vi "Main.vi"() -> ()   [LabVIEW 2013]
doc: "Use this template to build a producer/consumer design pattern with events to produce queue items. Use this design pattern instead of the User Interface Event Handler pattern for user interfaces when you want to execute code asynchronously in response to an event without slowing the user interface responsiveness."
uses:
  ControlLib.llb/state_cntrl.ctl
  ControlLib.llb/main_clstr.ctl
  ControlLib.llb/main_cons_loop_clstr.ctl
  ControlLib.llb/res_range_type_cntrl.ctl
panel:
  out "array":dbl[][](array[numeric])
  out "state_ind":T1=enum."idle" caption="State Status"
  in  "Tab Control":T2(tab)
  in  "initialize":bool caption="Clear All Flags"
  out "stat_oper_resp":string caption="Status Operation Cond Resp"
  in  "stat_oper_cond":bool caption="Check Status Oper Cond"
  in  "trig_dely_auto":bool=TRUE
  in  "trig_delay":dbl caption="Trigger Delay (s)"
  in  "smpl_cnt":u32=1 caption="Sample Count" min=1 max=500000 step=1
  in  "trig_timer_val":dbl caption="Trig Timer Value (s)" max=359999.0 format="%#_2e"
  in  "no_of_trig":u32=1 caption="No of Trigger" max=500000 step=1
  in  "max_trig_cnt":enum16{"Specify Count", "Infinity"}(ring) caption="Max Trig Cnt"
  in  "trig_src":T3(ring)=enum."Immediate" caption="Trigger Source"
  in  "conf_trig":bool caption="Config Trigger"
  out "Error Message":string
  in  "err_qry":bool caption="Error Query"
  in  "fetch_numbers":bool
  in  "byte_count":i32=1024
  out "scan_data":string[](array[string]) caption="Scan Data"
  in  "fetch":bool caption="Fetch Data"
  in  "init":bool caption="Initialize Trigger"
  in  "scan":bool caption="Start Scan"
  in  "range":T4(ring)=enum."Auto" caption="Range"
  in  "res":T5(ring)=enum."6 1/2" caption="Resolution"
  in  "off_comp":bool
  in  "conf_4_wire":bool caption="4 Wire Config"
  in  "open_ch":bool caption="Open Channel"
  in  "chk_ch_state":bool caption="Check channel state?"
  out "ch_state?":string caption="State of the channel"
  in  "VISA resource name":refnum<visa-resource-name>
  in  "close_ch":bool caption="Close Channel"
  in  "ch_string":string caption="Channel or ABUS"
  in  "res_path":path caption="Resistance Path"
  out "res_table":string[][](table) caption="Resistance Table"
  in  "start":bool
  out "text_file":string caption="Data File"
  out "ch_list_str":string caption="Channels Being Scan"
  in  "stop":bool
  # "JPL Automated Multiplexer Safe To Mate - June 2017"
  # "To measure the resistances:\n\n1.  Upload a channel list file.\n2.  Press START to scan.\n3.  The START button will depress\n      itself when the scanning is done."
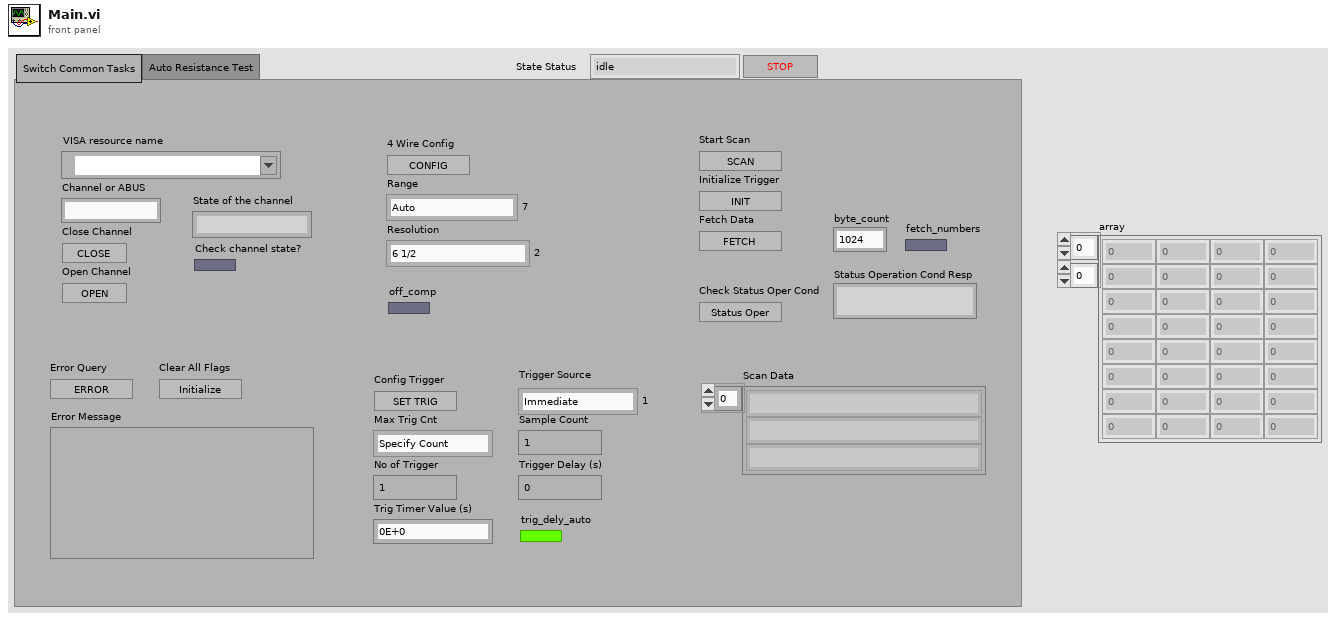
[diagram p1: front panel]
types:
  T1 = typedef "state_cntrl.ctl" = enum16{"initialize", "idle", "read_res_col", "res_val_qry", "plc_ch_in_100_list", "plc_ch_in_1K_list", "plc_ch_in_10K_list", "plc_ch_in_100K_list", "plc_ch_in_1M_list", "plc_ch_in_10M_list", "plc_ch_in_100M_list", "set_100_list_flg", "set_1K_list_flg", "set_10K_list_flg", "set_100K_list_flg", "set_1M_list_flg", "set_10M_list_flg", "set_100M_list_flg", "fin_arry_qry", "chk_100_list_flg", "chk_1K_list_flg", "chk_10K_list_flg", "chk_100K_list_flg", "chk_1M_list_flg", "chk_10M_list_flg", "chk_100M_list_flg", "set_100_ohm_chnl_list", "set_1K_ohm_chnl_list", "set_10K_ohm_chnl_list", "set_100K_ohm_chnl_list", "set_1M_ohm_chnl_list", "set_10M_ohm_chnl_list", "set_100M_ohm_chnl_list", "place_res_in_range", "eof", "det_rnge_to_meas", "set_ch_list", "conf_wire_mode", "conf_trig_type", "start_scan", "scan_cancel_qry", "init_meas", "done_meas_qry", "fetch_data", "fin_test_qry", "fill_data_table", "disp_results"}
  T2 = enum32{"Switch Common Tasks", "Auto Resistance Test"}
  T3 = enum16{"Bus", "Immediate", "External", "Alarm 1", "Alarm 2", "Alarm 3", "Alarm 4", "Timer"}
  T4 = enum16{"100 Ohm", "1 kOhm", "10 kOhm", "100 kOhm", "1 MOhm", "10 MOhm", "100 MOhm", "Auto", "Minimum", "Maximum", "Default"}
  T5 = enum16{"4 1/2", "5 1/2", "6 1/2", "Least", "Highest", "Default"}
  T6 = typedef "main_clstr.ctl" = cluster{"state":T1, "res_col_cnt":i32}
  T7 = typedef "main_cons_loop_clstr.ctl" = cluster{"state":T1, "res_row_cnt":i32, "res_col":dbl[], "res_range_type":T8, "chnl_col":dbl[], "range_setting":bool[], "first_time_set":bool[], "100_list_ch":dbl[], "100_list_row_cnt":i32, "1K_list_ch":dbl[], "1K_list_row_cnt":i32, "10K_list_ch":dbl[], "10K_list_row_cnt":i32, "100K_list_ch":dbl[], "100K_list_row_cnt":i32, "1M_list_ch":dbl[], "1M_list_row_cnt":i32, "10M_list_ch":dbl[], "10M_list_row_cnt":i32, "100M_list_ch":dbl[], "100M_list_row_cnt":i32, "list_flag":bool[], "ch_list_set_cnt":i32, "res_tot_cnt":i32, "slot_col":dbl[], "ch_list_indx_100":i32[], "ch_list_indx_1K":i32[], "ch_list_indx_10K":i32[], "ch_list_indx_100K":i32[], "ch_list_indx_1M":i32[], "ch_list_indx_10M":i32[], "ch_list_indx_100M":i32[], "res_table":dbl[][], "100_ch_list_str":string, "1K_ch_list_str":string, "10K_ch_list_str":string, "100K_ch_list_str":string, "1M_ch_list_str":string, "10M_ch_list_str":string, "100M_ch_list_str":string, "range":enum16{"100 Ohm", "1 kOhm", "10 kOhm", "100 kOhm", "1 MOhm", "10 MOhm", "100 MOhm", "Auto", "Minimum", "Maximum", "Default"}, "resolution":enum16{"4 1/2", "5 1/2", "6 1/2", "Least", "Highest", "Default"}, "scan_data":string[], "res_table_text":string[][]}
  T8 = typedef "res_range_type_cntrl.ctl" = enum16{"100", "1K", "10K", "100K", "1M", "10M", "100M"}
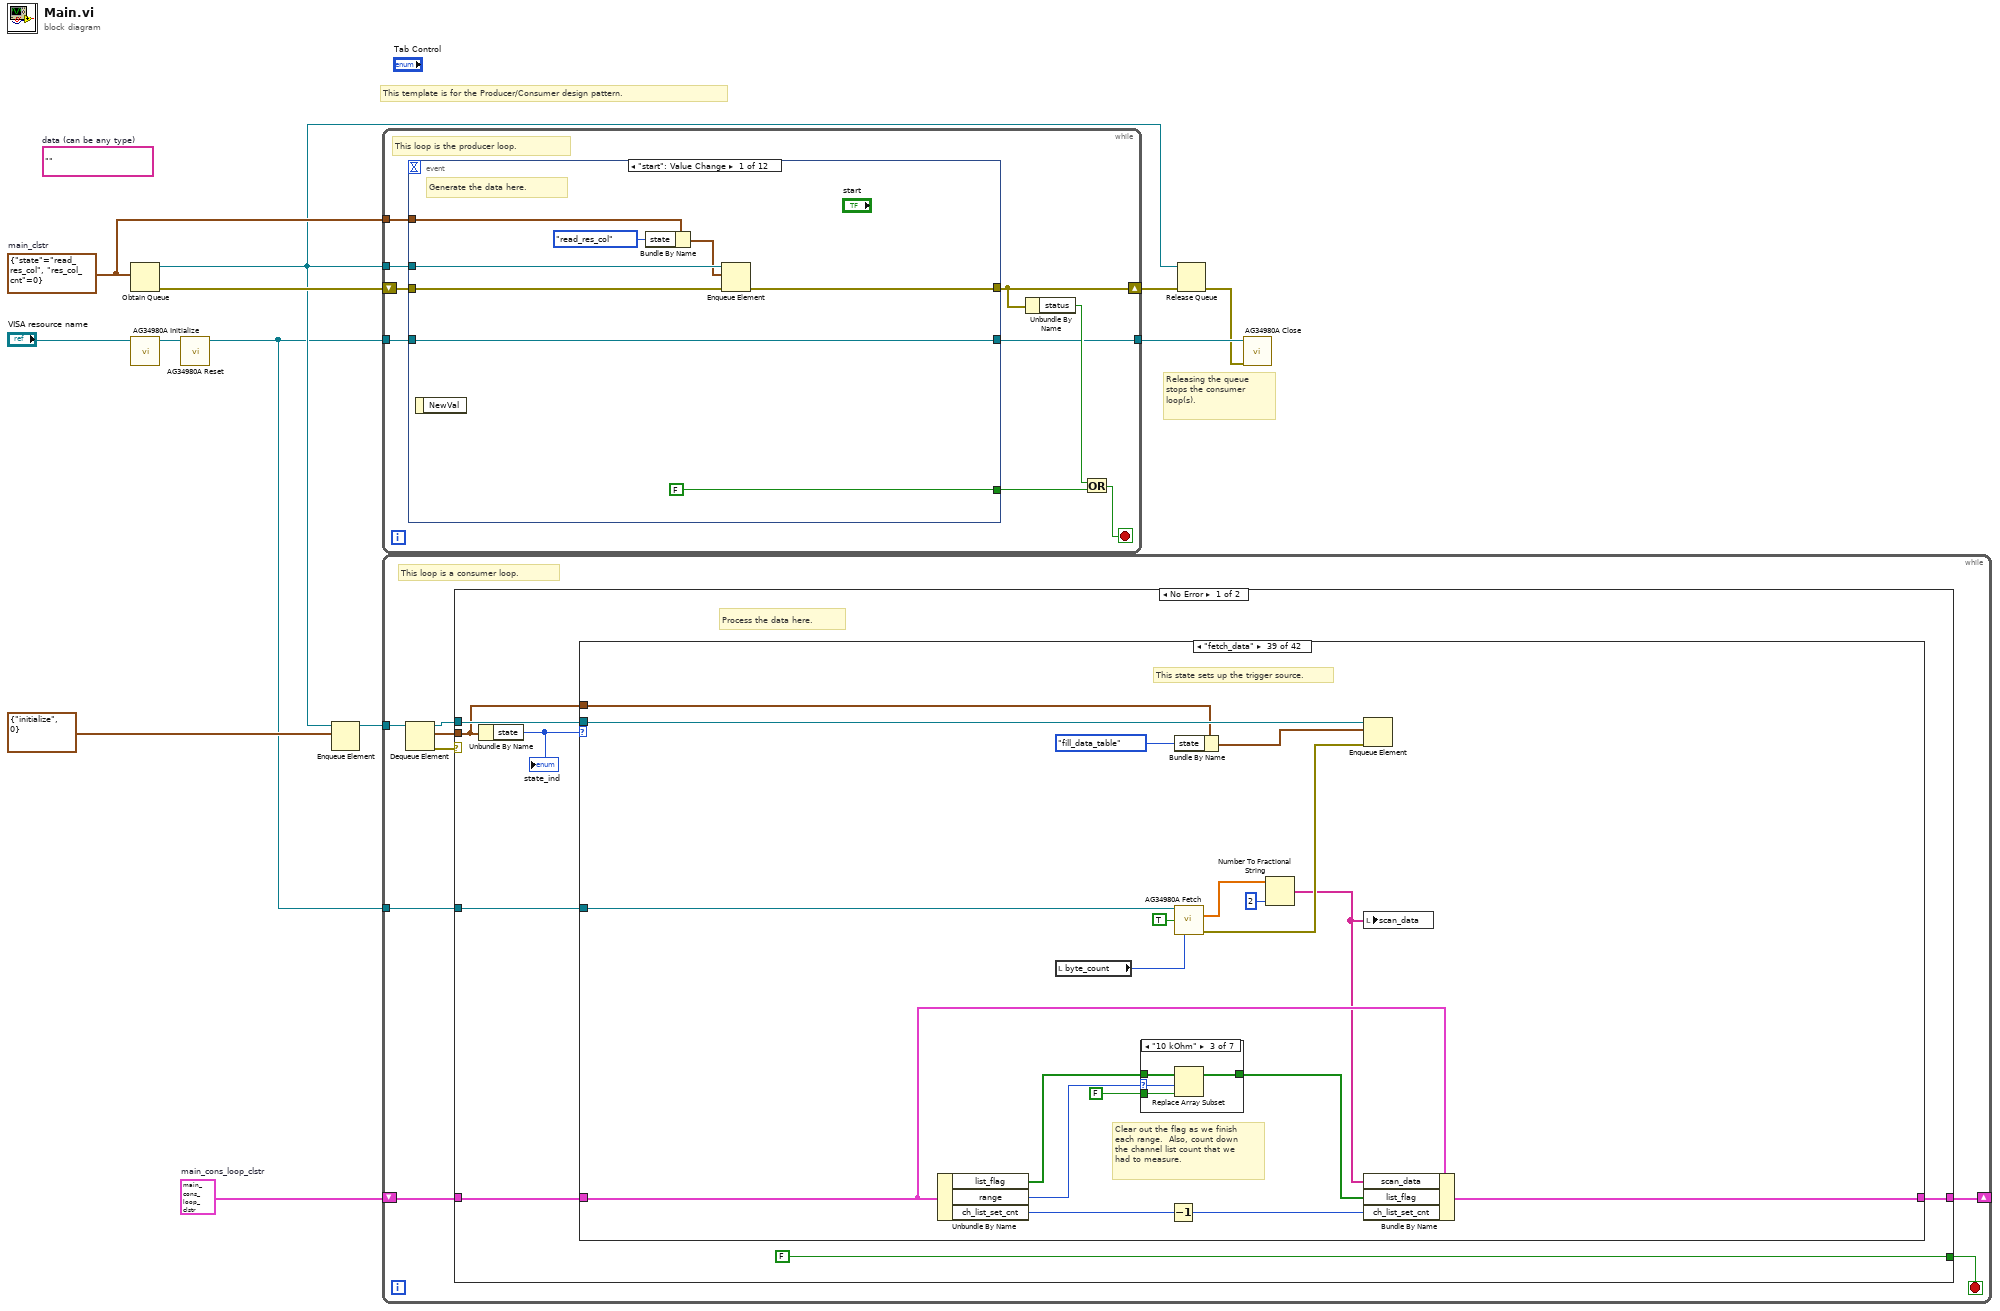
[diagram p0: block diagram]
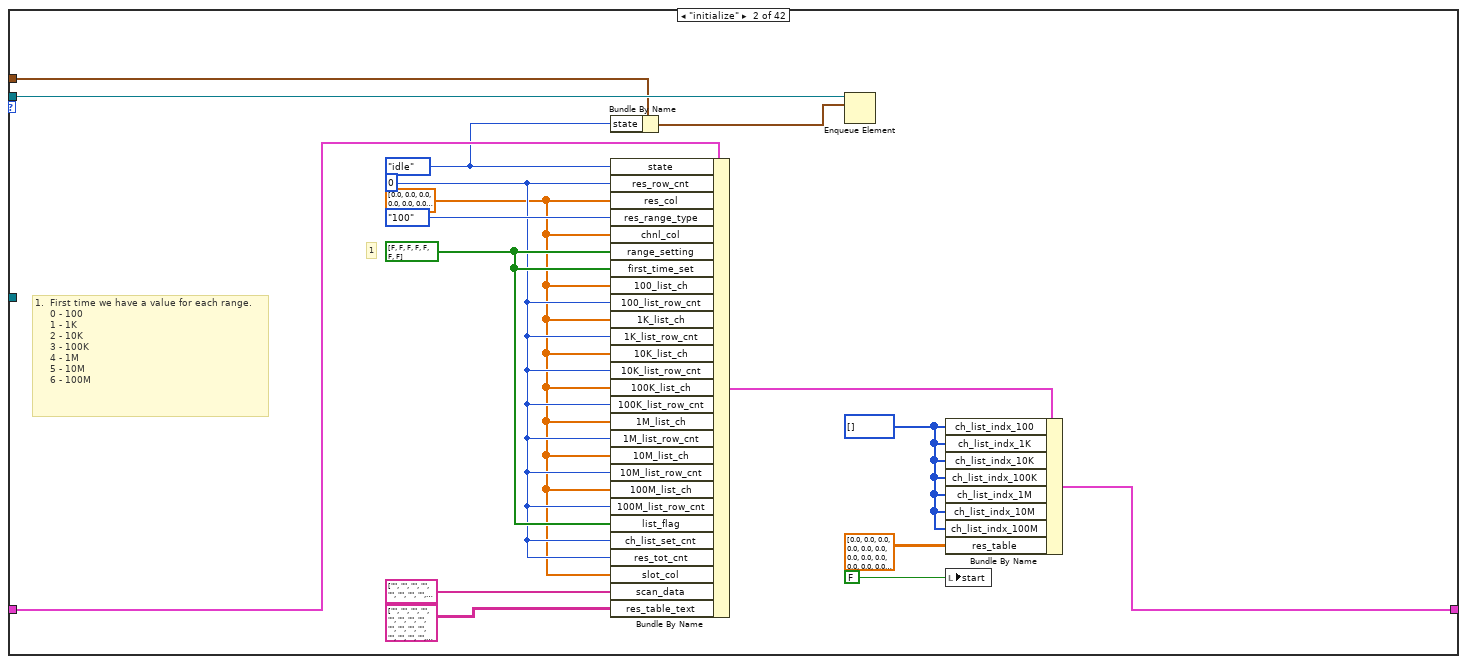
[diagram p3: hidden frame]
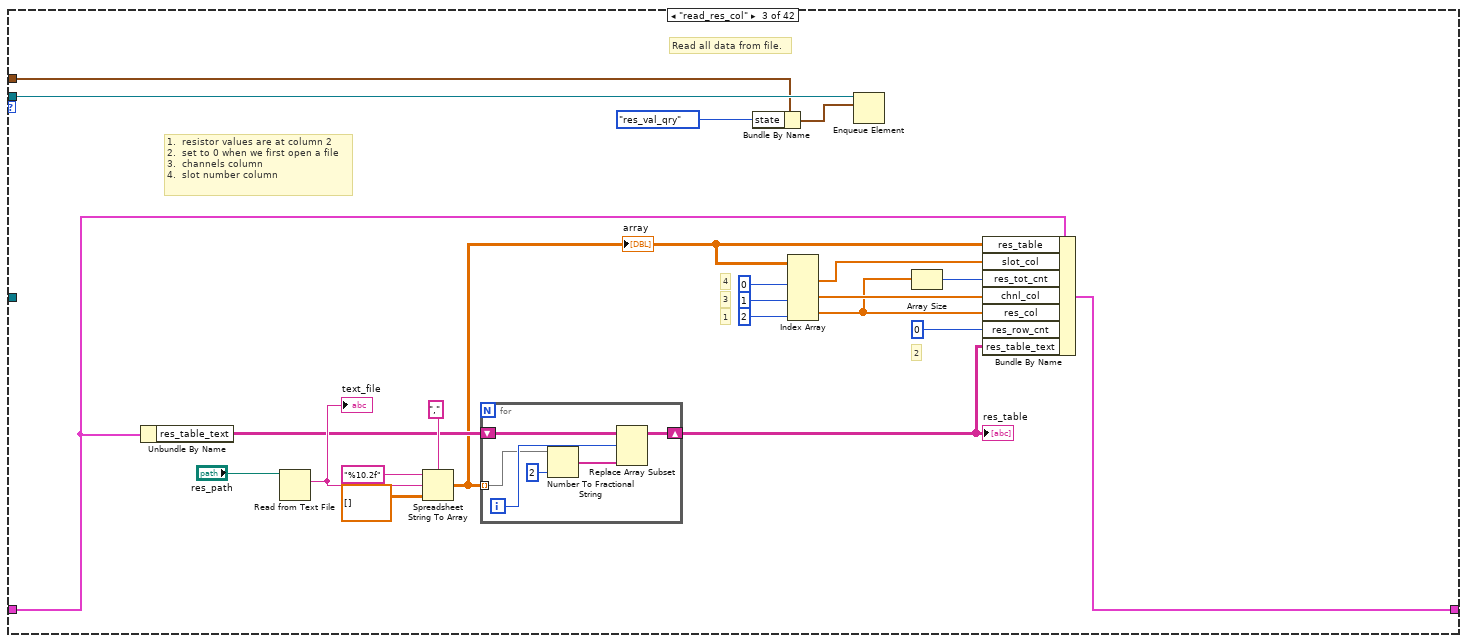
[diagram p4: hidden frame]
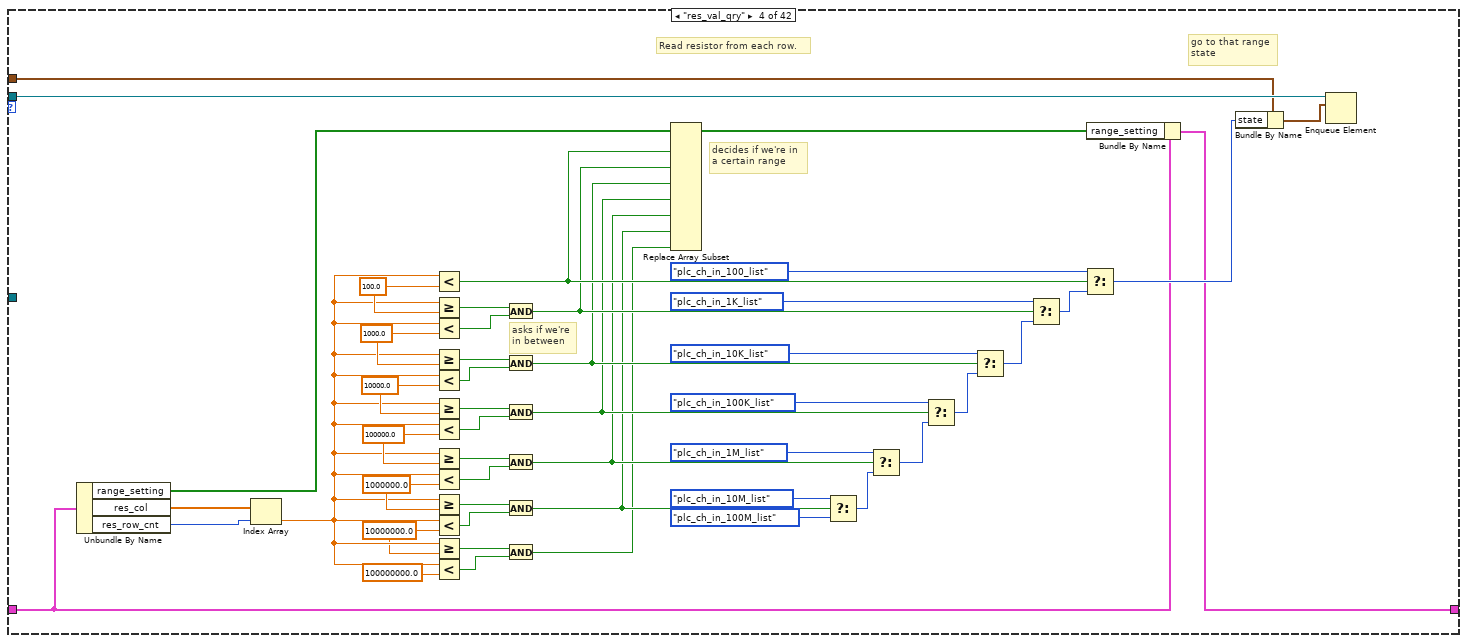
[diagram p5: hidden frame]
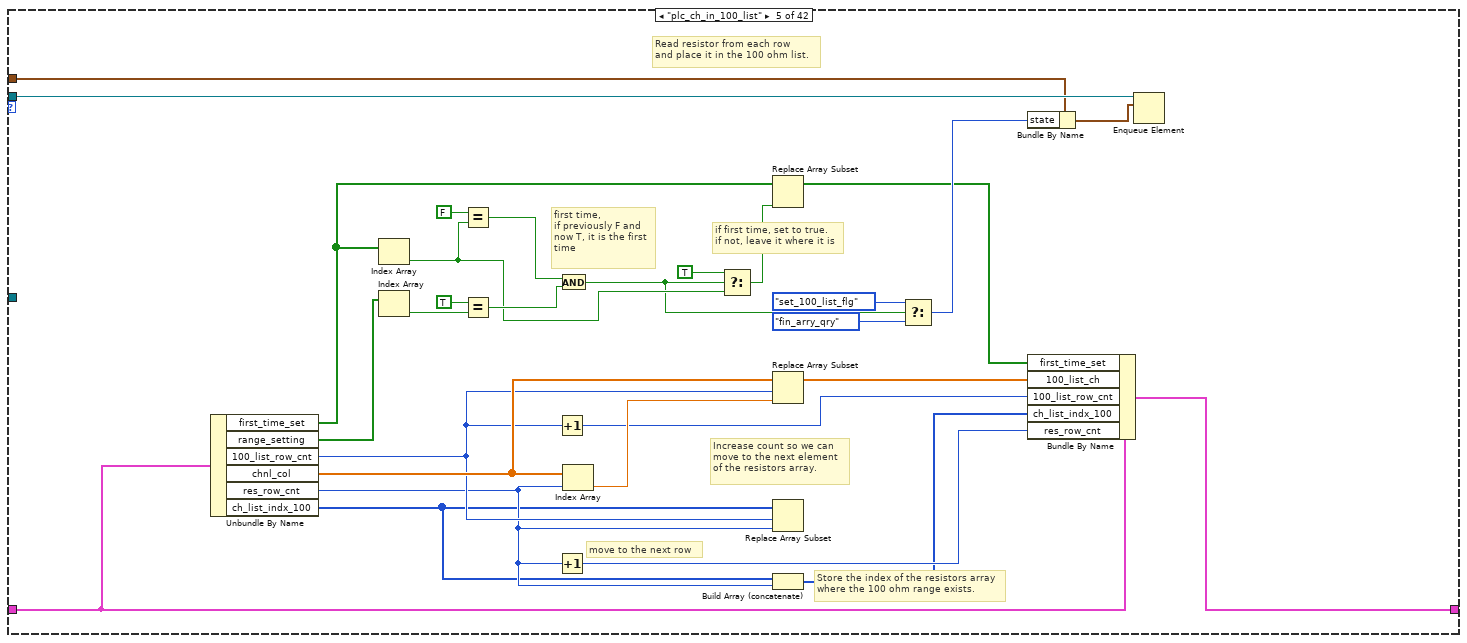
[diagram p6: hidden frame]
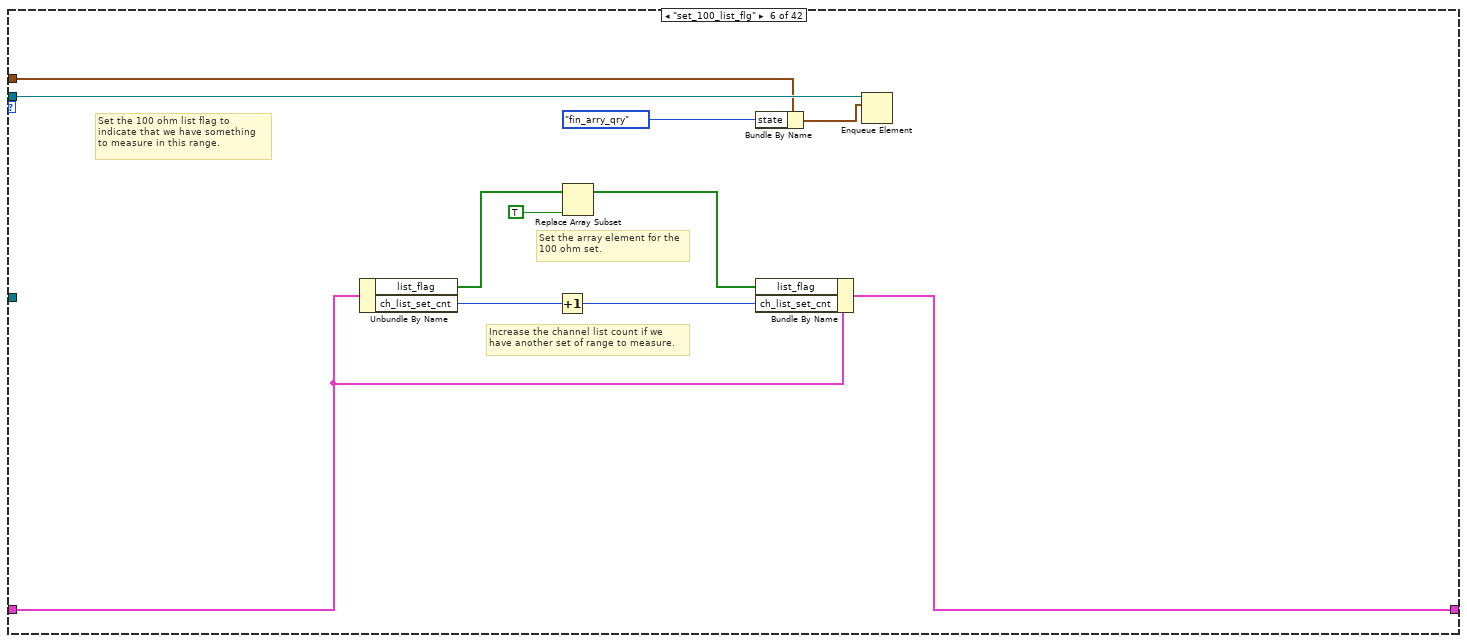
[diagram p7: hidden frame]
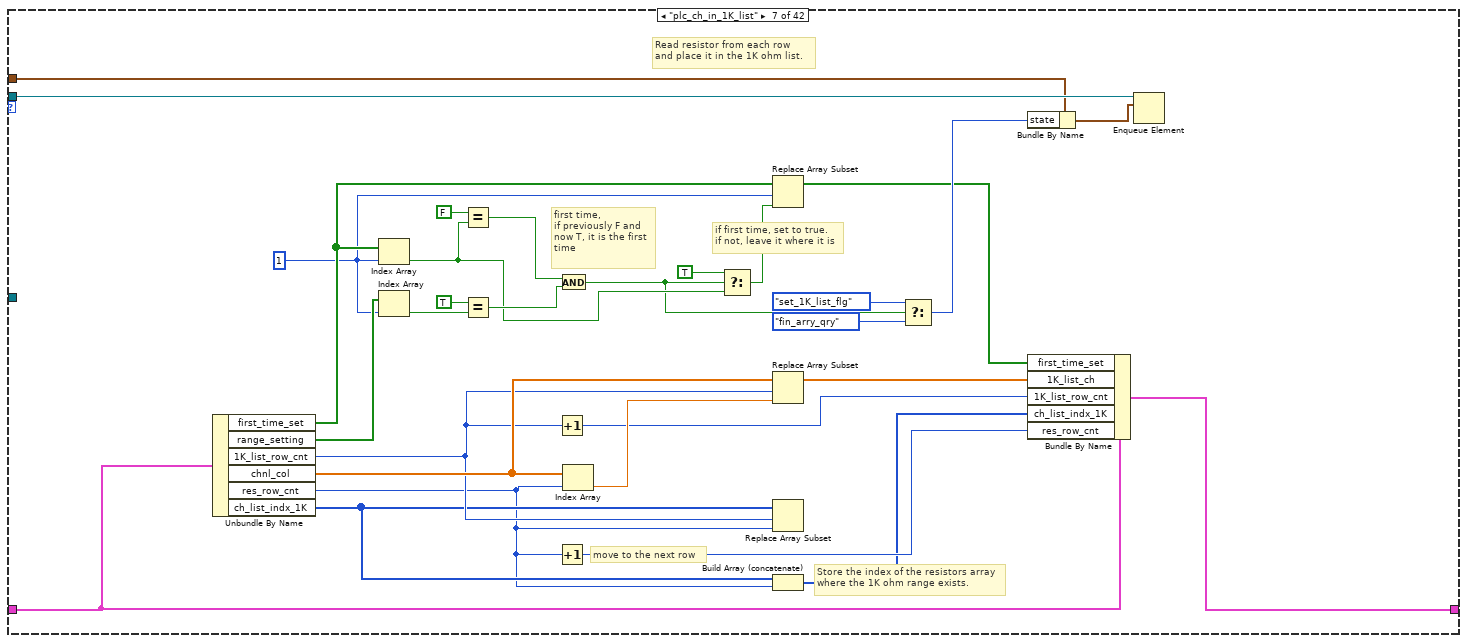
[diagram p8: hidden frame]
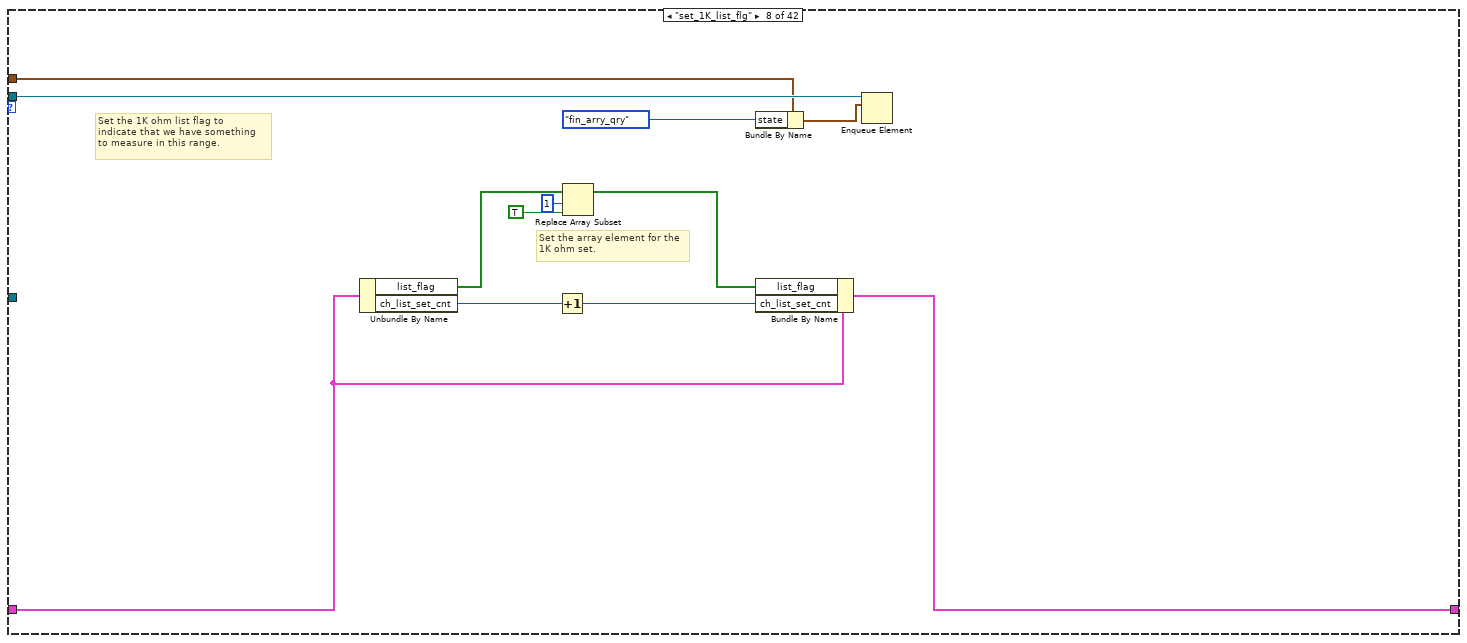
[diagram p9: hidden frame]
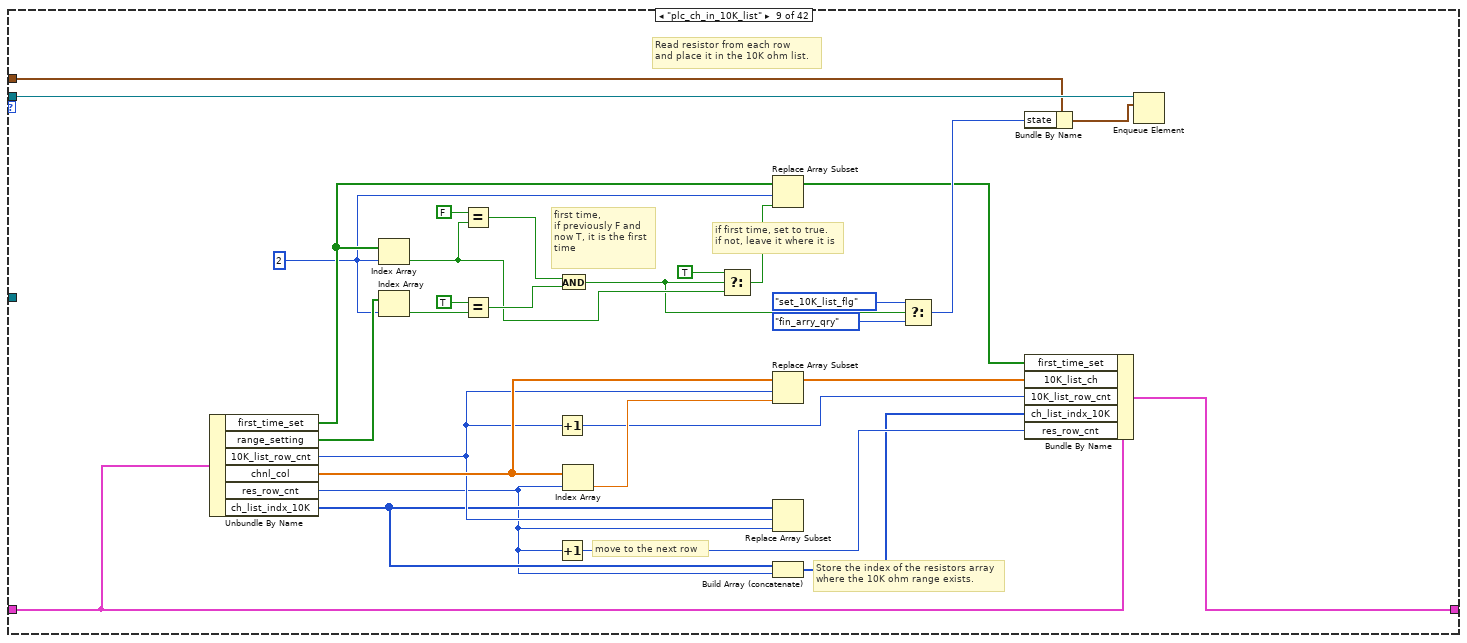
[diagram p10: hidden frame]
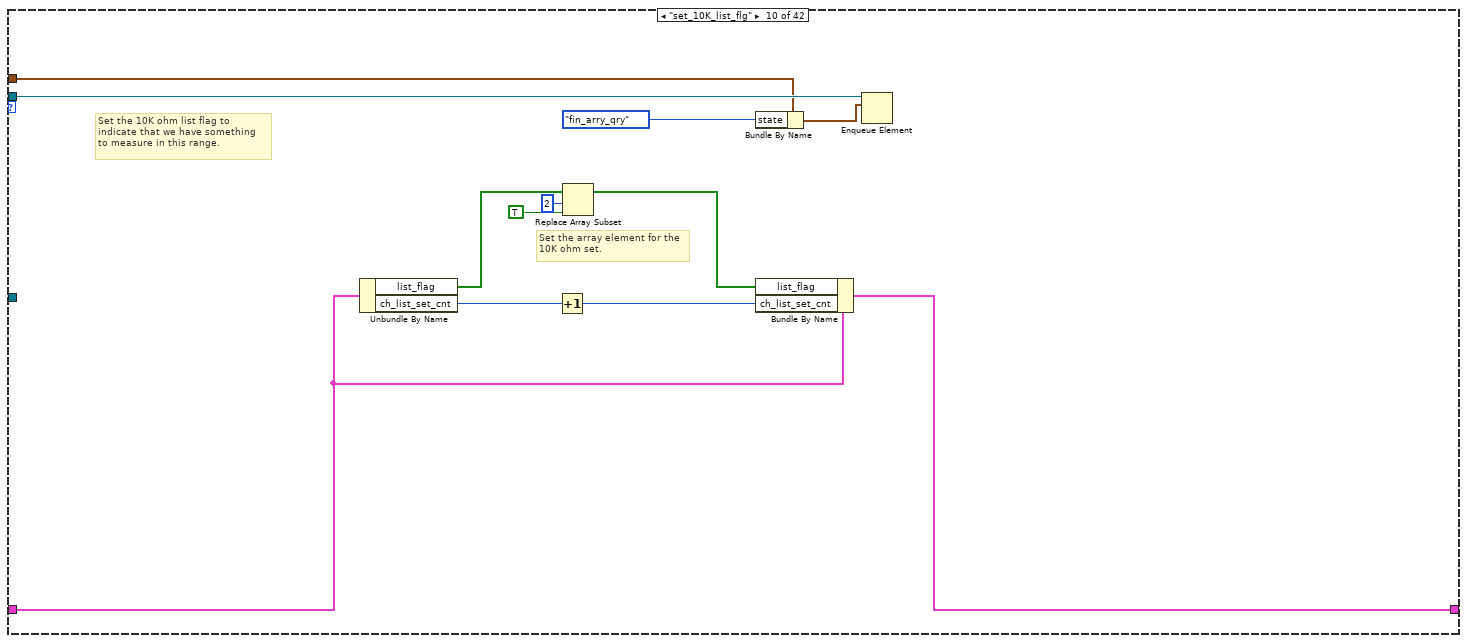
[diagram p11: hidden frame]
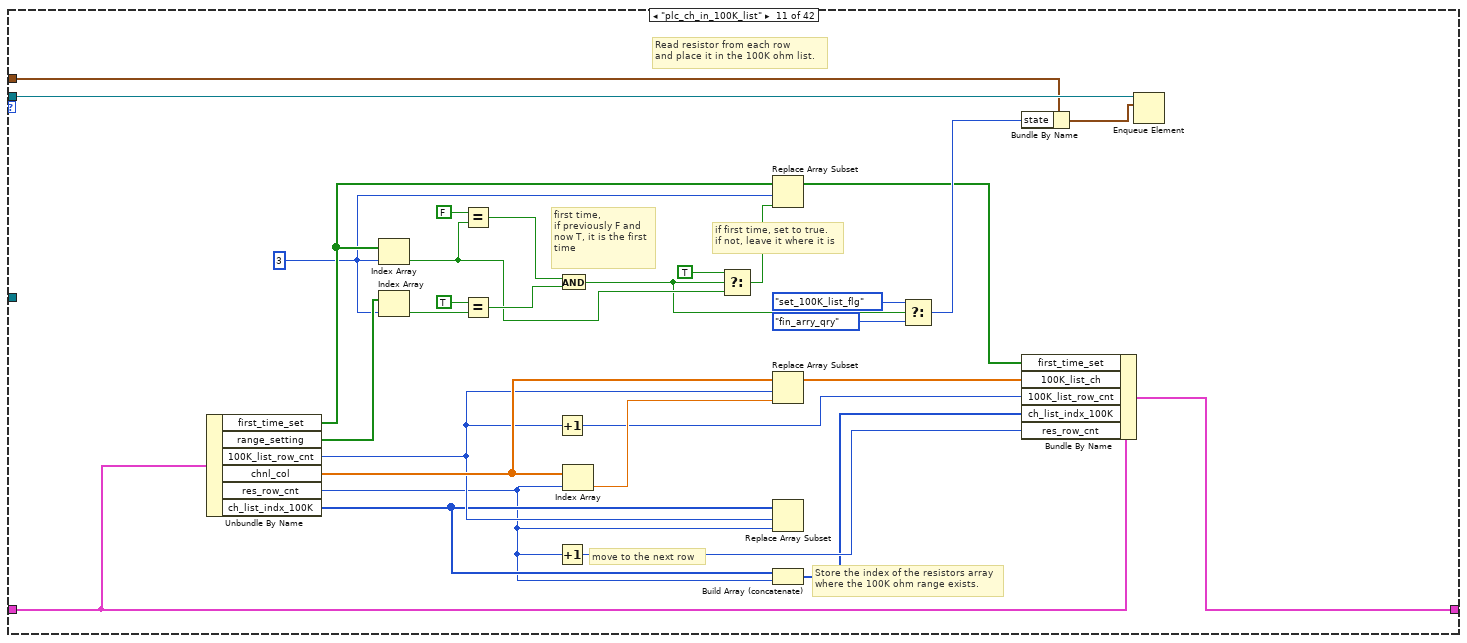
[diagram p12: hidden frame]
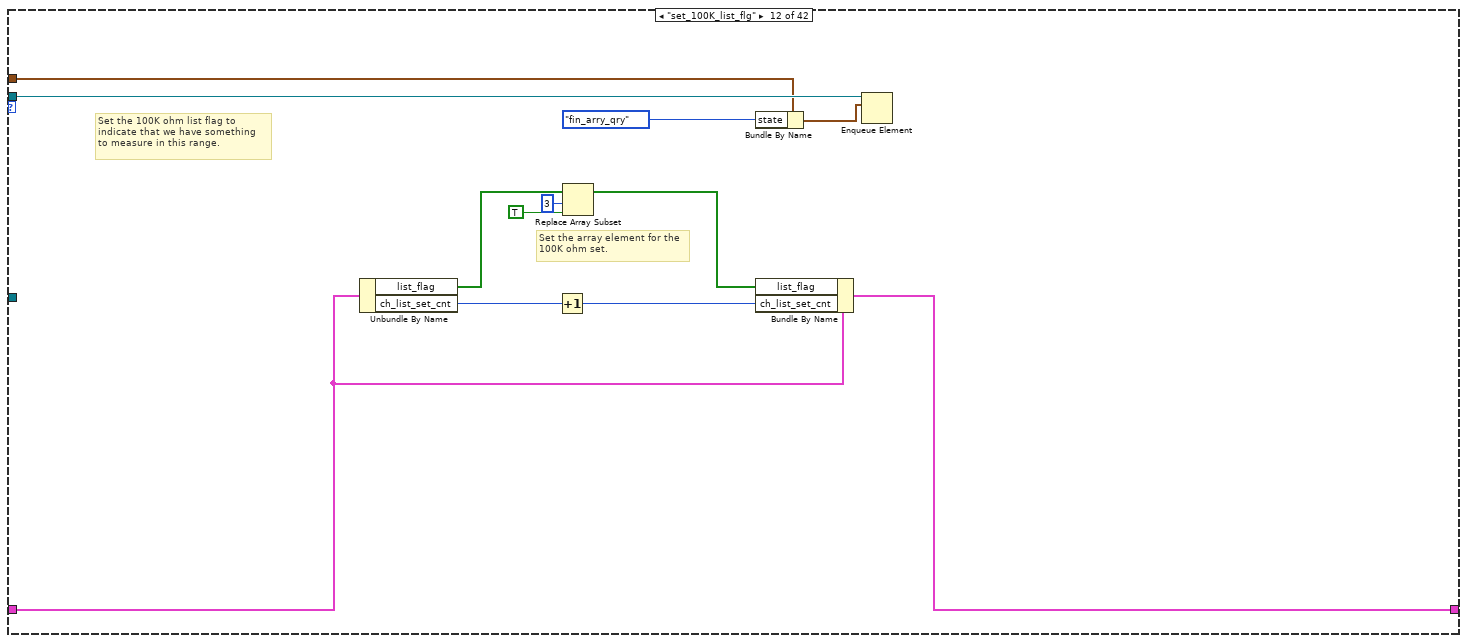
[diagram p13: hidden frame]
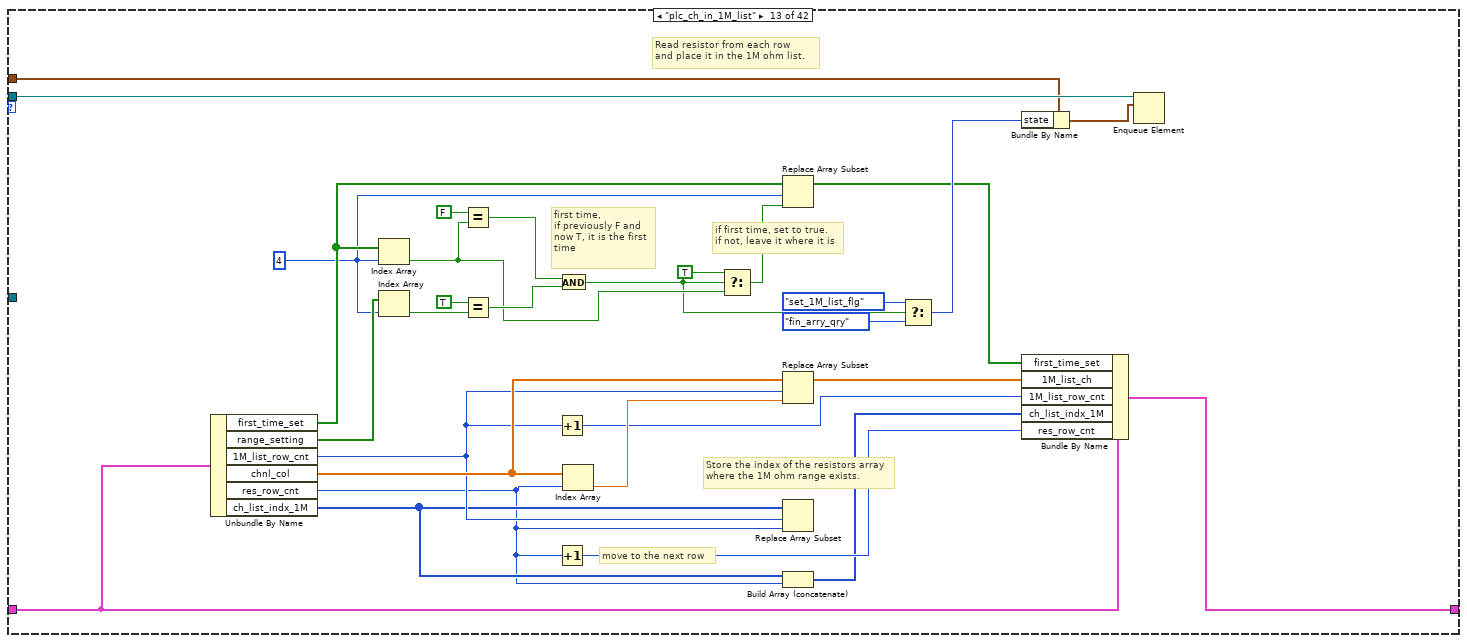
[diagram p14: hidden frame]
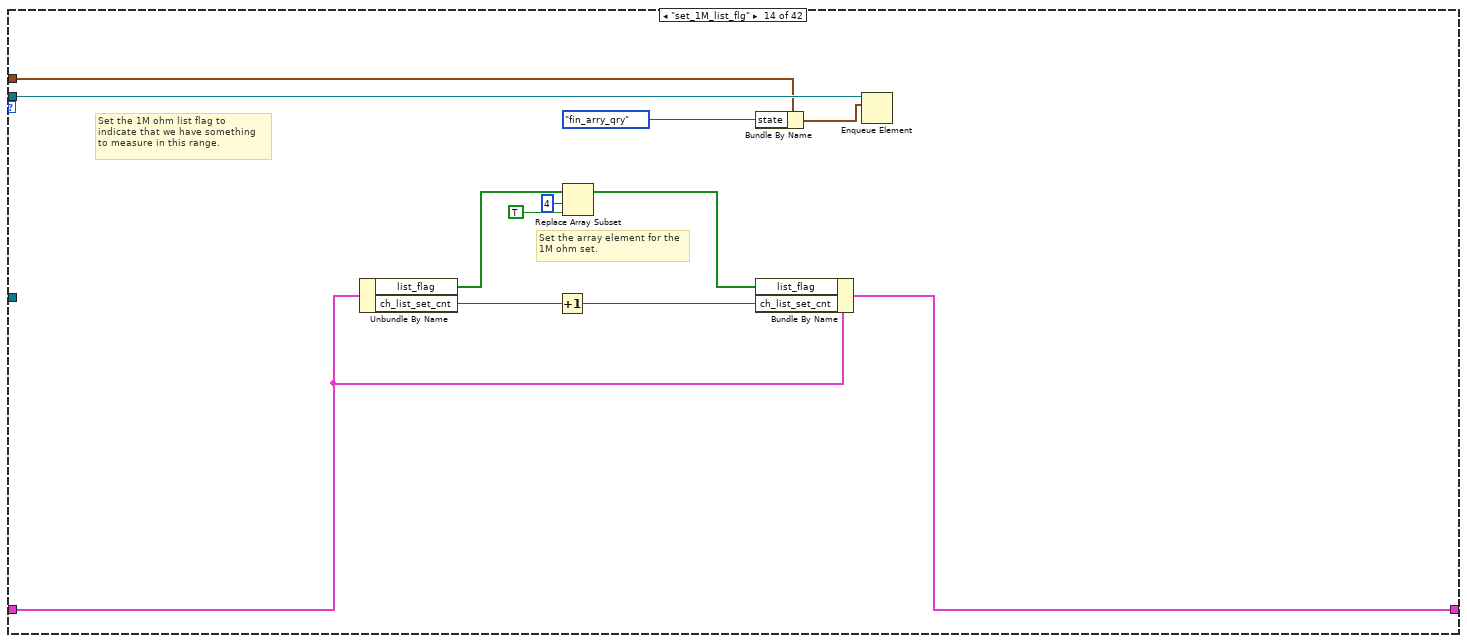
[diagram p15: hidden frame]
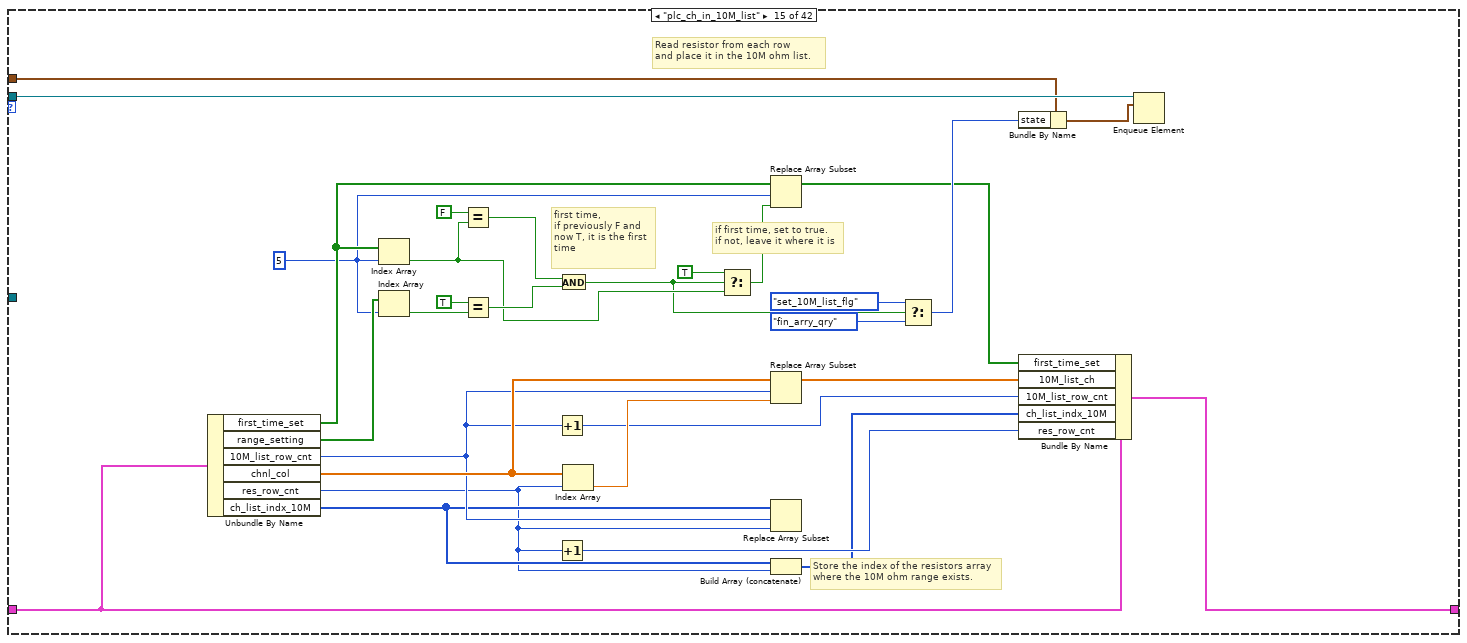
[diagram p16: hidden frame]
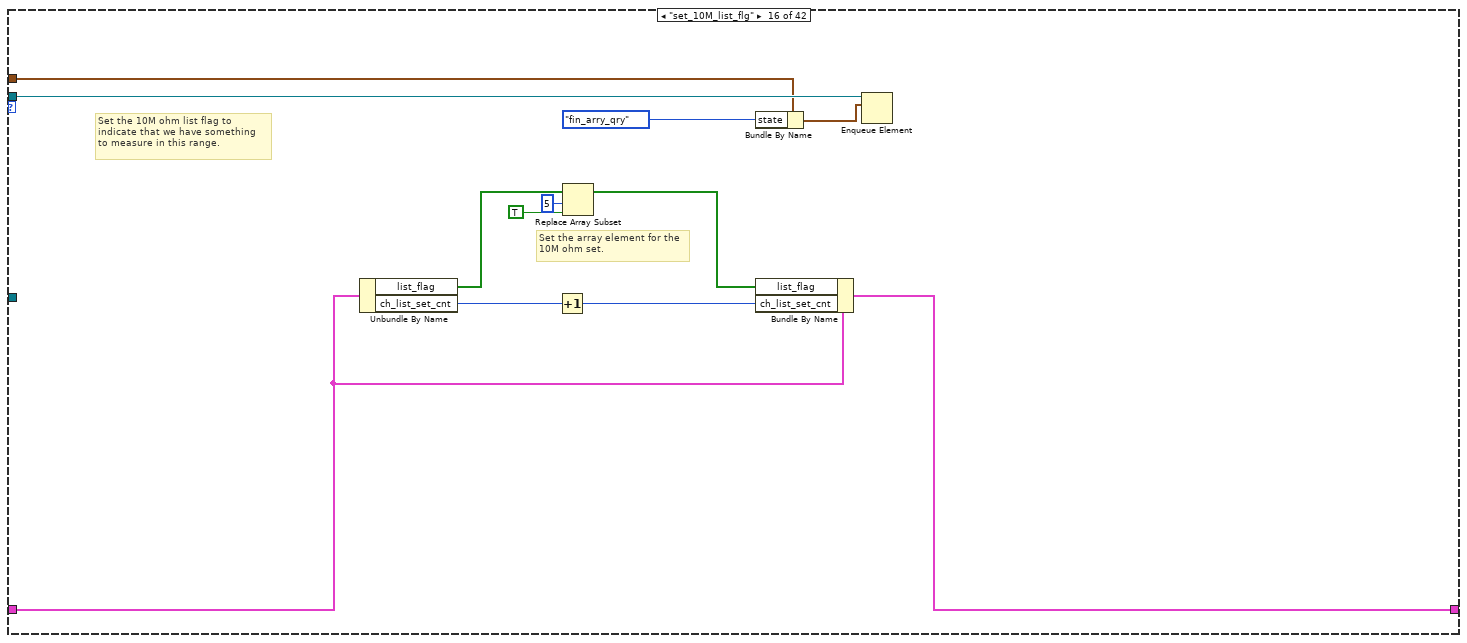
[diagram p17: hidden frame]
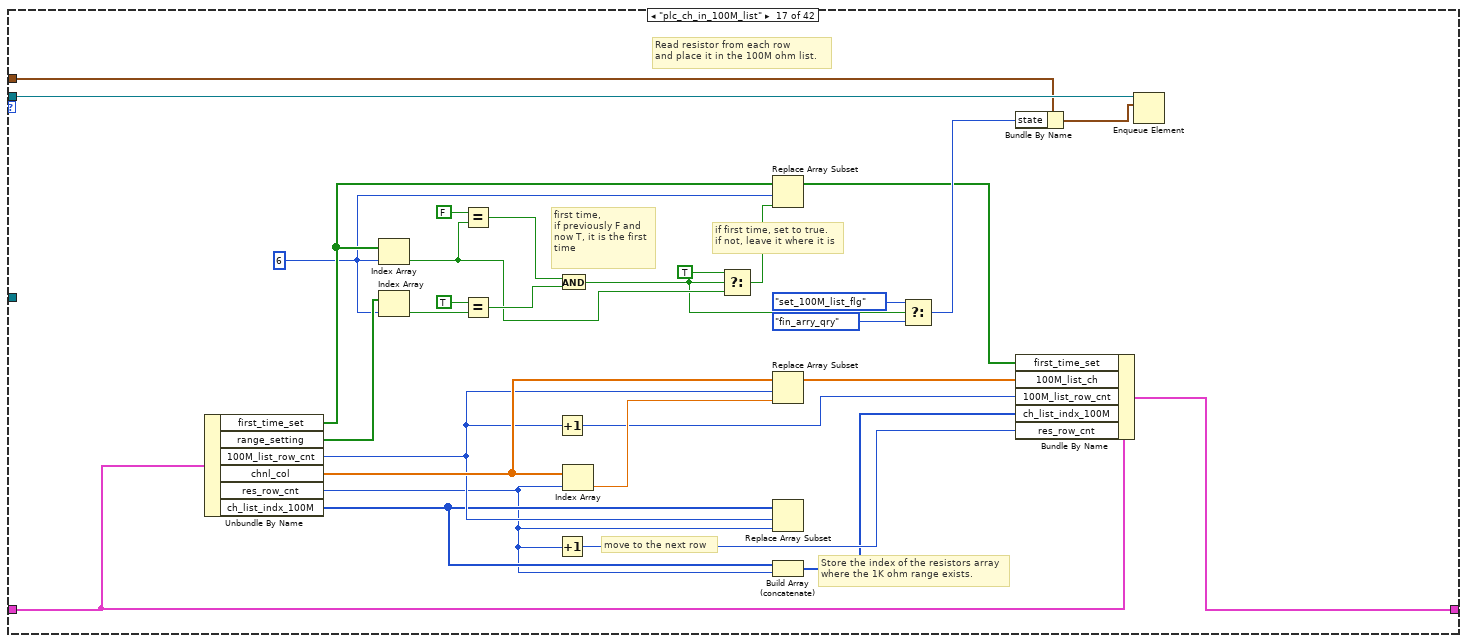
[diagram p18: hidden frame]
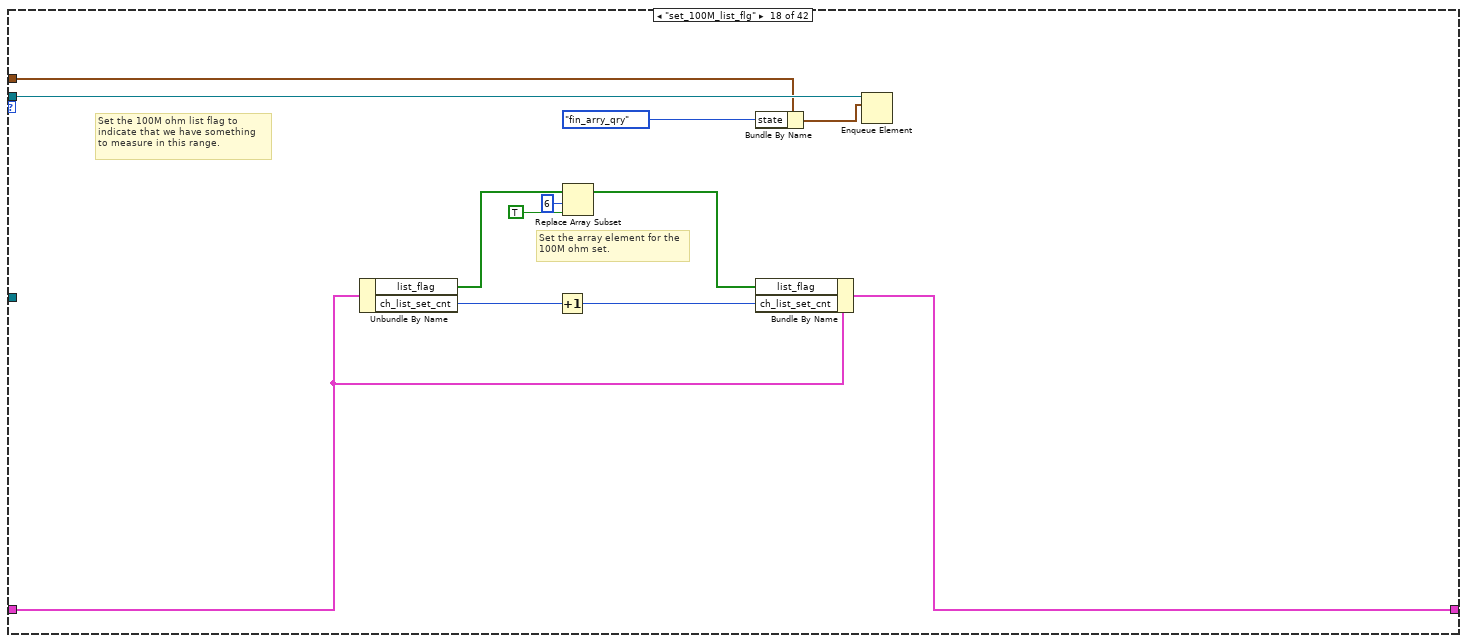
[diagram p19: hidden frame]
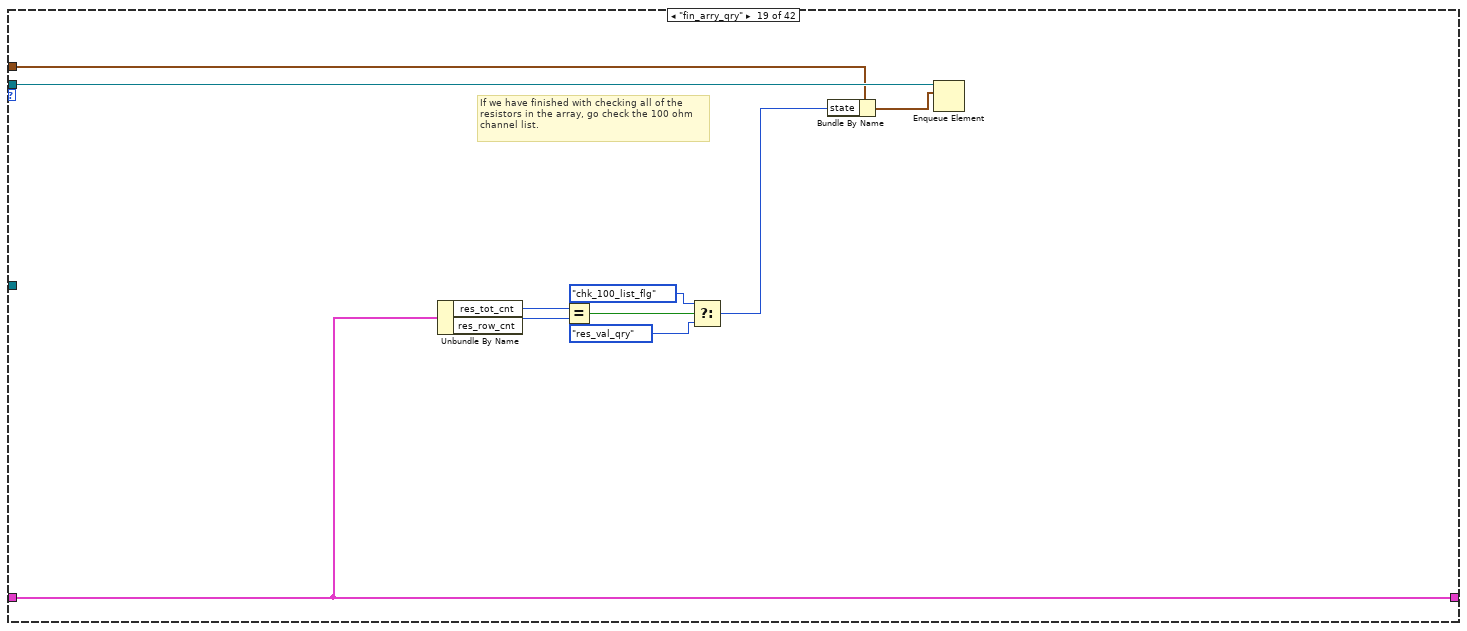
[diagram p20: hidden frame]
diagram:
  w5 = T7 {"state"=enum."read_res_col", "res_row_cnt"=0, "res_col"=[], "res_range_type"=enum."100", "chnl_col"=[], "range_setting"=[], "first_time_set"=[], "100_list_ch"=[], "100_list_row_cnt"=0, "1K_list_ch"=[], "1K_list_row_cnt"=0, "10K_list_ch"=[], "10K_list_row_cnt"=0, "100K_list_ch"=[], "100K_list_row_cnt"=0, "1M_list_ch"=[], "1M_list_row_cnt"=0, "10M_list_ch"=[], "10M_list_row_cnt"=0, "100M_list_ch"=[], "100M_list_row_cnt"=0, "list_flag"=[], "ch_list_set_cnt"=0, "res_tot_cnt"=0, "slot_col"=[], "ch_list_indx_100"=[], "ch_list_indx_1K"=[], "ch_list_indx_10K"=[], "ch_list_indx_100K"=[], "ch_list_indx_1M"=[], "ch_list_indx_10M"=[], "ch_list_indx_100M"=[], "res_table"=[], "100_ch_list_str"="", "1K_ch_list_str"="", "10K_ch_list_str"="", "100K_ch_list_str"="", "1M_ch_list_str"="", "10M_ch_list_str"="", "100M_ch_list_str"="", "range"=enum."100 Ohm", "resolution"=enum."4 1/2", "scan_data"=[], "res_table_text"=[]}  # main_cons_loop_clstr
  w6 = T6 {"state"=enum."read_res_col", "res_col_cnt"=0}  # main_clstr
  (unwired) ""  # data (can be any type)
  # "Releasing the queue stops the consumer loop(s)."
  # "This template is for the Producer/Consumer design pattern."
  n1 = Obtain Queue(element data type=w6) -> (queue out=w4:refnum<queue>, error out=w12:errorcluster)  [unwired: 4 in, 1 out]
  n2 = call <instrlib>:"AG34980A Initialize.vi"("VISA resource name"="VISA resource name") -> ("VISA session"=w9:refnum<visa-resource-name>)  [unwired: 13 in, 1 out]
  n3 = call <instrlib>:"AG34980A Reset.vi"("VISA resource name"=w9) -> ("VISA resource name out"=w1:refnum<visa-resource-name>)  [unwired: 13 in, 1 out]
  n4 = Enqueue Element(queue=w4, element=T6 {"state"=enum."initialize", "res_col_cnt"=0}) -> (queue out=w3:refnum<queue>)  [unwired: 2 in, 2 out]
  n5 = while {
    shift-right: [w18] -> w11
    shift-left: w12 -> [w20]
    tunnel: w4 -> [w21]
    tunnel: w1 -> [w16]
    tunnel: [w15] -> w8
    tunnel: w6 -> [w13]
    stop <- w14 stop-if-true
    # "This loop is the producer loop."
    n6 = event shown="[0] \"start\": Value Change" {
      selector: _ -> [_ _ _ _ _ _ _ _ _ _ _ _]
      dyn-events: _ -> [_ _ _ _ _ _ _ _ _ _ _ _]
      timeout: _ -> [_ _ _ _ _ _ _ _ _ _ _ _]
      tunnel: w21 -> [w29 w37 _ _ _ _ _ _ _ _ _ _]
      tunnel: w20 -> [w28 w36 w38 w46 w52 w57 w77 w88 w93 w97 w105 w110]
      tunnel: [w27 w35 w38 w46 w52 w57 w77 w88 w93 w97 w105 w110] -> w18
      tunnel: [FALSE ("stop") FALSE ("stop") FALSE ("stop") FALSE ("stop") FALSE ("stop") FALSE ("stop") FALSE ("stop") FALSE ("stop") FALSE ("stop") FALSE ("stop") FALSE ("stop") "stop"] -> w19
      tunnel: w16 -> [w25 w33 w44 w50 w55 w63 w86 w91 w95 w102 w107 w109]
      tunnel: [w25 w33 w39 w47 w54 w61 w85 w89 w94 w101 w106 w109] -> w15
      tunnel: w13 -> [w24 w32 _ _ _ _ _ _ _ _ _ _]
      event "start": Value Change {
        # "Generate the data here."
        n7 = event-data() -> ()  [unwired: 1 in, 1 out]
        n8 = Bundle By Name(cluster=w24, "state"=state_cntrl."read_res_col") -> (w22:T6)
        n9 = Enqueue Element(queue=w29, element=w22, error in (no error)=w28) -> (error out=w27:errorcluster)  [unwired: 1 in, 2 out]
      }
      event "initialize": Value Change {
        # "Generate the data here."
        n10 = event-data() -> ()  [unwired: 1 in, 1 out]
        n11 = Bundle By Name(cluster=w32, "state"=state_cntrl."initialize") -> (w30:T6)
        n12 = Enqueue Element(queue=w37, element=w30, error in (no error)=w36) -> (error out=w35:errorcluster)  [unwired: 1 in, 2 out]
      }
      event "close_ch": Value Change {
        n13 = event-data() -> ()  [unwired: 1 in, 1 out]
        n14 = call <instrlib>:"AG34980A Switch.vi"("VISA resource name"=w44, "Channel List"="ch_string", "Open/Close (0:Close)"=enum16{"Close", "Open"}."Close", "Set/Check (F:Set)"="chk_ch_state") -> ("VISA resource name out"=w39:refnum<visa-resource-name>, "Channel State?"=→"ch_state?":string)  [unwired: 9 in, 1 out]
      }
      event "open_ch": Value Change {
        n15 = event-data() -> ()  [unwired: 1 in, 1 out]
        n16 = local read "ch_string"() -> (w48:string)
        n17 = call <instrlib>:"AG34980A Switch.vi"("VISA resource name"=w50, "Channel List"=w48, "Open/Close (0:Close)"=enum16{"Close", "Open"}."Open") -> ("VISA resource name out"=w47:refnum<visa-resource-name>)  [unwired: 10 in, 2 out]
      }
      event "err_qry": Value Change {
        n18 = event-data() -> ()  [unwired: 1 in, 1 out]
        n19 = call <instrlib>:"AG34980A Error Query.vi"("VISA resource name"=w55) -> ("VISA resource name out"=w54:refnum<visa-resource-name>, "Error Message"=→"Error Message":string)  [unwired: 11 in, 2 out]
      }
      event "conf_4_wire": Value Change {
        n20 = event-data() -> ()  [unwired: 1 in, 1 out]
        n21 = local read "ch_string"() -> (w62:string)
        n22 = disable-structure shown="Enabled" {
          disable-tunnel: w63 -> [w70 w75]
          disable-tunnel: w62 -> [w69 w74]
          disable-tunnel: [w68 w76] -> w61
          disable-tunnel: "range" -> [w67 w73]
          disable-tunnel: "res" -> [w66 w72]
          disable-tunnel: "off_comp" -> [w65 w71]
          frame Enabled {
            n23 = call <instrlib>:"AG34980A Configure 4-Wire Resistance.vi"("VISA resource name"=w70, "Channel List(empty)"=w69, "Range (7:Auto)"=w67, "Resolution (5:Default)"=w66, "Offset Compensation (F:Off)"=w65) -> ("VISA resource name out"=w68:refnum<visa-resource-name>)  [unwired: 9 in, 1 out]
          }
          frame Disabled {
            n24 = call "AG34980A_Configure_4_Wire_Resistance.vi"("VISA resource name"=w75, "Channel List(empty)"=w74, "Range (7:Auto)"=w73, "Resolution (5:Default)"=w72, "Offset Compensation (F:Off)"=w71) -> ("VISA resource name out"=w76:refnum<visa-resource-name>)  [unwired: 9 in, 1 out]
          }
        }
      }
      event "conf_trig": Value Change {
        n25 = event-data() -> ()  [unwired: 1 in, 1 out]
        n26 = call <instrlib>:"AG34980A Configure Trigger.vi"("VISA resource name"=w86, "Trigger Timer Value (0 sec)"="trig_timer_val", "Sample Count (1)"="smpl_cnt", "Trigger Source (1:Immediate)"="trig_src", "Max Trigger Count (0:Specify Count)"="max_trig_cnt", "# Triggers (1)"="no_of_trig", "Trigger Delay (0 sec)"="trig_delay", "Trigger Delay Auto? (T:On)"="trig_dely_auto") -> ("VISA resource name out"=w85:refnum<visa-resource-name>)  [unwired: 6 in, 1 out]
      }
      event "scan": Value Change {
        n27 = event-data() -> ()  [unwired: 1 in, 1 out]
        n28 = local read "ch_string"() -> (w90:string)
        n29 = call <instrlib>:"AG34980A Configure Scan.vi"("VISA resource name"=w91, "Scan List(empty)"=w90) -> ("VISA resource name out"=w89:refnum<visa-resource-name>)  [unwired: 12 in, 1 out]
      }
      event "init": Value Change {
        n30 = event-data() -> ()  [unwired: 1 in, 1 out]
        n31 = call <instrlib>:"AG34980A Initiate.vi"("VISA resource name"=w95) -> ("VISA resource name out"=w94:refnum<visa-resource-name>)  [unwired: 13 in, 1 out]
      }
      event "fetch": Value Change {
        n32 = event-data() -> ()  [unwired: 1 in, 1 out]
        n33 = call <instrlib>:"AG34980A Fetch.vi"("VISA resource name"=w102, "Numbers Only (T:On)"="fetch_numbers", "Byte Count (1024 bytes)"="byte_count") -> ("VISA resource name out"=w101:refnum<visa-resource-name>, "Output Data"=→"scan_data":string[])  [unwired: 9 in, 2 out]
      }
      event "stat_oper_cond": Value Change {
        n34 = event-data() -> ()  [unwired: 1 in, 1 out]
        n35 = call "AG34980A_Status_Oper_Cond.vi"("VISA resource name"=w107) -> ("VISA resource name out"=w106:refnum<visa-resource-name>, "resp"=→"stat_oper_resp":string)  [unwired: 12 in, 1 out]
      }
      event "stop": Value Change {
        n36 = event-data() -> ()  [unwired: 1 in, 1 out]
      }
    }
    n37 = Unbundle By Name(w18) -> ("status"=w17:bool)
    n38 = Or(x=w17, y=w19) -> (x .or. y?=w14:bool)
  }
  n39 = while {
    tunnel: w3 -> [w119]
    shift-right: [w114] -> _
    shift-left: w5 -> [w115]
    tunnel: w1 -> [w112]
    stop <- w113 stop-if-true
    # "This loop is a consumer loop."
    n40 = Dequeue Element(queue=w119) -> (queue out=w116:refnum<queue>, element=w117:T6, error out=w118:errorcluster)  [unwired: 2 in, 1 out]
    n41 = case shown="No Error" w118 {
      tunnel: w117 -> [w123 _]
      tunnel: [FALSE TRUE] -> w113
      tunnel: w116 -> [w124 _]
      tunnel: w115 -> [w122 w3308]
      tunnel: [w121 w3308] -> w114
      tunnel: w112 -> [w120 _]
      frame No Error {
        # "Process the data here."
        n42 = Unbundle By Name(w123) -> ("state"=w125:T1)
        "state_ind" <- w125
        n43 = case shown="\"fetch_data\"" w125 {
          tunnel: w124 -> [_ w134 w161 w220 w249 w260 w290 w302 w332 w344 w374 w386 w416 w428 w458 w470 w500 w512 w522 w531 w541 w551 w561 w571 w581 w592 w624 w656 w688 w720 w752 w784 w823 w831 w848 w856 w863 w870 w902 w947 w3296 w3307]
          tunnel: w123 -> [_ w132 w160 w218 w247 w258 w288 w300 w330 w342 w372 w384 w414 w426 w456 w468 w498 w510 w520 w529 w539 w549 w559 w569 w579 w590 w622 w654 w686 w718 w750 w782 w821 w829 w846 w854 w861 w868 w900 w945 w3294 w3303]
          tunnel: w122 -> [w127 w143 w147 w172 w246 w257 w287 w299 w329 w341 w371 w383 w413 w425 w455 w467 w497 w509 w513 w525 w535 w545 w555 w565 w575 w585 w617 w649 w681 w713 w745 w777 w807 w826 w833 w853 w858 w865 w893 w933 w3292 w3299]
          tunnel: [w127 w137 w155 w201 w241 w254 w282 w296 w324 w338 w366 w380 w408 w422 w450 w464 w492 w506 w513 w525 w535 w545 w555 w565 w575 w583 w616 w648 w680 w712 w744 w776 w807 w826 w833 w853 w858 w865 w892 w932 w3292 w3297] -> w121
          tunnel: w120 -> [_ _ _ _ _ _ _ _ _ _ _ _ _ _ _ _ _ _ _ _ _ _ _ _ _ _ _ _ _ _ _ _ w819 w827 w844 _ w859 w866 w898 _ _ _]
          frame "idle", Default {
          }
          frame "initialize" {
            w135 = i32[] [] ("ch_list_indx_100")
            w133 = state_cntrl."idle" ("state")
            w140 = 0 ("100_list_row_cnt")
            w139 = dbl[] [0.0, 0.0, 0.0, 0.0, 0.0, 0.0, 0.0, 0.0, 0.0, 0.0, 0.0, 0.0, 0.0, 0.0, 0.0, 0.0, 0.0, 0.0, 0.0, 0.0, 0.0, 0.0, 0.0, 0.0, 0.0, 0.0, 0.0, 0.0, 0.0, 0.0, 0.0, 0.0, 0.0, 0.0, 0.0, 0.0, 0.0, 0.0, 0.0, 0.0, 0.0, 0.0, 0.0, 0.0, 0.0, 0.0, 0.0, 0.0, 0.0, 0.0, 0.0, 0.0, 0.0, 0.0, 0.0, 0.0, 0.0, 0.0, 0.0, 0.0, 0.0, 0.0, 0.0, 0.0, 0.0, 0.0, 0.0, 0.0, 0.0] ("100_list_ch")
            w141 = bool[] [FALSE, FALSE, FALSE, FALSE, FALSE, FALSE, FALSE] ("first_time_val")
            # "1.  First time we have a value for each range.\n     0 - 100\n     1 - 1K\n     2 - 10K\n     3 - 100K\n     4 - 1M\n     5 - 10M\n     6 - 100M"
            # "1"
            n44 = Bundle By Name(cluster=w132, "state"=w133) -> (w131:T6)
            n45 = Bundle By Name(cluster=w143, "state"=w133, "res_row_cnt"=w140, "res_col"=w139, "res_range_type"=res_range_type_cntrl."100", "chnl_col"=w139, "range_setting"=w141, "first_time_set"=w141, "100_list_ch"=w139, "100_list_row_cnt"=w140, "1K_list_ch"=w139, "1K_list_row_cnt"=w140, "10K_list_ch"=w139, "10K_list_row_cnt"=w140, "100K_list_ch"=w139, "100K_list_row_cnt"=w140, "1M_list_ch"=w139, "1M_list_row_cnt"=w140, "10M_list_ch"=w139, "10M_list_row_cnt"=w140, "100M_list_ch"=w139, "100M_list_row_cnt"=w140, "list_flag"=w141, "ch_list_set_cnt"=w140, "res_tot_cnt"=w140, "slot_col"=w139, "scan_data"=string[] ["", "", "", "", "", "", "", "", "", "", "", "", "", "", "", "", "", "", "", "", "", "", "", "", "", "", "", "", "", "", "", "", "", "", "", "", "", "", "", " "], "res_table_text"=string[][] [["", "", "", "", "", ""], ["", "", "", "", "", ""], ["", "", "", "", "", ""], ["", "", "", "", "", ""], ["", "", "", "", "", ""], ["", "", "", "", "", ""], ["", "", "", "", "", ""], ["", "", "", "", "", ""], ["", "", "", "", "", ""], ["", "", "", "", "", ""], ["", "", "", "", "", ""], ["", "", "", "", "", ""], ["", "", "", "", "", ""], ["", "", "", "", "", ""], ["", "", "", "", "", ""], ["", "", "", "", "", ""], ["", "", "", "", "", ""], ["", "", "", "", "", ""], ["", "", "", "", "", ""], ["", "", "", "", "", ""], ["", "", "", "", "", ""], ["", "", "", "", "", ""], ["", "", "", "", "", ""], ["", "", "", "", "", ""], ["", "", "", "", "", ""], ["", "", "", "", "", ""], ["", "", "", "", "", ""], ["", "", "", "", "", ""], ["", "", "", "", "", ""], ["", "", "", "", "", ""], ["", "", "", "", "", ""], ["", "", "", "", "", ""], ["", "", "", "", "", ""], ["", "", "", "", "", ""], ["", "", "", "", "", ""], ["", "", "", "", "", ""], ["", "", "", "", "", ""], ["", "", "", "", "", ""], ["", "", "", "", "", ""], ["", "", "", "", "", ""], ["", "", "", "", "", ""], ["", "", "", "", "", ""], ["", "", "", "", "", ""], ["", "", "", "", "", ""], ["", "", "", "", "", ""], ["", "", "", "", "", ""], ["", "", "", "", "", ""], ["", "", "", "", "", ""], ["", "", "", "", "", ""], ["", "", "", "", "", ""], ["", "", "", "", "", ""], ["", "", "", "", "", ""], ["", "", "", "", "", ""], ["", "", "", "", "", ""], ["", "", "", "", "", ""], ["", "", "", "", "", ""], ["", "", "", "", "", ""], ["", "", "", "", "", ""], ["", "", "", "", "", ""], ["", "", "", "", "", ""], ["", "", "", "", "", ""], ["", "", "", "", "", ""], ["", "", "", "", "", ""], ["", "", "", "", "", ""], ["", "", "", "", "", ""], ["", "", "", "", "", ""], ["", "", "", "", "", ""], ["", "", "", "", "", ""], ["", "", "", "", "", " "]]) -> (w138:T7)
            n46 = Enqueue Element(queue=w134, element=w131) -> ()  [unwired: 2 in, 3 out]
            n47 = Bundle By Name(cluster=w138, "ch_list_indx_100"=w135, "ch_list_indx_1K"=w135, "ch_list_indx_10K"=w135, "ch_list_indx_100K"=w135, "ch_list_indx_1M"=w135, "ch_list_indx_10M"=w135, "ch_list_indx_100M"=w135, "res_table"=dbl[][] [[0.0, 0.0, 0.0, 0.0], [0.0, 0.0, 0.0, 0.0], [0.0, 0.0, 0.0, 0.0], [0.0, 0.0, 0.0, 0.0], [0.0, 0.0, 0.0, 0.0], [0.0, 0.0, 0.0, 0.0], [0.0, 0.0, 0.0, 0.0], [0.0, 0.0, 0.0, 0.0], [0.0, 0.0, 0.0, 0.0], [0.0, 0.0, 0.0, 0.0], [0.0, 0.0, 0.0, 0.0], [0.0, 0.0, 0.0, 0.0], [0.0, 0.0, 0.0, 0.0], [0.0, 0.0, 0.0, 0.0], [0.0, 0.0, 0.0, 0.0], [0.0, 0.0, 0.0, 0.0], [0.0, 0.0, 0.0, 0.0], [0.0, 0.0, 0.0, 0.0], [0.0, 0.0, 0.0, 0.0], [0.0, 0.0, 0.0, 0.0], [0.0, 0.0, 0.0, 0.0], [0.0, 0.0, 0.0, 0.0], [0.0, 0.0, 0.0, 0.0], [0.0, 0.0, 0.0, 0.0], [0.0, 0.0, 0.0, 0.0], [0.0, 0.0, 0.0, 0.0], [0.0, 0.0, 0.0, 0.0], [0.0, 0.0, 0.0, 0.0], [0.0, 0.0, 0.0, 0.0], [0.0, 0.0, 0.0, 0.0], [0.0, 0.0, 0.0, 0.0], [0.0, 0.0, 0.0, 0.0], [0.0, 0.0, 0.0, 0.0], [0.0, 0.0, 0.0, 0.0], [0.0, 0.0, 0.0, 0.0], [0.0, 0.0, 0.0, 0.0], [0.0, 0.0, 0.0, 0.0], [0.0, 0.0, 0.0, 0.0], [0.0, 0.0, 0.0, 0.0], [0.0, 0.0, 0.0, 0.0], [0.0, 0.0, 0.0, 0.0], [0.0, 0.0, 0.0, 0.0], [0.0, 0.0, 0.0, 0.0], [0.0, 0.0, 0.0, 0.0], [0.0, 0.0, 0.0, 0.0], [0.0, 0.0, 0.0, 0.0], [0.0, 0.0, 0.0, 0.0], [0.0, 0.0, 0.0, 0.0], [0.0, 0.0, 0.0, 0.0], [0.0, 0.0, 0.0, 0.0], [0.0, 0.0, 0.0, 0.0], [0.0, 0.0, 0.0, 0.0], [0.0, 0.0, 0.0, 0.0], [0.0, 0.0, 0.0, 0.0], [0.0, 0.0, 0.0, 0.0], [0.0, 0.0, 0.0, 0.0], [0.0, 0.0, 0.0, 0.0], [0.0, 0.0, 0.0, 0.0], [0.0, 0.0, 0.0, 0.0], [0.0, 0.0, 0.0, 0.0], [0.0, 0.0, 0.0, 0.0], [0.0, 0.0, 0.0, 0.0], [0.0, 0.0, 0.0, 0.0], [0.0, 0.0, 0.0, 0.0], [0.0, 0.0, 0.0, 0.0], [0.0, 0.0, 0.0, 0.0], [0.0, 0.0, 0.0, 0.0], [0.0, 0.0, 0.0, 0.0], [0.0, 0.0, 0.0, 0.0]]) -> (w137:T7)
            n48 = local write "start"(FALSE ("start")) -> ()
          }
          frame "read_res_col" {
            # "4"
            # "3"
            # "Read all data from file."
            # "2"
            # "1"
            # "1.  resistor values are at column 2\n2.  set to 0 when we first open a file\n3.  channels column\n4.  slot number column"
            n49 = Unbundle By Name(w147) -> ("res_table_text"=w146:string[][])
            n50 = Read from Text File(file (use dialog)="res_path") -> (text=w164:string)  [unwired: 3 in, 3 out]
            "text_file" <- w164
            n51 = Spreadsheet String To Array(delimiter (Tab)=",", format string="%10.2f", spreadsheet string=w164, array type (2D Dbl)=dbl[][] []) -> (array=w145:dbl[][])
            "array" <- w145
            n52 = for {
              shift-right: [w170] -> w144
              shift-left: w146 -> [w171]
              tunnel: w145 -> [w168] mode=indexing
              i -> [w169]
              n53 = Number To Fractional String(number=w168, precision (6)=i16 2) -> (F-format string=w167:string[])  [unwired: 2 in]
              n54 = Replace Array Subset(array=w171, new element=w167, index (row)=w169) -> (w170:string[][])  [unwired: 1 in]
            }
            "res_table" <- w144
            n55 = Bundle By Name(cluster=w160, "state"=state_cntrl."res_val_qry") -> (w159:T6)
            n56 = Index Array(array=w145, index (col) #1=0 ("disabled index (col)"), index (col) #2=1 ("disabled index (col)"), index (col) #3=2 ("disabled index (col)")) -> (element #1=w149:dbl[], element #2=w153:dbl[], element #3=w152:dbl[])  [unwired: 3 in]
            n57 = Enqueue Element(queue=w161, element=w159) -> ()  [unwired: 2 in, 3 out]
            n58 = Array Size(array=w152) -> (size(s)=w151:i32)
            n59 = Bundle By Name(cluster=w147, "res_table"=w145, "slot_col"=w149, "res_tot_cnt"=w151, "chnl_col"=w153, "res_col"=w152, "res_row_cnt"=0 ("res_col_cnt"), "res_table_text"=w144) -> (w155:T7)
          }
          frame "res_val_qry" {
            w176 = 10000000.0 ("y")
            w181 = 1000000.0 ("y")
            w185 = 100000.0 ("y")
            w189 = 10000.0 ("y")
            w193 = 1000.0 ("y")
            w197 = 100.0 ("y")
            # "asks if we're\nin between"
            # "go to that range\nstate"
            # "decides if we're in\na certain range"
            # "Read resistor from each row."
            n60 = Unbundle By Name(w172) -> ("range_setting"=w200:bool[], "res_col"=w217:dbl[], "res_row_cnt"=w216:i32)
            n61 = Index Array(array=w217, index=w216) -> (element=w177:dbl)
            n62 = Less?(x=w177, y=w197) -> (x < y?=w199:bool)
            n63 = Greater Or Equal?(x=w177, y=w197) -> (x >= y?=w196:bool)
            n64 = Less?(x=w177, y=w193) -> (x < y?=w195:bool)
            n65 = Greater Or Equal?(x=w177, y=w193) -> (x >= y?=w192:bool)
            n66 = Less?(x=w177, y=w189) -> (x < y?=w191:bool)
            n67 = Greater Or Equal?(x=w177, y=w189) -> (x >= y?=w188:bool)
            n68 = Less?(x=w177, y=w185) -> (x < y?=w187:bool)
            n69 = Greater Or Equal?(x=w177, y=w185) -> (x >= y?=w184:bool)
            n70 = Less?(x=w177, y=w181) -> (x < y?=w183:bool)
            n71 = Greater Or Equal?(x=w177, y=w181) -> (x >= y?=w180:bool)
            n72 = Less?(x=w177, y=w176) -> (x < y?=w179:bool)
            n73 = Greater Or Equal?(x=w177, y=w176) -> (x >= y?=w175:bool)
            n74 = Less?(x=w177, y=100000000.0) -> (x < y?=w174:bool)
            n75 = And(x=w196, y=w195) -> (x .and. y?=w194:bool)
            n76 = And(x=w192, y=w191) -> (x .and. y?=w190:bool)
            n77 = And(x=w188, y=w187) -> (x .and. y?=w186:bool)
            n78 = And(x=w184, y=w183) -> (x .and. y?=w182:bool)
            n79 = And(x=w180, y=w179) -> (x .and. y?=w178:bool)
            n80 = And(x=w175, y=w174) -> (x .and. y?=w173:bool)
            n81 = Replace Array Subset(array=w200, new element #1=w199, new element #2=w194, new element #3=w190, new element #4=w186, new element #5=w182, new element #6=w178, new element #7=w173) -> (w202:bool[])  [unwired: 7 in]
            n82 = Select(t=state_cntrl."plc_ch_in_10M_list" ("state"), s=w178, f=state_cntrl."plc_ch_in_100M_list" ("state")) -> (s? t:f=w211:T1)
            n83 = Select(t=state_cntrl."plc_ch_in_1M_list" ("state"), s=w182, f=w211) -> (s? t:f=w212:T1)
            n84 = Select(t=state_cntrl."plc_ch_in_100K_list" ("state"), s=w186, f=w212) -> (s? t:f=w213:T1)
            n85 = Select(t=state_cntrl."plc_ch_in_10K_list" ("state"), s=w190, f=w213) -> (s? t:f=w214:T1)
            n86 = Select(t=state_cntrl."plc_ch_in_1K_list" ("state"), s=w194, f=w214) -> (s? t:f=w215:T1)
            n87 = Select(t=state_cntrl."plc_ch_in_100_list" ("state"), s=w199, f=w215) -> (s? t:f=w209:T1)
            n88 = Bundle By Name(cluster=w172, "range_setting"=w202) -> (w201:T7)
            n89 = Bundle By Name(cluster=w218, "state"=w209) -> (w219:T6)
            n90 = Enqueue Element(queue=w220, element=w219) -> ()  [unwired: 2 in, 3 out]
          }
          frame "plc_ch_in_100_list" {
            # "move to the next row"
            # "Store the index of the resistors array\nwhere the 100 ohm range exists."
            # "Increase count so we can\nmove to the next element\nof the resistors array."
            # "if first time, set to true.\nif not, leave it where it is"
            # "first time,\nif previously F and\nnow T, it is the first\ntime"
            # "Read resistor from each row\nand place it in the 100 ohm list."
            n91 = Unbundle By Name(w246) -> ("first_time_set"=w234:bool[], "range_setting"=w240:bool[], "100_list_row_cnt"=w225:i32, "chnl_col"=w245:dbl[], "res_row_cnt"=w223:i32, "ch_list_indx_100"=w222:i32[])
            n92 = Index Array(array=w234) -> (element=w232:bool)  [unwired: 1 in]
            n93 = Index Array(array=w240) -> (element=w239:bool)  [unwired: 1 in]
            n94 = Equal?(x=FALSE, y=w232) -> (x = y?=w236:bool)
            n95 = Equal?(x=TRUE, y=w239) -> (x = y?=w235:bool)
            n96 = Increment(x=w225) -> (x+1=w242:i32)
            n97 = Increment(x=w223) -> (x+1=w224:i32)
            n98 = And(x=w236, y=w235) -> (x .and. y?=w230:bool)
            n99 = Index Array(array=w245, index=w223) -> (element=w244:dbl)
            n100 = Select(t=TRUE ("x"), s=w230, f=w232) -> (s? t:f=w231:bool)
            n101 = Replace Array Subset(array=w234, new element=w231) -> (w226:bool[])  [unwired: 1 in]
            n102 = Replace Array Subset(array=w245, new element=w244, index=w225) -> (w243:dbl[])
            n103 = Replace Array Subset(array=w222, new element=w223, index=w225) -> ()  [unwired: 1 out]
            n104 = Build Array (concatenate)(w222, w223) -> (w221:i32[])
            n105 = Select(t=state_cntrl."set_100_list_flg" ("state"), s=w230, f=state_cntrl."fin_arry_qry") -> (s? t:f=w228:T1)
            n106 = Bundle By Name(cluster=w247, "state"=w228) -> (w248:T6)
            n107 = Bundle By Name(cluster=w246, "first_time_set"=w226, "100_list_ch"=w243, "100_list_row_cnt"=w242, "ch_list_indx_100"=w221, "res_row_cnt"=w224) -> (w241:T7)
            n108 = Enqueue Element(queue=w249, element=w248) -> ()  [unwired: 2 in, 3 out]
          }
          frame "set_100_list_flg" {
            # "Increase the channel list count if we\nhave another set of range to measure."
            # "Set the array element for the\n100 ohm set."
            # "Set the 100 ohm list flag to\nindicate that we have something\nto measure in this range."
            n109 = Unbundle By Name(w257) -> ("list_flag"=w253:bool[], "ch_list_set_cnt"=w256:i32)
            n110 = Increment(x=w256) -> (x+1=w255:i32)
            n111 = Replace Array Subset(array=w253, new element=TRUE ("new element/subarray")) -> (w252:bool[])  [unwired: 1 in]
            n112 = Bundle By Name(cluster=w258, "state"=state_cntrl."fin_arry_qry" ("f")) -> (w259:T6)
            n113 = Bundle By Name(cluster=w257, "list_flag"=w252, "ch_list_set_cnt"=w255) -> (w254:T7)
            n114 = Enqueue Element(queue=w260, element=w259) -> ()  [unwired: 2 in, 3 out]
          }
          frame "plc_ch_in_1K_list" {
            w266 = 1 ("index")
            # "move to the next row"
            # "Store the index of the resistors array\nwhere the 1K ohm range exists."
            # "Read resistor from each row\nand place it in the 1K ohm list."
            # "if first time, set to true.\nif not, leave it where it is"
            # "first time,\nif previously F and\nnow T, it is the first\ntime"
            n115 = Unbundle By Name(w287) -> ("first_time_set"=w275:bool[], "range_setting"=w281:bool[], "1K_list_row_cnt"=w265:i32, "chnl_col"=w286:dbl[], "res_row_cnt"=w262:i32, "ch_list_indx_1K"=w263:i32[])
            n116 = Index Array(array=w275, index=w266) -> (element=w273:bool)
            n117 = Index Array(array=w281, index=w266) -> (element=w280:bool)
            n118 = Equal?(x=FALSE, y=w273) -> (x = y?=w277:bool)
            n119 = Equal?(x=TRUE, y=w280) -> (x = y?=w276:bool)
            n120 = Increment(x=w265) -> (x+1=w283:i32)
            n121 = Increment(x=w262) -> (x+1=w264:i32)
            n122 = And(x=w277, y=w276) -> (x .and. y?=w271:bool)
            n123 = Index Array(array=w286, index=w262) -> (element=w285:dbl)
            n124 = Select(t=TRUE ("x"), s=w271, f=w273) -> (s? t:f=w272:bool)
            n125 = Replace Array Subset(array=w275, new element=w272, index=w266) -> (w267:bool[])
            n126 = Replace Array Subset(array=w286, new element=w285, index=w265) -> (w284:dbl[])
            n127 = Replace Array Subset(array=w263, new element=w262, index=w265) -> ()  [unwired: 1 out]
            n128 = Build Array (concatenate)(w263, w262) -> (w261:i32[])
            n129 = Select(t=state_cntrl."set_1K_list_flg" ("state"), s=w271, f=state_cntrl."fin_arry_qry") -> (s? t:f=w269:T1)
            n130 = Bundle By Name(cluster=w288, "state"=w269) -> (w289:T6)
            n131 = Bundle By Name(cluster=w287, "first_time_set"=w267, "1K_list_ch"=w284, "1K_list_row_cnt"=w283, "ch_list_indx_1K"=w261, "res_row_cnt"=w264) -> (w282:T7)
            n132 = Enqueue Element(queue=w290, element=w289) -> ()  [unwired: 2 in, 3 out]
          }
          frame "set_1K_list_flg" {
            # "Set the array element for the\n1K ohm set."
            # "Set the 1K ohm list flag to\nindicate that we have something\nto measure in this range."
            n133 = Unbundle By Name(w299) -> ("list_flag"=w295:bool[], "ch_list_set_cnt"=w298:i32)
            n134 = Increment(x=w298) -> (x+1=w297:i32)
            n135 = Replace Array Subset(array=w295, new element=TRUE ("new element/subarray"), index=1) -> (w294:bool[])
            n136 = Bundle By Name(cluster=w300, "state"=state_cntrl."fin_arry_qry" ("f")) -> (w301:T6)
            n137 = Bundle By Name(cluster=w299, "list_flag"=w294, "ch_list_set_cnt"=w297) -> (w296:T7)
            n138 = Enqueue Element(queue=w302, element=w301) -> ()  [unwired: 2 in, 3 out]
          }
          frame "plc_ch_in_10K_list" {
            w308 = 2 ("index")
            # "move to the next row"
            # "Store the index of the resistors array\nwhere the 10K ohm range exists."
            # "Read resistor from each row\nand place it in the 10K ohm list."
            # "if first time, set to true.\nif not, leave it where it is"
            # "first time,\nif previously F and\nnow T, it is the first\ntime"
            n139 = Unbundle By Name(w329) -> ("first_time_set"=w317:bool[], "range_setting"=w323:bool[], "10K_list_row_cnt"=w307:i32, "chnl_col"=w328:dbl[], "res_row_cnt"=w304:i32, "ch_list_indx_10K"=w305:i32[])
            n140 = Index Array(array=w317, index=w308) -> (element=w315:bool)
            n141 = Index Array(array=w323, index=w308) -> (element=w322:bool)
            n142 = Equal?(x=FALSE, y=w315) -> (x = y?=w319:bool)
            n143 = Equal?(x=TRUE, y=w322) -> (x = y?=w318:bool)
            n144 = Increment(x=w307) -> (x+1=w325:i32)
            n145 = Increment(x=w304) -> (x+1=w306:i32)
            n146 = And(x=w319, y=w318) -> (x .and. y?=w313:bool)
            n147 = Index Array(array=w328, index=w304) -> (element=w327:dbl)
            n148 = Select(t=TRUE ("x"), s=w313, f=w315) -> (s? t:f=w314:bool)
            n149 = Replace Array Subset(array=w317, new element=w314, index=w308) -> (w309:bool[])
            n150 = Replace Array Subset(array=w328, new element=w327, index=w307) -> (w326:dbl[])
            n151 = Replace Array Subset(array=w305, new element=w304, index=w307) -> ()  [unwired: 1 out]
            n152 = Build Array (concatenate)(w305, w304) -> (w303:i32[])
            n153 = Select(t=state_cntrl."set_10K_list_flg" ("state"), s=w313, f=state_cntrl."fin_arry_qry") -> (s? t:f=w311:T1)
            n154 = Bundle By Name(cluster=w330, "state"=w311) -> (w331:T6)
            n155 = Bundle By Name(cluster=w329, "first_time_set"=w309, "10K_list_ch"=w326, "10K_list_row_cnt"=w325, "ch_list_indx_10K"=w303, "res_row_cnt"=w306) -> (w324:T7)
            n156 = Enqueue Element(queue=w332, element=w331) -> ()  [unwired: 2 in, 3 out]
          }
          frame "set_10K_list_flg" {
            # "Set the array element for the\n10K ohm set."
            # "Set the 10K ohm list flag to\nindicate that we have something\nto measure in this range."
            n157 = Unbundle By Name(w341) -> ("list_flag"=w337:bool[], "ch_list_set_cnt"=w340:i32)
            n158 = Increment(x=w340) -> (x+1=w339:i32)
            n159 = Replace Array Subset(array=w337, new element=TRUE ("new element/subarray"), index=2) -> (w336:bool[])
            n160 = Bundle By Name(cluster=w342, "state"=state_cntrl."fin_arry_qry" ("f")) -> (w343:T6)
            n161 = Bundle By Name(cluster=w341, "list_flag"=w336, "ch_list_set_cnt"=w339) -> (w338:T7)
            n162 = Enqueue Element(queue=w344, element=w343) -> ()  [unwired: 2 in, 3 out]
          }
          frame "plc_ch_in_100K_list" {
            w350 = 3 ("index")
            # "move to the next row"
            # "Store the index of the resistors array\nwhere the 100K ohm range exists."
            # "Read resistor from each row\nand place it in the 100K ohm list."
            # "if first time, set to true.\nif not, leave it where it is"
            # "first time,\nif previously F and\nnow T, it is the first\ntime"
            n163 = Unbundle By Name(w371) -> ("first_time_set"=w359:bool[], "range_setting"=w365:bool[], "100K_list_row_cnt"=w349:i32, "chnl_col"=w370:dbl[], "res_row_cnt"=w346:i32, "ch_list_indx_100K"=w347:i32[])
            n164 = Index Array(array=w359, index=w350) -> (element=w357:bool)
            n165 = Index Array(array=w365, index=w350) -> (element=w364:bool)
            n166 = Equal?(x=FALSE, y=w357) -> (x = y?=w361:bool)
            n167 = Equal?(x=TRUE, y=w364) -> (x = y?=w360:bool)
            n168 = Increment(x=w349) -> (x+1=w367:i32)
            n169 = Increment(x=w346) -> (x+1=w348:i32)
            n170 = And(x=w361, y=w360) -> (x .and. y?=w355:bool)
            n171 = Index Array(array=w370, index=w346) -> (element=w369:dbl)
            n172 = Select(t=TRUE ("x"), s=w355, f=w357) -> (s? t:f=w356:bool)
            n173 = Replace Array Subset(array=w359, new element=w356, index=w350) -> (w351:bool[])
            n174 = Replace Array Subset(array=w370, new element=w369, index=w349) -> (w368:dbl[])
            n175 = Replace Array Subset(array=w347, new element=w346, index=w349) -> ()  [unwired: 1 out]
            n176 = Build Array (concatenate)(w347, w346) -> (w345:i32[])
            n177 = Select(t=state_cntrl."set_100K_list_flg" ("state"), s=w355, f=state_cntrl."fin_arry_qry") -> (s? t:f=w353:T1)
            n178 = Bundle By Name(cluster=w372, "state"=w353) -> (w373:T6)
            n179 = Bundle By Name(cluster=w371, "first_time_set"=w351, "100K_list_ch"=w368, "100K_list_row_cnt"=w367, "ch_list_indx_100K"=w345, "res_row_cnt"=w348) -> (w366:T7)
            n180 = Enqueue Element(queue=w374, element=w373) -> ()  [unwired: 2 in, 3 out]
          }
          frame "set_100K_list_flg" {
            # "Set the array element for the\n100K ohm set."
            # "Set the 100K ohm list flag to\nindicate that we have something\nto measure in this range."
            n181 = Unbundle By Name(w383) -> ("list_flag"=w379:bool[], "ch_list_set_cnt"=w382:i32)
            n182 = Increment(x=w382) -> (x+1=w381:i32)
            n183 = Replace Array Subset(array=w379, new element=TRUE ("new element/subarray"), index=3) -> (w378:bool[])
            n184 = Bundle By Name(cluster=w384, "state"=state_cntrl."fin_arry_qry" ("f")) -> (w385:T6)
            n185 = Bundle By Name(cluster=w383, "list_flag"=w378, "ch_list_set_cnt"=w381) -> (w380:T7)
            n186 = Enqueue Element(queue=w386, element=w385) -> ()  [unwired: 2 in, 3 out]
          }
          frame "plc_ch_in_1M_list" {
            w392 = 4 ("index")
            # "move to the next row"
            # "Store the index of the resistors array\nwhere the 1M ohm range exists."
            # "Read resistor from each row\nand place it in the 1M ohm list."
            # "if first time, set to true.\nif not, leave it where it is"
            # "first time,\nif previously F and\nnow T, it is the first\ntime"
            n187 = Unbundle By Name(w413) -> ("first_time_set"=w401:bool[], "range_setting"=w407:bool[], "1M_list_row_cnt"=w391:i32, "chnl_col"=w412:dbl[], "res_row_cnt"=w388:i32, "ch_list_indx_1M"=w389:i32[])
            n188 = Index Array(array=w401, index=w392) -> (element=w399:bool)
            n189 = Index Array(array=w407, index=w392) -> (element=w406:bool)
            n190 = Equal?(x=FALSE, y=w399) -> (x = y?=w403:bool)
            n191 = Equal?(x=TRUE, y=w406) -> (x = y?=w402:bool)
            n192 = Increment(x=w391) -> (x+1=w409:i32)
            n193 = Increment(x=w388) -> (x+1=w390:i32)
            n194 = And(x=w403, y=w402) -> (x .and. y?=w397:bool)
            n195 = Index Array(array=w412, index=w388) -> (element=w411:dbl)
            n196 = Select(t=TRUE ("x"), s=w397, f=w399) -> (s? t:f=w398:bool)
            n197 = Replace Array Subset(array=w401, new element=w398, index=w392) -> (w393:bool[])
            n198 = Replace Array Subset(array=w412, new element=w411, index=w391) -> (w410:dbl[])
            n199 = Replace Array Subset(array=w389, new element=w388, index=w391) -> ()  [unwired: 1 out]
            n200 = Build Array (concatenate)(w389, w388) -> (w387:i32[])
            n201 = Select(t=state_cntrl."set_1M_list_flg" ("state"), s=w397, f=state_cntrl."fin_arry_qry") -> (s? t:f=w395:T1)
            n202 = Bundle By Name(cluster=w414, "state"=w395) -> (w415:T6)
            n203 = Bundle By Name(cluster=w413, "first_time_set"=w393, "1M_list_ch"=w410, "1M_list_row_cnt"=w409, "ch_list_indx_1M"=w387, "res_row_cnt"=w390) -> (w408:T7)
            n204 = Enqueue Element(queue=w416, element=w415) -> ()  [unwired: 2 in, 3 out]
          }
          frame "set_1M_list_flg" {
            # "Set the array element for the\n1M ohm set."
            # "Set the 1M ohm list flag to\nindicate that we have something\nto measure in this range."
            n205 = Unbundle By Name(w425) -> ("list_flag"=w421:bool[], "ch_list_set_cnt"=w424:i32)
            n206 = Increment(x=w424) -> (x+1=w423:i32)
            n207 = Replace Array Subset(array=w421, new element=TRUE ("new element/subarray"), index=4) -> (w420:bool[])
            n208 = Bundle By Name(cluster=w426, "state"=state_cntrl."fin_arry_qry" ("f")) -> (w427:T6)
            n209 = Bundle By Name(cluster=w425, "list_flag"=w420, "ch_list_set_cnt"=w423) -> (w422:T7)
            n210 = Enqueue Element(queue=w428, element=w427) -> ()  [unwired: 2 in, 3 out]
          }
          frame "plc_ch_in_10M_list" {
            w434 = 5 ("index")
            # "Store the index of the resistors array\nwhere the 10M ohm range exists."
            # "Read resistor from each row\nand place it in the 10M ohm list."
            # "if first time, set to true.\nif not, leave it where it is"
            # "first time,\nif previously F and\nnow T, it is the first\ntime"
            n211 = Unbundle By Name(w455) -> ("first_time_set"=w443:bool[], "range_setting"=w449:bool[], "10M_list_row_cnt"=w433:i32, "chnl_col"=w454:dbl[], "res_row_cnt"=w430:i32, "ch_list_indx_10M"=w431:i32[])
            n212 = Index Array(array=w443, index=w434) -> (element=w441:bool)
            n213 = Index Array(array=w449, index=w434) -> (element=w448:bool)
            n214 = Equal?(x=FALSE, y=w441) -> (x = y?=w445:bool)
            n215 = Equal?(x=TRUE, y=w448) -> (x = y?=w444:bool)
            n216 = Increment(x=w433) -> (x+1=w451:i32)
            n217 = Increment(x=w430) -> (x+1=w432:i32)
            n218 = And(x=w445, y=w444) -> (x .and. y?=w439:bool)
            n219 = Index Array(array=w454, index=w430) -> (element=w453:dbl)
            n220 = Select(t=TRUE ("x"), s=w439, f=w441) -> (s? t:f=w440:bool)
            n221 = Replace Array Subset(array=w443, new element=w440, index=w434) -> (w435:bool[])
            n222 = Replace Array Subset(array=w454, new element=w453, index=w433) -> (w452:dbl[])
            n223 = Replace Array Subset(array=w431, new element=w430, index=w433) -> ()  [unwired: 1 out]
            n224 = Build Array (concatenate)(w431, w430) -> (w429:i32[])
            n225 = Select(t=state_cntrl."set_10M_list_flg" ("state"), s=w439, f=state_cntrl."fin_arry_qry") -> (s? t:f=w437:T1)
            n226 = Bundle By Name(cluster=w456, "state"=w437) -> (w457:T6)
            n227 = Bundle By Name(cluster=w455, "first_time_set"=w435, "10M_list_ch"=w452, "10M_list_row_cnt"=w451, "ch_list_indx_10M"=w429, "res_row_cnt"=w432) -> (w450:T7)
            n228 = Enqueue Element(queue=w458, element=w457) -> ()  [unwired: 2 in, 3 out]
          }
          frame "set_10M_list_flg" {
            # "Set the array element for the\n10M ohm set."
            # "Set the 10M ohm list flag to\nindicate that we have something\nto measure in this range."
            n229 = Unbundle By Name(w467) -> ("list_flag"=w463:bool[], "ch_list_set_cnt"=w466:i32)
            n230 = Increment(x=w466) -> (x+1=w465:i32)
            n231 = Replace Array Subset(array=w463, new element=TRUE ("new element/subarray"), index=5) -> (w462:bool[])
            n232 = Bundle By Name(cluster=w468, "state"=state_cntrl."fin_arry_qry" ("f")) -> (w469:T6)
            n233 = Bundle By Name(cluster=w467, "list_flag"=w462, "ch_list_set_cnt"=w465) -> (w464:T7)
            n234 = Enqueue Element(queue=w470, element=w469) -> ()  [unwired: 2 in, 3 out]
          }
          frame "plc_ch_in_100M_list" {
            w476 = 6 ("index")
            # "move to the next row"
            # "Store the index of the resistors array\nwhere the 1K ohm range exists."
            # "Read resistor from each row\nand place it in the 100M ohm list."
            # "if first time, set to true.\nif not, leave it where it is"
            # "first time,\nif previously F and\nnow T, it is the first\ntime"
            n235 = Unbundle By Name(w497) -> ("first_time_set"=w485:bool[], "range_setting"=w491:bool[], "100M_list_row_cnt"=w475:i32, "chnl_col"=w496:dbl[], "res_row_cnt"=w472:i32, "ch_list_indx_100M"=w473:i32[])
            n236 = Index Array(array=w485, index=w476) -> (element=w483:bool)
            n237 = Index Array(array=w491, index=w476) -> (element=w490:bool)
            n238 = Equal?(x=FALSE, y=w483) -> (x = y?=w487:bool)
            n239 = Equal?(x=TRUE, y=w490) -> (x = y?=w486:bool)
            n240 = Increment(x=w475) -> (x+1=w493:i32)
            n241 = Increment(x=w472) -> (x+1=w474:i32)
            n242 = And(x=w487, y=w486) -> (x .and. y?=w481:bool)
            n243 = Index Array(array=w496, index=w472) -> (element=w495:dbl)
            n244 = Select(t=TRUE ("x"), s=w481, f=w483) -> (s? t:f=w482:bool)
            n245 = Replace Array Subset(array=w485, new element=w482, index=w476) -> (w477:bool[])
            n246 = Replace Array Subset(array=w496, new element=w495, index=w475) -> (w494:dbl[])
            n247 = Replace Array Subset(array=w473, new element=w472, index=w475) -> ()  [unwired: 1 out]
            n248 = Build Array (concatenate)(w473, w472) -> (w471:i32[])
            n249 = Select(t=state_cntrl."set_100M_list_flg" ("state"), s=w481, f=state_cntrl."fin_arry_qry") -> (s? t:f=w479:T1)
            n250 = Bundle By Name(cluster=w498, "state"=w479) -> (w499:T6)
            n251 = Bundle By Name(cluster=w497, "first_time_set"=w477, "100M_list_ch"=w494, "100M_list_row_cnt"=w493, "ch_list_indx_100M"=w471, "res_row_cnt"=w474) -> (w492:T7)
            n252 = Enqueue Element(queue=w500, element=w499) -> ()  [unwired: 2 in, 3 out]
          }
          frame "set_100M_list_flg" {
            # "Set the array element for the\n100M ohm set."
            # "Set the 100M ohm list flag to\nindicate that we have something\nto measure in this range."
            n253 = Unbundle By Name(w509) -> ("list_flag"=w505:bool[], "ch_list_set_cnt"=w508:i32)
            n254 = Increment(x=w508) -> (x+1=w507:i32)
            n255 = Replace Array Subset(array=w505, new element=TRUE ("new element/subarray"), index=6) -> (w504:bool[])
            n256 = Bundle By Name(cluster=w510, "state"=state_cntrl."fin_arry_qry" ("f")) -> (w511:T6)
            n257 = Bundle By Name(cluster=w509, "list_flag"=w504, "ch_list_set_cnt"=w507) -> (w506:T7)
            n258 = Enqueue Element(queue=w512, element=w511) -> ()  [unwired: 2 in, 3 out]
          }
          frame "fin_arry_qry" {
            # "If we have finished with checking all of the\nresistors in the array, go check the 100 ohm\nchannel list."
            n259 = Unbundle By Name(w513) -> ("res_tot_cnt"=w519:i32, "res_row_cnt"=w518:i32)
            n260 = Equal?(x=w519, y=w518) -> (x = y?=w517:bool)
            n261 = Select(t=state_cntrl."chk_100_list_flg", s=w517, f=state_cntrl."res_val_qry") -> (s? t:f=w515:T1)
            n262 = Bundle By Name(cluster=w520, "state"=w515) -> (w521:T6)
            n263 = Enqueue Element(queue=w522, element=w521) -> ()  [unwired: 2 in, 3 out]
          }
          frame "chk_100_list_flg" {
            # "Check to see if there is any resistor to measure\nin the 100 ohm range list.  If not, check the\n1K ohm list."
            n264 = Unbundle By Name(w525) -> ("list_flag"=w524:bool[])
            n265 = Index Array(array=w524) -> (element=w523:bool)  [unwired: 1 in]
            n266 = Select(t=state_cntrl."set_100_ohm_chnl_list", s=w523, f=state_cntrl."chk_1K_list_flg") -> (s? t:f=w527:T1)
            n267 = Bundle By Name(cluster=w529, "state"=w527) -> (w530:T6)
            n268 = Enqueue Element(queue=w531, element=w530) -> ()  [unwired: 2 in, 3 out]
          }
          frame "chk_1K_list_flg" {
            # "Check to see if there is any resistor to measure\nin the 1K ohm range list.  If not, check the\n10K ohm list."
            n269 = Unbundle By Name(w535) -> ("list_flag"=w534:bool[])
            n270 = Index Array(array=w534, index=1) -> (element=w533:bool)
            n271 = Select(t=state_cntrl."set_1K_ohm_chnl_list", s=w533, f=state_cntrl."chk_10K_list_flg") -> (s? t:f=w537:T1)
            n272 = Bundle By Name(cluster=w539, "state"=w537) -> (w540:T6)
            n273 = Enqueue Element(queue=w541, element=w540) -> ()  [unwired: 2 in, 3 out]
          }
          frame "chk_10K_list_flg" {
            # "Check to see if there is any resistor to measure\nin the 10K ohm range list.  If not, check the\n100K ohm list."
            n274 = Unbundle By Name(w545) -> ("list_flag"=w544:bool[])
            n275 = Index Array(array=w544, index=2) -> (element=w543:bool)
            n276 = Select(t=state_cntrl."set_10K_ohm_chnl_list", s=w543, f=state_cntrl."chk_100K_list_flg") -> (s? t:f=w547:T1)
            n277 = Bundle By Name(cluster=w549, "state"=w547) -> (w550:T6)
            n278 = Enqueue Element(queue=w551, element=w550) -> ()  [unwired: 2 in, 3 out]
          }
          frame "chk_100K_list_flg" {
            # "Check to see if there is any resistor to measure\nin the 100K ohm range list.  If not, check the\n1M ohm list."
            n279 = Unbundle By Name(w555) -> ("list_flag"=w554:bool[])
            n280 = Index Array(array=w554, index=3) -> (element=w553:bool)
            n281 = Select(t=state_cntrl."set_100K_ohm_chnl_list", s=w553, f=state_cntrl."chk_1M_list_flg") -> (s? t:f=w557:T1)
            n282 = Bundle By Name(cluster=w559, "state"=w557) -> (w560:T6)
            n283 = Enqueue Element(queue=w561, element=w560) -> ()  [unwired: 2 in, 3 out]
          }
          frame "chk_1M_list_flg" {
            # "Check to see if there is any resistor to measure\nin the 1M ohm range list.  If not, check the\n10M ohm list."
            n284 = Unbundle By Name(w565) -> ("list_flag"=w564:bool[])
            n285 = Index Array(array=w564, index=4) -> (element=w563:bool)
            n286 = Select(t=state_cntrl."set_1M_ohm_chnl_list", s=w563, f=state_cntrl."chk_10M_list_flg") -> (s? t:f=w567:T1)
            n287 = Bundle By Name(cluster=w569, "state"=w567) -> (w570:T6)
            n288 = Enqueue Element(queue=w571, element=w570) -> ()  [unwired: 2 in, 3 out]
          }
          frame "chk_10M_list_flg" {
            # "Check to see if there is any resistor to measure\nin the 10M ohm range list.  If not, it must be\nfor the 100M ohm range."
            n289 = Unbundle By Name(w575) -> ("list_flag"=w574:bool[])
            n290 = Index Array(array=w574, index=5) -> (element=w573:bool)
            n291 = Select(t=state_cntrl."set_10M_ohm_chnl_list", s=w573, f=state_cntrl."set_100M_ohm_chnl_list") -> (s? t:f=w577:T1)
            n292 = Bundle By Name(cluster=w579, "state"=w577) -> (w580:T6)
            n293 = Enqueue Element(queue=w581, element=w580) -> ()  [unwired: 2 in, 3 out]
          }
          frame "set_100_ohm_chnl_list" {
            # "configure for 100 ohm range"
            # "array of 100 ohm range indexes"
            # "Go through the 100 ohm ch list index array\nand pull out the slot # and ch # to form the\nchannel list."
            n294 = Unbundle By Name(w585) -> ("ch_list_indx_100"=w589:i32[], "res_table"=w588:dbl[][])
            n295 = for {
              N -> [w602]
              tunnel: w589 -> [w612] mode=indexing
              tunnel: w588 -> [w613]
              shift-right: [w593] -> w584
              shift-left: "" -> [w595]
              i -> [w600]
              # "don't add a comma if\nwe're at the last channel"
              # "slot #\nch #"
              n296 = Decrement(x=w602) -> (x-1=w601:i32)
              n297 = Index Array(array=w613, index (row)=w612) -> (element=w611:dbl[])  [unwired: 1 in]
              n298 = Equal?(x=w601, y=w600) -> (x = y?=w599:bool)
              n299 = Index Array(array=w611) -> (element #1=w610:dbl, element #2=w609:dbl)  [unwired: 2 in]
              n300 = To Long Integer(number=w610) -> (32bit integer=w608:i32)
              n301 = To Long Integer(number=w609) -> (32bit integer=w604:i32)
              n302 = Number To Decimal String(number=w608, width (-)=i16 1) -> (decimal integer string=w606:string)
              n303 = Format Value(format string="%03d", value (0)=w604) -> (output string=w605:string)  [unwired: 1 in]
              n304 = Select(t="", s=w599, f="," ("string")) -> (s? t:f=w596:string)
              n305 = Concatenate Strings(w606, w605, w596) -> (w594:string)
              n306 = Concatenate Strings(w595, w594) -> (w593:string)
            }
            "ch_list_str" <- w584
            n307 = Bundle By Name(cluster=w585, "range"=T4."100 Ohm", "100_ch_list_str"=w584) -> (w583:T7)
            n308 = Bundle By Name(cluster=w590, "state"=state_cntrl."conf_wire_mode") -> (w591:T6)
            n309 = Enqueue Element(queue=w592, element=w591) -> ()  [unwired: 2 in, 3 out]
          }
          frame "set_1K_ohm_chnl_list" {
            # "configure for 1K ohm range"
            # "array of 1K ohm range indexes"
            # "Go through the 1K ohm ch list index array\nand pull out the slot # and ch # to form the\nchannel list."
            n310 = Unbundle By Name(w617) -> ("ch_list_indx_1K"=w621:i32[], "res_table"=w620:dbl[][])
            n311 = for {
              N -> [w634]
              tunnel: w621 -> [w644] mode=indexing
              tunnel: w620 -> [w645]
              shift-right: [w625] -> w614
              shift-left: "" -> [w627]
              i -> [w632]
              # "don't add a comma if\nwe're at the last channel"
              # "slot #\nch #"
              n312 = Decrement(x=w634) -> (x-1=w633:i32)
              n313 = Index Array(array=w645, index (row)=w644) -> (element=w643:dbl[])  [unwired: 1 in]
              n314 = Equal?(x=w633, y=w632) -> (x = y?=w631:bool)
              n315 = Index Array(array=w643) -> (element #1=w642:dbl, element #2=w641:dbl)  [unwired: 2 in]
              n316 = To Long Integer(number=w642) -> (32bit integer=w640:i32)
              n317 = To Long Integer(number=w641) -> (32bit integer=w636:i32)
              n318 = Number To Decimal String(number=w640, width (-)=i16 1) -> (decimal integer string=w638:string)
              n319 = Format Value(format string="%03d", value (0)=w636) -> (output string=w637:string)  [unwired: 1 in]
              n320 = Select(t="", s=w631, f="," ("string")) -> (s? t:f=w628:string)
              n321 = Concatenate Strings(w638, w637, w628) -> (w626:string)
              n322 = Concatenate Strings(w627, w626) -> (w625:string)
            }
            n323 = local write "ch_list_str"(w614) -> ()
            n324 = Bundle By Name(cluster=w617, "range"=T4."1 kOhm", "1K_ch_list_str"=w614) -> (w616:T7)
            n325 = Bundle By Name(cluster=w622, "state"=state_cntrl."conf_wire_mode") -> (w623:T6)
            n326 = Enqueue Element(queue=w624, element=w623) -> ()  [unwired: 2 in, 3 out]
          }
          frame "set_10K_ohm_chnl_list" {
            # "configure for 10K ohm range"
            # "array of 10K ohm range indexes"
            # "Go through the 10K ohm ch list index array\nand pull out the slot # and ch # to form the\nchannel list."
            n327 = Unbundle By Name(w649) -> ("ch_list_indx_10K"=w653:i32[], "res_table"=w652:dbl[][])
            n328 = for {
              N -> [w666]
              tunnel: w653 -> [w676] mode=indexing
              tunnel: w652 -> [w677]
              shift-right: [w657] -> w647
              shift-left: "" -> [w659]
              i -> [w664]
              # "don't add a comma if\nwe're at the last channel"
              # "slot #\nch #"
              n329 = Decrement(x=w666) -> (x-1=w665:i32)
              n330 = Index Array(array=w677, index (row)=w676) -> (element=w675:dbl[])  [unwired: 1 in]
              n331 = Equal?(x=w665, y=w664) -> (x = y?=w663:bool)
              n332 = Index Array(array=w675) -> (element #1=w674:dbl, element #2=w673:dbl)  [unwired: 2 in]
              n333 = To Long Integer(number=w674) -> (32bit integer=w672:i32)
              n334 = To Long Integer(number=w673) -> (32bit integer=w668:i32)
              n335 = Number To Decimal String(number=w672, width (-)=i16 1) -> (decimal integer string=w670:string)
              n336 = Format Value(format string="%03d", value (0)=w668) -> (output string=w669:string)  [unwired: 1 in]
              n337 = Select(t="", s=w663, f="," ("string")) -> (s? t:f=w660:string)
              n338 = Concatenate Strings(w670, w669, w660) -> (w658:string)
              n339 = Concatenate Strings(w659, w658) -> (w657:string)
            }
            n340 = local write "ch_list_str"(w647) -> ()
            n341 = Bundle By Name(cluster=w649, "range"=T4."10 kOhm", "10K_ch_list_str"=w647) -> (w648:T7)
            n342 = Bundle By Name(cluster=w654, "state"=state_cntrl."conf_wire_mode") -> (w655:T6)
            n343 = Enqueue Element(queue=w656, element=w655) -> ()  [unwired: 2 in, 3 out]
          }
          frame "set_100K_ohm_chnl_list" {
            # "configure for 100K ohm range"
            # "array of 100K ohm range indexes"
            # "Go through the 100K ohm ch list index array\nand pull out the slot # and ch # to form the\nchannel list."
            n344 = Unbundle By Name(w681) -> ("ch_list_indx_100K"=w685:i32[], "res_table"=w684:dbl[][])
            n345 = for {
              N -> [w698]
              tunnel: w685 -> [w708] mode=indexing
              tunnel: w684 -> [w709]
              shift-right: [w689] -> w678
              shift-left: "" -> [w691]
              i -> [w696]
              # "don't add a comma if\nwe're at the last channel"
              # "slot #\nch #"
              n346 = Decrement(x=w698) -> (x-1=w697:i32)
              n347 = Index Array(array=w709, index (row)=w708) -> (element=w707:dbl[])  [unwired: 1 in]
              n348 = Equal?(x=w697, y=w696) -> (x = y?=w695:bool)
              n349 = Index Array(array=w707) -> (element #1=w706:dbl, element #2=w705:dbl)  [unwired: 2 in]
              n350 = To Long Integer(number=w706) -> (32bit integer=w704:i32)
              n351 = To Long Integer(number=w705) -> (32bit integer=w700:i32)
              n352 = Number To Decimal String(number=w704, width (-)=i16 1) -> (decimal integer string=w702:string)
              n353 = Format Value(format string="%03d", value (0)=w700) -> (output string=w701:string)  [unwired: 1 in]
              n354 = Select(t="", s=w695, f="," ("string")) -> (s? t:f=w692:string)
              n355 = Concatenate Strings(w702, w701, w692) -> (w690:string)
              n356 = Concatenate Strings(w691, w690) -> (w689:string)
            }
            n357 = local write "ch_list_str"(w678) -> ()
            n358 = Bundle By Name(cluster=w681, "range"=T4."100 kOhm", "100K_ch_list_str"=w678) -> (w680:T7)
            n359 = Bundle By Name(cluster=w686, "state"=state_cntrl."conf_wire_mode") -> (w687:T6)
            n360 = Enqueue Element(queue=w688, element=w687) -> ()  [unwired: 2 in, 3 out]
          }
          frame "set_1M_ohm_chnl_list" {
            # "configure for 1M ohm range"
            # "array of 1M ohm range indexes"
            # "Go through the 1M ohm ch list index array\nand pull out the slot # and ch # to form the\nchannel list."
            n361 = Unbundle By Name(w713) -> ("ch_list_indx_1M"=w717:i32[], "res_table"=w716:dbl[][])
            n362 = for {
              N -> [w730]
              tunnel: w717 -> [w740] mode=indexing
              tunnel: w716 -> [w741]
              shift-right: [w721] -> w710
              shift-left: "" -> [w723]
              i -> [w728]
              # "don't add a comma if\nwe're at the last channel"
              # "slot #\nch #"
              n363 = Decrement(x=w730) -> (x-1=w729:i32)
              n364 = Index Array(array=w741, index (row)=w740) -> (element=w739:dbl[])  [unwired: 1 in]
              n365 = Equal?(x=w729, y=w728) -> (x = y?=w727:bool)
              n366 = Index Array(array=w739) -> (element #1=w738:dbl, element #2=w737:dbl)  [unwired: 2 in]
              n367 = To Long Integer(number=w738) -> (32bit integer=w736:i32)
              n368 = To Long Integer(number=w737) -> (32bit integer=w732:i32)
              n369 = Number To Decimal String(number=w736, width (-)=i16 1) -> (decimal integer string=w734:string)
              n370 = Format Value(format string="%03d", value (0)=w732) -> (output string=w733:string)  [unwired: 1 in]
              n371 = Select(t="", s=w727, f="," ("string")) -> (s? t:f=w724:string)
              n372 = Concatenate Strings(w734, w733, w724) -> (w722:string)
              n373 = Concatenate Strings(w723, w722) -> (w721:string)
            }
            n374 = local write "ch_list_str"(w710) -> ()
            n375 = Bundle By Name(cluster=w713, "range"=T4."1 MOhm", "1M_ch_list_str"=w710) -> (w712:T7)
            n376 = Bundle By Name(cluster=w718, "state"=state_cntrl."conf_wire_mode") -> (w719:T6)
            n377 = Enqueue Element(queue=w720, element=w719) -> ()  [unwired: 2 in, 3 out]
          }
          frame "set_10M_ohm_chnl_list" {
            # "configure for 10M ohm range"
            # "array of 10M ohm range indexes"
            # "Go through the 10M ohm ch list index array\nand pull out the slot # and ch # to form the\nchannel list."
            n378 = Unbundle By Name(w745) -> ("ch_list_indx_10M"=w749:i32[], "res_table"=w748:dbl[][])
            n379 = for {
              N -> [w762]
              tunnel: w749 -> [w772] mode=indexing
              tunnel: w748 -> [w773]
              shift-right: [w753] -> w742
              shift-left: "" -> [w755]
              i -> [w760]
              # "don't add a comma if\nwe're at the last channel"
              # "slot #\nch #"
              n380 = Decrement(x=w762) -> (x-1=w761:i32)
              n381 = Index Array(array=w773, index (row)=w772) -> (element=w771:dbl[])  [unwired: 1 in]
              n382 = Equal?(x=w761, y=w760) -> (x = y?=w759:bool)
              n383 = Index Array(array=w771) -> (element #1=w770:dbl, element #2=w769:dbl)  [unwired: 2 in]
              n384 = To Long Integer(number=w770) -> (32bit integer=w768:i32)
              n385 = To Long Integer(number=w769) -> (32bit integer=w764:i32)
              n386 = Number To Decimal String(number=w768, width (-)=i16 1) -> (decimal integer string=w766:string)
              n387 = Format Value(format string="%03d", value (0)=w764) -> (output string=w765:string)  [unwired: 1 in]
              n388 = Select(t="", s=w759, f="," ("string")) -> (s? t:f=w756:string)
              n389 = Concatenate Strings(w766, w765, w756) -> (w754:string)
              n390 = Concatenate Strings(w755, w754) -> (w753:string)
            }
            n391 = local write "ch_list_str"(w742) -> ()
            n392 = Bundle By Name(cluster=w745, "range"=T4."10 MOhm", "10M_ch_list_str"=w742) -> (w744:T7)
            n393 = Bundle By Name(cluster=w750, "state"=state_cntrl."conf_wire_mode") -> (w751:T6)
            n394 = Enqueue Element(queue=w752, element=w751) -> ()  [unwired: 2 in, 3 out]
          }
          frame "set_100M_ohm_chnl_list" {
            # "configure for 100M ohm range"
            # "array of 100M ohm range indexes"
            # "Go through the 100M ohm ch list index array\nand pull out the slot # and ch # to form the\nchannel list."
            n395 = Unbundle By Name(w777) -> ("ch_list_indx_100M"=w781:i32[], "res_table"=w780:dbl[][])
            n396 = for {
              N -> [w794]
              tunnel: w781 -> [w804] mode=indexing
              tunnel: w780 -> [w805]
              shift-right: [w785] -> w774
              shift-left: "" -> [w787]
              i -> [w792]
              # "don't add a comma if\nwe're at the last channel"
              # "slot #\nch #"
              n397 = Decrement(x=w794) -> (x-1=w793:i32)
              n398 = Index Array(array=w805, index (row)=w804) -> (element=w803:dbl[])  [unwired: 1 in]
              n399 = Equal?(x=w793, y=w792) -> (x = y?=w791:bool)
              n400 = Index Array(array=w803) -> (element #1=w802:dbl, element #2=w801:dbl)  [unwired: 2 in]
              n401 = To Long Integer(number=w802) -> (32bit integer=w800:i32)
              n402 = To Long Integer(number=w801) -> (32bit integer=w796:i32)
              n403 = Number To Decimal String(number=w800, width (-)=i16 1) -> (decimal integer string=w798:string)
              n404 = Format Value(format string="%03d", value (0)=w796) -> (output string=w797:string)  [unwired: 1 in]
              n405 = Select(t="", s=w791, f="," ("string")) -> (s? t:f=w788:string)
              n406 = Concatenate Strings(w798, w797, w788) -> (w786:string)
              n407 = Concatenate Strings(w787, w786) -> (w785:string)
            }
            n408 = local write "ch_list_str"(w774) -> ()
            n409 = Bundle By Name(cluster=w777, "range"=T4."100 MOhm", "100M_ch_list_str"=w774) -> (w776:T7)
            n410 = Bundle By Name(cluster=w782, "state"=state_cntrl."conf_wire_mode") -> (w783:T6)
            n411 = Enqueue Element(queue=w784, element=w783) -> ()  [unwired: 2 in, 3 out]
          }
          frame "conf_wire_mode" {
            # "This state configure the switch for a 4 wire\nresistance test."
            n412 = Unbundle By Name(w807) -> ("100_ch_list_str"=w817:string, "1K_ch_list_str"=w816:string, "10K_ch_list_str"=w815:string, "100K_ch_list_str"=w814:string, "1M_ch_list_str"=w813:string, "10M_ch_list_str"=w812:string, "100M_ch_list_str"=w811:string, "range"=w809:T4)
            n413 = local read "res"() -> (w818:T5)
            n414 = Build Array(w817, w816, w815, w814, w813, w812, w811) -> (w810:string[])
            n415 = Index Array(array=w810, index=w809) -> (element=w808:string)
            n416 = call <instrlib>:"AG34980A Configure 4-Wire Resistance.vi"("VISA resource name"=w819, "Channel List(empty)"=w808, "Resolution (5:Default)"=w818) -> ("error out"=w806:errorcluster)  [unwired: 11 in, 1 out]
            n417 = Bundle By Name(cluster=w821, "state"=state_cntrl."conf_trig_type") -> (w822:T6)
            n418 = Enqueue Element(queue=w823, element=w822, error in (no error)=w806) -> ()  [unwired: 1 in, 3 out]
          }
          frame "conf_trig_type" {
            # "This state sets up the trigger source."
            n419 = local read "trig_src"() -> (w824:T3)
            n420 = Bundle By Name(cluster=w829, "state"=state_cntrl."start_scan") -> (w830:T6)
            n421 = call <instrlib>:"AG34980A Configure Trigger.vi"("VISA resource name"=w827, "Trigger Source (1:Immediate)"=w824) -> ("error out"=w825:errorcluster)  [unwired: 12 in, 1 out]
            n422 = Enqueue Element(queue=w831, element=w830, error in (no error)=w825) -> ()  [unwired: 1 in, 3 out]
          }
          frame "start_scan" {
            # "This state sets the scan for the channels list."
            n423 = Unbundle By Name(w833) -> ("100_ch_list_str"=w843:string, "1K_ch_list_str"=w842:string, "10K_ch_list_str"=w841:string, "100K_ch_list_str"=w840:string, "1M_ch_list_str"=w839:string, "10M_ch_list_str"=w838:string, "100M_ch_list_str"=w837:string, "range"=w835:T4)
            n424 = Build Array(w843, w842, w841, w840, w839, w838, w837) -> (w836:string[])
            n425 = Index Array(array=w836, index=w835) -> (element=w834:string)
            n426 = call <instrlib>:"AG34980A Configure Scan.vi"("VISA resource name"=w844, "Scan List(empty)"=w834) -> ("error out"=w832:errorcluster)  [unwired: 12 in, 1 out]
            n427 = Bundle By Name(cluster=w846, "state"=state_cntrl."scan_cancel_qry") -> (w847:T6)
            n428 = Enqueue Element(queue=w848, element=w847, error in (no error)=w832) -> ()  [unwired: 1 in, 3 out]
          }
          frame "scan_cancel_qry" {
            # "If the start button is still pressed,\ncontinue with the measurement.\nElse, clear all flags and quit."
            # "This state check if we need to cancel the measurment."
            n429 = property on="start" class="Bool (strict)"() -> ("Value"=w849:bool)  [unwired: 2 in, 2 out]
            n430 = Select(t=state_cntrl."init_meas" ("state"), s=w849, f=state_cntrl."initialize") -> (s? t:f=w850:T1)
            n431 = Bundle By Name(cluster=w854, "state"=w850) -> (w855:T6)
            n432 = Enqueue Element(queue=w856, element=w855) -> ()  [unwired: 2 in, 3 out]
          }
          frame "init_meas" {
            # "Put the switch into the \"wait-for-trigger\" mode.\nOnce the trigger happens, the internal DMM will\ntake the measurement.  We are using the\nimmediate trigger, so the measurment should\nhappens right away."
            n433 = call <instrlib>:"AG34980A Initiate.vi"("VISA resource name"=w859) -> ("error out"=w857:errorcluster)  [unwired: 13 in, 1 out]
            n434 = Bundle By Name(cluster=w861, "state"=state_cntrl."done_meas_qry") -> (w862:T6)
            n435 = Enqueue Element(queue=w863, element=w862, error in (no error)=w857) -> ()  [unwired: 1 in, 3 out]
          }
          frame "done_meas_qry" {
            # "We will check if the switch has the\nmeasurments ready."
            n436 = while {
              tunnel: w866 -> [w883]
              tunnel: [w871] -> w864
              stop <- w876 stop-if-true
              # "We will stop querying if the switch\nhas all the data ready or we cancel\nthe test."
              n437 = call "AG34980A_Status_Oper_Cond.vi"("VISA resource name"=w883) -> ("resp"=w882:string, "error out"=w871:errorcluster)  [unwired: 12 in, 1 out]
              n438 = String Subset(string=w882, offset (0)=1, length (rest)=3 ("length (rest)")) -> (substring=w875:string)
              n439 = Decimal String To Number(string=w875) -> (number=w881:i32)  [unwired: 2 in, 1 out]
              n440 = local read "start"() -> (w872:bool)
              n441 = Equal?(x=w881, y=512) -> (x = y?=w878:bool)
              n442 = Equal?(x=FALSE ("stop"), y=w872) -> (x = y?=w877:bool)
              n443 = Or(x=w878, y=w877) -> (x .or. y?=w876:bool)
            }
            n444 = Bundle By Name(cluster=w868, "state"=state_cntrl."fetch_data") -> (w869:T6)
            n445 = Enqueue Element(queue=w870, element=w869, error in (no error)=w864) -> ()  [unwired: 1 in, 3 out]
          }
          frame "fetch_data" {
            # "Clear out the flag as we finish\neach range.  Also, count down\nthe channel list count that we\nhad to measure."
            # "This state sets up the trigger source."
            n446 = Unbundle By Name(w893) -> ("list_flag"=w890:bool[], "range"=w891:T4, "ch_list_set_cnt"=w895:i32)
            n447 = local read "byte_count"() -> (w896:i32)
            n448 = case shown="\"10 kOhm\"" w891 {
              selector: w891 -> [w905 w909 w913 w917 w921 w925 w929]
              tunnel: w890 -> [w906 w910 w914 w918 w922 w926 w930]
              tunnel: FALSE ("new element/subarray") -> [w904 w908 w912 w916 w920 w924 w928]
              tunnel: [w903 w907 w911 w915 w919 w923 w927] -> w888
              frame "100 Ohm", Default {
                n449 = Replace Array Subset(array=w906, new element=w904, index=w905) -> (w903:bool[])
              }
              frame "1 kOhm" {
                n450 = Replace Array Subset(array=w910, new element=w908, index=w909) -> (w907:bool[])
              }
              frame "10 kOhm" {
                n451 = Replace Array Subset(array=w914, new element=w912, index=w913) -> (w911:bool[])
              }
              frame "100 kOhm" {
                n452 = Replace Array Subset(array=w918, new element=w916, index=w917) -> (w915:bool[])
              }
              frame "1 MOhm" {
                n453 = Replace Array Subset(array=w922, new element=w920, index=w921) -> (w919:bool[])
              }
              frame "10 MOhm" {
                n454 = Replace Array Subset(array=w926, new element=w924, index=w925) -> (w923:bool[])
              }
              frame "100 MOhm" {
                n455 = Replace Array Subset(array=w930, new element=w928, index=w929) -> (w927:bool[])
              }
            }
            n456 = Decrement(x=w895) -> (x-1=w894:i32)
            n457 = Bundle By Name(cluster=w900, "state"=state_cntrl."fill_data_table") -> (w901:T6)
            n458 = call <instrlib>:"AG34980A Fetch.vi"("VISA resource name"=w898, "Numbers Only (T:On)"=TRUE, "Byte Count (1024 bytes)"=w896) -> ("Output Data (Numbers Only)"=w887:dbl[], "error out"=w897:errorcluster)  [unwired: 9 in, 2 out]
            n459 = Number To Fractional String(number=w887, precision (6)=i16 2) -> (F-format string=w886:string[])  [unwired: 2 in]
            n460 = Enqueue Element(queue=w902, element=w901, error in (no error)=w897) -> ()  [unwired: 1 in, 3 out]
            n461 = local write "scan_data"(w886) -> ()
            n462 = Bundle By Name(cluster=w893, "scan_data"=w886, "list_flag"=w888, "ch_list_set_cnt"=w894) -> (w892:T7)
          }
          frame "fill_data_table" {
            # "Fill out the data table with the\nmeasured resistances."
            # "If we know the range we are doing,\nwe can pull out the row indexes from\nthe corresponding ch_list_indx_X."
            n463 = Unbundle By Name(w933) -> ("res_table_text"=w934:string[][], "ch_list_indx_100"=w942:i32[], "ch_list_indx_1K"=w941:i32[], "ch_list_indx_10K"=w940:i32[], "ch_list_indx_100K"=w939:i32[], "ch_list_indx_1M"=w938:i32[], "ch_list_indx_10M"=w937:i32[], "ch_list_indx_100M"=w936:i32[], "range"=w943:T4, "scan_data"=w935:string[])
            n464 = case shown="\"10 kOhm\"" w943 {
              tunnel: w942 -> [w951 _ _]
              tunnel: w941 -> [_ w1728 _]
              tunnel: w940 -> [_ _ w2508]
              tunnel: w939 -> [_ _ _]
              tunnel: w938 -> [_ _ _]
              tunnel: w937 -> [_ _ _]
              tunnel: w936 -> [_ _ _]
              tunnel: w935 -> [w949 w1730 w2510]
              tunnel: w934 -> [w950 w1731 w2511]
              tunnel: [w948 w1729 w2509] -> w931
              frame "100 Ohm", Default {
                n465 = for {
                  tunnel: w951 -> [w957] mode=indexing
                  tunnel: w949 -> [w955]
                  shift-right: [w953] -> w948
                  shift-left: w950 -> [w956]
                  i -> [w952]
                  # "34924A has a \nmax of 35 \nchannels."
                  n466 = Index Array(array=w955, index=w952) -> (element=w954:string)
                  n467 = case shown="0, Default" w957 {
                    selector: w957 -> [w964 w986 w1008 w1030 w1052 w1074 w1096 w1118 w1140 w1162 w1184 w1206 w1228 w1250 w1272 w1294 w1316 w1338 w1360 w1382 w1404 w1426 w1448 w1470 w1492 w1514 w1536 w1558 w1580 w1602 w1624 w1646 w1668 w1690 w1712]
                    tunnel: w956 -> [w978 w1000 w1022 w1044 w1066 w1088 w1110 w1132 w1154 w1176 w1198 w1220 w1242 w1264 w1286 w1308 w1330 w1352 w1374 w1396 w1418 w1440 w1462 w1484 w1506 w1528 w1550 w1572 w1594 w1616 w1638 w1660 w1682 w1704 w1726]
                    tunnel: w954 -> [w971 w993 w1015 w1037 w1059 w1081 w1103 w1125 w1147 w1169 w1191 w1213 w1235 w1257 w1279 w1301 w1323 w1345 w1367 w1389 w1411 w1433 w1455 w1477 w1499 w1521 w1543 w1565 w1587 w1609 w1631 w1653 w1675 w1697 w1719]
                    tunnel: [w961 w983 w1005 w1027 w1049 w1071 w1093 w1115 w1137 w1159 w1181 w1203 w1225 w1247 w1269 w1291 w1313 w1335 w1357 w1379 w1401 w1423 w1445 w1467 w1489 w1511 w1533 w1555 w1577 w1599 w1621 w1643 w1665 w1687 w1709] -> w953
                    frame 0, Default {
                      w976 = 3  # tol
                      w977 = 2  # res
                      w979 = 4  # meas
                      # "fill the P/F\ncol"
                      # "fill the meas col"
                      # "check to see\npass or fail"
                      # "pull out resistor\nvalue and tolerance\nto find limits"
                      n468 = Index Array(array=w978, index (row) #1=w964, index (col) #1=w977, index (row) #2=w964, index (col) #2=w976) -> (element #1=w975:string, element #2=w974:string)
                      n469 = Fract/Exp String To Number(string=w975) -> (number=w959:dbl)  [unwired: 3 in, 1 out]
                      n470 = Fract/Exp String To Number(string=w974) -> (number=w973:dbl)  [unwired: 3 in, 1 out]
                      n471 = Fract/Exp String To Number(string=w971) -> (number=w968:dbl)  [unwired: 3 in, 1 out]
                      n472 = Divide(x=w973, y=100.0) -> (x/y=w960:dbl)
                      n473 = Multiply(x=w960, y=w959) -> (x*y=w958:dbl)
                      n474 = Add(x=w959, y=w958) -> (x+y=w970:dbl)
                      n475 = Subtract(x=w959, y=w958) -> (x-y=w969:dbl)
                      n476 = In Range and Coerce(upper limit=w970, x=w968, lower limit=w969) -> (In Range?=w967:bool)  [unwired: 1 out]
                      n477 = Select(t="P", s=w967, f="F") -> (s? t:f=w962:string)
                      n478 = Replace Array Subset(array=w978, new element #1=w971, index (row) #1=w964, index (col) #1=w979, new element #2=w962, index (row) #2=w964, index (col) #2=5 ("disabled index (col)")) -> (w961:string[][])
                    }
                    frame 1 {
                      w998 = 3  # tol
                      w999 = 2  # res
                      w1001 = 4  # meas
                      # "fill the P/F\ncol"
                      # "fill the meas col"
                      # "check to see\npass or fail"
                      # "pull out resistor\nvalue and tolerance\nto find limits"
                      n479 = Index Array(array=w1000, index (row) #1=w986, index (col) #1=w999, index (row) #2=w986, index (col) #2=w998) -> (element #1=w997:string, element #2=w996:string)
                      n480 = Fract/Exp String To Number(string=w997) -> (number=w981:dbl)  [unwired: 3 in, 1 out]
                      n481 = Fract/Exp String To Number(string=w996) -> (number=w995:dbl)  [unwired: 3 in, 1 out]
                      n482 = Fract/Exp String To Number(string=w993) -> (number=w990:dbl)  [unwired: 3 in, 1 out]
                      n483 = Divide(x=w995, y=100.0) -> (x/y=w982:dbl)
                      n484 = Multiply(x=w982, y=w981) -> (x*y=w980:dbl)
                      n485 = Add(x=w981, y=w980) -> (x+y=w992:dbl)
                      n486 = Subtract(x=w981, y=w980) -> (x-y=w991:dbl)
                      n487 = In Range and Coerce(upper limit=w992, x=w990, lower limit=w991) -> (In Range?=w989:bool)  [unwired: 1 out]
                      n488 = Select(t="P", s=w989, f="F") -> (s? t:f=w984:string)
                      n489 = Replace Array Subset(array=w1000, new element #1=w993, index (row) #1=w986, index (col) #1=w1001, new element #2=w984, index (row) #2=w986, index (col) #2=5 ("disabled index (col)")) -> (w983:string[][])
                    }
                    frame 2 {
                      w1020 = 3  # tol
                      w1021 = 2  # res
                      w1023 = 4  # meas
                      # "fill the P/F\ncol"
                      # "fill the meas col"
                      # "check to see\npass or fail"
                      # "pull out resistor\nvalue and tolerance\nto find limits"
                      n490 = Index Array(array=w1022, index (row) #1=w1008, index (col) #1=w1021, index (row) #2=w1008, index (col) #2=w1020) -> (element #1=w1019:string, element #2=w1018:string)
                      n491 = Fract/Exp String To Number(string=w1019) -> (number=w1003:dbl)  [unwired: 3 in, 1 out]
                      n492 = Fract/Exp String To Number(string=w1018) -> (number=w1017:dbl)  [unwired: 3 in, 1 out]
                      n493 = Fract/Exp String To Number(string=w1015) -> (number=w1012:dbl)  [unwired: 3 in, 1 out]
                      n494 = Divide(x=w1017, y=100.0) -> (x/y=w1004:dbl)
                      n495 = Multiply(x=w1004, y=w1003) -> (x*y=w1002:dbl)
                      n496 = Add(x=w1003, y=w1002) -> (x+y=w1014:dbl)
                      n497 = Subtract(x=w1003, y=w1002) -> (x-y=w1013:dbl)
                      n498 = In Range and Coerce(upper limit=w1014, x=w1012, lower limit=w1013) -> (In Range?=w1011:bool)  [unwired: 1 out]
                      n499 = Select(t="P", s=w1011, f="F") -> (s? t:f=w1006:string)
                      n500 = Replace Array Subset(array=w1022, new element #1=w1015, index (row) #1=w1008, index (col) #1=w1023, new element #2=w1006, index (row) #2=w1008, index (col) #2=5 ("disabled index (col)")) -> (w1005:string[][])
                    }
                    frame 3 {
                      w1042 = 3  # tol
                      w1043 = 2  # res
                      w1045 = 4  # meas
                      # "fill the P/F\ncol"
                      # "fill the meas col"
                      # "check to see\npass or fail"
                      # "pull out resistor\nvalue and tolerance\nto find limits"
                      n501 = Index Array(array=w1044, index (row) #1=w1030, index (col) #1=w1043, index (row) #2=w1030, index (col) #2=w1042) -> (element #1=w1041:string, element #2=w1040:string)
                      n502 = Fract/Exp String To Number(string=w1041) -> (number=w1025:dbl)  [unwired: 3 in, 1 out]
                      n503 = Fract/Exp String To Number(string=w1040) -> (number=w1039:dbl)  [unwired: 3 in, 1 out]
                      n504 = Fract/Exp String To Number(string=w1037) -> (number=w1034:dbl)  [unwired: 3 in, 1 out]
                      n505 = Divide(x=w1039, y=100.0) -> (x/y=w1026:dbl)
                      n506 = Multiply(x=w1026, y=w1025) -> (x*y=w1024:dbl)
                      n507 = Add(x=w1025, y=w1024) -> (x+y=w1036:dbl)
                      n508 = Subtract(x=w1025, y=w1024) -> (x-y=w1035:dbl)
                      n509 = In Range and Coerce(upper limit=w1036, x=w1034, lower limit=w1035) -> (In Range?=w1033:bool)  [unwired: 1 out]
                      n510 = Select(t="P", s=w1033, f="F") -> (s? t:f=w1028:string)
                      n511 = Replace Array Subset(array=w1044, new element #1=w1037, index (row) #1=w1030, index (col) #1=w1045, new element #2=w1028, index (row) #2=w1030, index (col) #2=5 ("disabled index (col)")) -> (w1027:string[][])
                    }
                    frame 4 {
                      w1064 = 3  # tol
                      w1065 = 2  # res
                      w1067 = 4  # meas
                      # "fill the P/F\ncol"
                      # "fill the meas col"
                      # "check to see\npass or fail"
                      # "pull out resistor\nvalue and tolerance\nto find limits"
                      n512 = Index Array(array=w1066, index (row) #1=w1052, index (col) #1=w1065, index (row) #2=w1052, index (col) #2=w1064) -> (element #1=w1063:string, element #2=w1062:string)
                      n513 = Fract/Exp String To Number(string=w1063) -> (number=w1047:dbl)  [unwired: 3 in, 1 out]
                      n514 = Fract/Exp String To Number(string=w1062) -> (number=w1061:dbl)  [unwired: 3 in, 1 out]
                      n515 = Fract/Exp String To Number(string=w1059) -> (number=w1056:dbl)  [unwired: 3 in, 1 out]
                      n516 = Divide(x=w1061, y=100.0) -> (x/y=w1048:dbl)
                      n517 = Multiply(x=w1048, y=w1047) -> (x*y=w1046:dbl)
                      n518 = Add(x=w1047, y=w1046) -> (x+y=w1058:dbl)
                      n519 = Subtract(x=w1047, y=w1046) -> (x-y=w1057:dbl)
                      n520 = In Range and Coerce(upper limit=w1058, x=w1056, lower limit=w1057) -> (In Range?=w1055:bool)  [unwired: 1 out]
                      n521 = Select(t="P", s=w1055, f="F") -> (s? t:f=w1050:string)
                      n522 = Replace Array Subset(array=w1066, new element #1=w1059, index (row) #1=w1052, index (col) #1=w1067, new element #2=w1050, index (row) #2=w1052, index (col) #2=5 ("disabled index (col)")) -> (w1049:string[][])
                    }
                    frame 5 {
                      w1086 = 3  # tol
                      w1087 = 2  # res
                      w1089 = 4  # meas
                      # "fill the P/F\ncol"
                      # "fill the meas col"
                      # "check to see\npass or fail"
                      # "pull out resistor\nvalue and tolerance\nto find limits"
                      n523 = Index Array(array=w1088, index (row) #1=w1074, index (col) #1=w1087, index (row) #2=w1074, index (col) #2=w1086) -> (element #1=w1085:string, element #2=w1084:string)
                      n524 = Fract/Exp String To Number(string=w1085) -> (number=w1069:dbl)  [unwired: 3 in, 1 out]
                      n525 = Fract/Exp String To Number(string=w1084) -> (number=w1083:dbl)  [unwired: 3 in, 1 out]
                      n526 = Fract/Exp String To Number(string=w1081) -> (number=w1078:dbl)  [unwired: 3 in, 1 out]
                      n527 = Divide(x=w1083, y=100.0) -> (x/y=w1070:dbl)
                      n528 = Multiply(x=w1070, y=w1069) -> (x*y=w1068:dbl)
                      n529 = Add(x=w1069, y=w1068) -> (x+y=w1080:dbl)
                      n530 = Subtract(x=w1069, y=w1068) -> (x-y=w1079:dbl)
                      n531 = In Range and Coerce(upper limit=w1080, x=w1078, lower limit=w1079) -> (In Range?=w1077:bool)  [unwired: 1 out]
                      n532 = Select(t="P", s=w1077, f="F") -> (s? t:f=w1072:string)
                      n533 = Replace Array Subset(array=w1088, new element #1=w1081, index (row) #1=w1074, index (col) #1=w1089, new element #2=w1072, index (row) #2=w1074, index (col) #2=5 ("disabled index (col)")) -> (w1071:string[][])
                    }
                    frame 6 {
                      w1108 = 3  # tol
                      w1109 = 2  # res
                      w1111 = 4  # meas
                      # "fill the P/F\ncol"
                      # "fill the meas col"
                      # "check to see\npass or fail"
                      # "pull out resistor\nvalue and tolerance\nto find limits"
                      n534 = Index Array(array=w1110, index (row) #1=w1096, index (col) #1=w1109, index (row) #2=w1096, index (col) #2=w1108) -> (element #1=w1107:string, element #2=w1106:string)
                      n535 = Fract/Exp String To Number(string=w1107) -> (number=w1091:dbl)  [unwired: 3 in, 1 out]
                      n536 = Fract/Exp String To Number(string=w1106) -> (number=w1105:dbl)  [unwired: 3 in, 1 out]
                      n537 = Fract/Exp String To Number(string=w1103) -> (number=w1100:dbl)  [unwired: 3 in, 1 out]
                      n538 = Divide(x=w1105, y=100.0) -> (x/y=w1092:dbl)
                      n539 = Multiply(x=w1092, y=w1091) -> (x*y=w1090:dbl)
                      n540 = Add(x=w1091, y=w1090) -> (x+y=w1102:dbl)
                      n541 = Subtract(x=w1091, y=w1090) -> (x-y=w1101:dbl)
                      n542 = In Range and Coerce(upper limit=w1102, x=w1100, lower limit=w1101) -> (In Range?=w1099:bool)  [unwired: 1 out]
                      n543 = Select(t="P", s=w1099, f="F") -> (s? t:f=w1094:string)
                      n544 = Replace Array Subset(array=w1110, new element #1=w1103, index (row) #1=w1096, index (col) #1=w1111, new element #2=w1094, index (row) #2=w1096, index (col) #2=5 ("disabled index (col)")) -> (w1093:string[][])
                    }
                    frame 7 {
                      w1130 = 3  # tol
                      w1131 = 2  # res
                      w1133 = 4  # meas
                      # "fill the P/F\ncol"
                      # "fill the meas col"
                      # "check to see\npass or fail"
                      # "pull out resistor\nvalue and tolerance\nto find limits"
                      n545 = Index Array(array=w1132, index (row) #1=w1118, index (col) #1=w1131, index (row) #2=w1118, index (col) #2=w1130) -> (element #1=w1129:string, element #2=w1128:string)
                      n546 = Fract/Exp String To Number(string=w1129) -> (number=w1113:dbl)  [unwired: 3 in, 1 out]
                      n547 = Fract/Exp String To Number(string=w1128) -> (number=w1127:dbl)  [unwired: 3 in, 1 out]
                      n548 = Fract/Exp String To Number(string=w1125) -> (number=w1122:dbl)  [unwired: 3 in, 1 out]
                      n549 = Divide(x=w1127, y=100.0) -> (x/y=w1114:dbl)
                      n550 = Multiply(x=w1114, y=w1113) -> (x*y=w1112:dbl)
                      n551 = Add(x=w1113, y=w1112) -> (x+y=w1124:dbl)
                      n552 = Subtract(x=w1113, y=w1112) -> (x-y=w1123:dbl)
                      n553 = In Range and Coerce(upper limit=w1124, x=w1122, lower limit=w1123) -> (In Range?=w1121:bool)  [unwired: 1 out]
                      n554 = Select(t="P", s=w1121, f="F") -> (s? t:f=w1116:string)
                      n555 = Replace Array Subset(array=w1132, new element #1=w1125, index (row) #1=w1118, index (col) #1=w1133, new element #2=w1116, index (row) #2=w1118, index (col) #2=5 ("disabled index (col)")) -> (w1115:string[][])
                    }
                    frame 8 {
                      w1152 = 3  # tol
                      w1153 = 2  # res
                      w1155 = 4  # meas
                      # "fill the P/F\ncol"
                      # "fill the meas col"
                      # "check to see\npass or fail"
                      # "pull out resistor\nvalue and tolerance\nto find limits"
                      n556 = Index Array(array=w1154, index (row) #1=w1140, index (col) #1=w1153, index (row) #2=w1140, index (col) #2=w1152) -> (element #1=w1151:string, element #2=w1150:string)
                      n557 = Fract/Exp String To Number(string=w1151) -> (number=w1135:dbl)  [unwired: 3 in, 1 out]
                      n558 = Fract/Exp String To Number(string=w1150) -> (number=w1149:dbl)  [unwired: 3 in, 1 out]
                      n559 = Fract/Exp String To Number(string=w1147) -> (number=w1144:dbl)  [unwired: 3 in, 1 out]
                      n560 = Divide(x=w1149, y=100.0) -> (x/y=w1136:dbl)
                      n561 = Multiply(x=w1136, y=w1135) -> (x*y=w1134:dbl)
                      n562 = Add(x=w1135, y=w1134) -> (x+y=w1146:dbl)
                      n563 = Subtract(x=w1135, y=w1134) -> (x-y=w1145:dbl)
                      n564 = In Range and Coerce(upper limit=w1146, x=w1144, lower limit=w1145) -> (In Range?=w1143:bool)  [unwired: 1 out]
                      n565 = Select(t="P", s=w1143, f="F") -> (s? t:f=w1138:string)
                      n566 = Replace Array Subset(array=w1154, new element #1=w1147, index (row) #1=w1140, index (col) #1=w1155, new element #2=w1138, index (row) #2=w1140, index (col) #2=5 ("disabled index (col)")) -> (w1137:string[][])
                    }
                    frame 9 {
                      w1174 = 3  # tol
                      w1175 = 2  # res
                      w1177 = 4  # meas
                      # "fill the P/F\ncol"
                      # "fill the meas col"
                      # "check to see\npass or fail"
                      # "pull out resistor\nvalue and tolerance\nto find limits"
                      n567 = Index Array(array=w1176, index (row) #1=w1162, index (col) #1=w1175, index (row) #2=w1162, index (col) #2=w1174) -> (element #1=w1173:string, element #2=w1172:string)
                      n568 = Fract/Exp String To Number(string=w1173) -> (number=w1157:dbl)  [unwired: 3 in, 1 out]
                      n569 = Fract/Exp String To Number(string=w1172) -> (number=w1171:dbl)  [unwired: 3 in, 1 out]
                      n570 = Fract/Exp String To Number(string=w1169) -> (number=w1166:dbl)  [unwired: 3 in, 1 out]
                      n571 = Divide(x=w1171, y=100.0) -> (x/y=w1158:dbl)
                      n572 = Multiply(x=w1158, y=w1157) -> (x*y=w1156:dbl)
                      n573 = Add(x=w1157, y=w1156) -> (x+y=w1168:dbl)
                      n574 = Subtract(x=w1157, y=w1156) -> (x-y=w1167:dbl)
                      n575 = In Range and Coerce(upper limit=w1168, x=w1166, lower limit=w1167) -> (In Range?=w1165:bool)  [unwired: 1 out]
                      n576 = Select(t="P", s=w1165, f="F") -> (s? t:f=w1160:string)
                      n577 = Replace Array Subset(array=w1176, new element #1=w1169, index (row) #1=w1162, index (col) #1=w1177, new element #2=w1160, index (row) #2=w1162, index (col) #2=5 ("disabled index (col)")) -> (w1159:string[][])
                    }
                    frame 10 {
                      w1196 = 3  # tol
                      w1197 = 2  # res
                      w1199 = 4  # meas
                      # "fill the P/F\ncol"
                      # "fill the meas col"
                      # "check to see\npass or fail"
                      # "pull out resistor\nvalue and tolerance\nto find limits"
                      n578 = Index Array(array=w1198, index (row) #1=w1184, index (col) #1=w1197, index (row) #2=w1184, index (col) #2=w1196) -> (element #1=w1195:string, element #2=w1194:string)
                      n579 = Fract/Exp String To Number(string=w1195) -> (number=w1179:dbl)  [unwired: 3 in, 1 out]
                      n580 = Fract/Exp String To Number(string=w1194) -> (number=w1193:dbl)  [unwired: 3 in, 1 out]
                      n581 = Fract/Exp String To Number(string=w1191) -> (number=w1188:dbl)  [unwired: 3 in, 1 out]
                      n582 = Divide(x=w1193, y=100.0) -> (x/y=w1180:dbl)
                      n583 = Multiply(x=w1180, y=w1179) -> (x*y=w1178:dbl)
                      n584 = Add(x=w1179, y=w1178) -> (x+y=w1190:dbl)
                      n585 = Subtract(x=w1179, y=w1178) -> (x-y=w1189:dbl)
                      n586 = In Range and Coerce(upper limit=w1190, x=w1188, lower limit=w1189) -> (In Range?=w1187:bool)  [unwired: 1 out]
                      n587 = Select(t="P", s=w1187, f="F") -> (s? t:f=w1182:string)
                      n588 = Replace Array Subset(array=w1198, new element #1=w1191, index (row) #1=w1184, index (col) #1=w1199, new element #2=w1182, index (row) #2=w1184, index (col) #2=5 ("disabled index (col)")) -> (w1181:string[][])
                    }
                    frame 11 {
                      w1218 = 3  # tol
                      w1219 = 2  # res
                      w1221 = 4  # meas
                      # "fill the P/F\ncol"
                      # "fill the meas col"
                      # "check to see\npass or fail"
                      # "pull out resistor\nvalue and tolerance\nto find limits"
                      n589 = Index Array(array=w1220, index (row) #1=w1206, index (col) #1=w1219, index (row) #2=w1206, index (col) #2=w1218) -> (element #1=w1217:string, element #2=w1216:string)
                      n590 = Fract/Exp String To Number(string=w1217) -> (number=w1201:dbl)  [unwired: 3 in, 1 out]
                      n591 = Fract/Exp String To Number(string=w1216) -> (number=w1215:dbl)  [unwired: 3 in, 1 out]
                      n592 = Fract/Exp String To Number(string=w1213) -> (number=w1210:dbl)  [unwired: 3 in, 1 out]
                      n593 = Divide(x=w1215, y=100.0) -> (x/y=w1202:dbl)
                      n594 = Multiply(x=w1202, y=w1201) -> (x*y=w1200:dbl)
                      n595 = Add(x=w1201, y=w1200) -> (x+y=w1212:dbl)
                      n596 = Subtract(x=w1201, y=w1200) -> (x-y=w1211:dbl)
                      n597 = In Range and Coerce(upper limit=w1212, x=w1210, lower limit=w1211) -> (In Range?=w1209:bool)  [unwired: 1 out]
                      n598 = Select(t="P", s=w1209, f="F") -> (s? t:f=w1204:string)
                      n599 = Replace Array Subset(array=w1220, new element #1=w1213, index (row) #1=w1206, index (col) #1=w1221, new element #2=w1204, index (row) #2=w1206, index (col) #2=5 ("disabled index (col)")) -> (w1203:string[][])
                    }
                    frame 12 {
                      w1240 = 3  # tol
                      w1241 = 2  # res
                      w1243 = 4  # meas
                      # "fill the P/F\ncol"
                      # "fill the meas col"
                      # "check to see\npass or fail"
                      # "pull out resistor\nvalue and tolerance\nto find limits"
                      n600 = Index Array(array=w1242, index (row) #1=w1228, index (col) #1=w1241, index (row) #2=w1228, index (col) #2=w1240) -> (element #1=w1239:string, element #2=w1238:string)
                      n601 = Fract/Exp String To Number(string=w1239) -> (number=w1223:dbl)  [unwired: 3 in, 1 out]
                      n602 = Fract/Exp String To Number(string=w1238) -> (number=w1237:dbl)  [unwired: 3 in, 1 out]
                      n603 = Fract/Exp String To Number(string=w1235) -> (number=w1232:dbl)  [unwired: 3 in, 1 out]
                      n604 = Divide(x=w1237, y=100.0) -> (x/y=w1224:dbl)
                      n605 = Multiply(x=w1224, y=w1223) -> (x*y=w1222:dbl)
                      n606 = Add(x=w1223, y=w1222) -> (x+y=w1234:dbl)
                      n607 = Subtract(x=w1223, y=w1222) -> (x-y=w1233:dbl)
                      n608 = In Range and Coerce(upper limit=w1234, x=w1232, lower limit=w1233) -> (In Range?=w1231:bool)  [unwired: 1 out]
                      n609 = Select(t="P", s=w1231, f="F") -> (s? t:f=w1226:string)
                      n610 = Replace Array Subset(array=w1242, new element #1=w1235, index (row) #1=w1228, index (col) #1=w1243, new element #2=w1226, index (row) #2=w1228, index (col) #2=5 ("disabled index (col)")) -> (w1225:string[][])
                    }
                    frame 13 {
                      w1262 = 3  # tol
                      w1263 = 2  # res
                      w1265 = 4  # meas
                      # "fill the P/F\ncol"
                      # "fill the meas col"
                      # "check to see\npass or fail"
                      # "pull out resistor\nvalue and tolerance\nto find limits"
                      n611 = Index Array(array=w1264, index (row) #1=w1250, index (col) #1=w1263, index (row) #2=w1250, index (col) #2=w1262) -> (element #1=w1261:string, element #2=w1260:string)
                      n612 = Fract/Exp String To Number(string=w1261) -> (number=w1245:dbl)  [unwired: 3 in, 1 out]
                      n613 = Fract/Exp String To Number(string=w1260) -> (number=w1259:dbl)  [unwired: 3 in, 1 out]
                      n614 = Fract/Exp String To Number(string=w1257) -> (number=w1254:dbl)  [unwired: 3 in, 1 out]
                      n615 = Divide(x=w1259, y=100.0) -> (x/y=w1246:dbl)
                      n616 = Multiply(x=w1246, y=w1245) -> (x*y=w1244:dbl)
                      n617 = Add(x=w1245, y=w1244) -> (x+y=w1256:dbl)
                      n618 = Subtract(x=w1245, y=w1244) -> (x-y=w1255:dbl)
                      n619 = In Range and Coerce(upper limit=w1256, x=w1254, lower limit=w1255) -> (In Range?=w1253:bool)  [unwired: 1 out]
                      n620 = Select(t="P", s=w1253, f="F") -> (s? t:f=w1248:string)
                      n621 = Replace Array Subset(array=w1264, new element #1=w1257, index (row) #1=w1250, index (col) #1=w1265, new element #2=w1248, index (row) #2=w1250, index (col) #2=5 ("disabled index (col)")) -> (w1247:string[][])
                    }
                    frame 14 {
                      w1284 = 3  # tol
                      w1285 = 2  # res
                      w1287 = 4  # meas
                      # "fill the P/F\ncol"
                      # "fill the meas col"
                      # "check to see\npass or fail"
                      # "pull out resistor\nvalue and tolerance\nto find limits"
                      n622 = Index Array(array=w1286, index (row) #1=w1272, index (col) #1=w1285, index (row) #2=w1272, index (col) #2=w1284) -> (element #1=w1283:string, element #2=w1282:string)
                      n623 = Fract/Exp String To Number(string=w1283) -> (number=w1267:dbl)  [unwired: 3 in, 1 out]
                      n624 = Fract/Exp String To Number(string=w1282) -> (number=w1281:dbl)  [unwired: 3 in, 1 out]
                      n625 = Fract/Exp String To Number(string=w1279) -> (number=w1276:dbl)  [unwired: 3 in, 1 out]
                      n626 = Divide(x=w1281, y=100.0) -> (x/y=w1268:dbl)
                      n627 = Multiply(x=w1268, y=w1267) -> (x*y=w1266:dbl)
                      n628 = Add(x=w1267, y=w1266) -> (x+y=w1278:dbl)
                      n629 = Subtract(x=w1267, y=w1266) -> (x-y=w1277:dbl)
                      n630 = In Range and Coerce(upper limit=w1278, x=w1276, lower limit=w1277) -> (In Range?=w1275:bool)  [unwired: 1 out]
                      n631 = Select(t="P", s=w1275, f="F") -> (s? t:f=w1270:string)
                      n632 = Replace Array Subset(array=w1286, new element #1=w1279, index (row) #1=w1272, index (col) #1=w1287, new element #2=w1270, index (row) #2=w1272, index (col) #2=5 ("disabled index (col)")) -> (w1269:string[][])
                    }
                    frame 15 {
                      w1306 = 3  # tol
                      w1307 = 2  # res
                      w1309 = 4  # meas
                      # "fill the P/F\ncol"
                      # "fill the meas col"
                      # "check to see\npass or fail"
                      # "pull out resistor\nvalue and tolerance\nto find limits"
                      n633 = Index Array(array=w1308, index (row) #1=w1294, index (col) #1=w1307, index (row) #2=w1294, index (col) #2=w1306) -> (element #1=w1305:string, element #2=w1304:string)
                      n634 = Fract/Exp String To Number(string=w1305) -> (number=w1289:dbl)  [unwired: 3 in, 1 out]
                      n635 = Fract/Exp String To Number(string=w1304) -> (number=w1303:dbl)  [unwired: 3 in, 1 out]
                      n636 = Fract/Exp String To Number(string=w1301) -> (number=w1298:dbl)  [unwired: 3 in, 1 out]
                      n637 = Divide(x=w1303, y=100.0) -> (x/y=w1290:dbl)
                      n638 = Multiply(x=w1290, y=w1289) -> (x*y=w1288:dbl)
                      n639 = Add(x=w1289, y=w1288) -> (x+y=w1300:dbl)
                      n640 = Subtract(x=w1289, y=w1288) -> (x-y=w1299:dbl)
                      n641 = In Range and Coerce(upper limit=w1300, x=w1298, lower limit=w1299) -> (In Range?=w1297:bool)  [unwired: 1 out]
                      n642 = Select(t="P", s=w1297, f="F") -> (s? t:f=w1292:string)
                      n643 = Replace Array Subset(array=w1308, new element #1=w1301, index (row) #1=w1294, index (col) #1=w1309, new element #2=w1292, index (row) #2=w1294, index (col) #2=5 ("disabled index (col)")) -> (w1291:string[][])
                    }
                    frame 16 {
                      w1328 = 3  # tol
                      w1329 = 2  # res
                      w1331 = 4  # meas
                      # "fill the P/F\ncol"
                      # "fill the meas col"
                      # "check to see\npass or fail"
                      # "pull out resistor\nvalue and tolerance\nto find limits"
                      n644 = Index Array(array=w1330, index (row) #1=w1316, index (col) #1=w1329, index (row) #2=w1316, index (col) #2=w1328) -> (element #1=w1327:string, element #2=w1326:string)
                      n645 = Fract/Exp String To Number(string=w1327) -> (number=w1311:dbl)  [unwired: 3 in, 1 out]
                      n646 = Fract/Exp String To Number(string=w1326) -> (number=w1325:dbl)  [unwired: 3 in, 1 out]
                      n647 = Fract/Exp String To Number(string=w1323) -> (number=w1320:dbl)  [unwired: 3 in, 1 out]
                      n648 = Divide(x=w1325, y=100.0) -> (x/y=w1312:dbl)
                      n649 = Multiply(x=w1312, y=w1311) -> (x*y=w1310:dbl)
                      n650 = Add(x=w1311, y=w1310) -> (x+y=w1322:dbl)
                      n651 = Subtract(x=w1311, y=w1310) -> (x-y=w1321:dbl)
                      n652 = In Range and Coerce(upper limit=w1322, x=w1320, lower limit=w1321) -> (In Range?=w1319:bool)  [unwired: 1 out]
                      n653 = Select(t="P", s=w1319, f="F") -> (s? t:f=w1314:string)
                      n654 = Replace Array Subset(array=w1330, new element #1=w1323, index (row) #1=w1316, index (col) #1=w1331, new element #2=w1314, index (row) #2=w1316, index (col) #2=5 ("disabled index (col)")) -> (w1313:string[][])
                    }
                    frame 17 {
                      w1350 = 3  # tol
                      w1351 = 2  # res
                      w1353 = 4  # meas
                      # "fill the P/F\ncol"
                      # "fill the meas col"
                      # "check to see\npass or fail"
                      # "pull out resistor\nvalue and tolerance\nto find limits"
                      n655 = Index Array(array=w1352, index (row) #1=w1338, index (col) #1=w1351, index (row) #2=w1338, index (col) #2=w1350) -> (element #1=w1349:string, element #2=w1348:string)
                      n656 = Fract/Exp String To Number(string=w1349) -> (number=w1333:dbl)  [unwired: 3 in, 1 out]
                      n657 = Fract/Exp String To Number(string=w1348) -> (number=w1347:dbl)  [unwired: 3 in, 1 out]
                      n658 = Fract/Exp String To Number(string=w1345) -> (number=w1342:dbl)  [unwired: 3 in, 1 out]
                      n659 = Divide(x=w1347, y=100.0) -> (x/y=w1334:dbl)
                      n660 = Multiply(x=w1334, y=w1333) -> (x*y=w1332:dbl)
                      n661 = Add(x=w1333, y=w1332) -> (x+y=w1344:dbl)
                      n662 = Subtract(x=w1333, y=w1332) -> (x-y=w1343:dbl)
                      n663 = In Range and Coerce(upper limit=w1344, x=w1342, lower limit=w1343) -> (In Range?=w1341:bool)  [unwired: 1 out]
                      n664 = Select(t="P", s=w1341, f="F") -> (s? t:f=w1336:string)
                      n665 = Replace Array Subset(array=w1352, new element #1=w1345, index (row) #1=w1338, index (col) #1=w1353, new element #2=w1336, index (row) #2=w1338, index (col) #2=5 ("disabled index (col)")) -> (w1335:string[][])
                    }
                    frame 18 {
                      w1372 = 3  # tol
                      w1373 = 2  # res
                      w1375 = 4  # meas
                      # "fill the P/F\ncol"
                      # "fill the meas col"
                      # "check to see\npass or fail"
                      # "pull out resistor\nvalue and tolerance\nto find limits"
                      n666 = Index Array(array=w1374, index (row) #1=w1360, index (col) #1=w1373, index (row) #2=w1360, index (col) #2=w1372) -> (element #1=w1371:string, element #2=w1370:string)
                      n667 = Fract/Exp String To Number(string=w1371) -> (number=w1355:dbl)  [unwired: 3 in, 1 out]
                      n668 = Fract/Exp String To Number(string=w1370) -> (number=w1369:dbl)  [unwired: 3 in, 1 out]
                      n669 = Fract/Exp String To Number(string=w1367) -> (number=w1364:dbl)  [unwired: 3 in, 1 out]
                      n670 = Divide(x=w1369, y=100.0) -> (x/y=w1356:dbl)
                      n671 = Multiply(x=w1356, y=w1355) -> (x*y=w1354:dbl)
                      n672 = Add(x=w1355, y=w1354) -> (x+y=w1366:dbl)
                      n673 = Subtract(x=w1355, y=w1354) -> (x-y=w1365:dbl)
                      n674 = In Range and Coerce(upper limit=w1366, x=w1364, lower limit=w1365) -> (In Range?=w1363:bool)  [unwired: 1 out]
                      n675 = Select(t="P", s=w1363, f="F") -> (s? t:f=w1358:string)
                      n676 = Replace Array Subset(array=w1374, new element #1=w1367, index (row) #1=w1360, index (col) #1=w1375, new element #2=w1358, index (row) #2=w1360, index (col) #2=5 ("disabled index (col)")) -> (w1357:string[][])
                    }
                    frame 19 {
                      w1394 = 3  # tol
                      w1395 = 2  # res
                      w1397 = 4  # meas
                      # "fill the P/F\ncol"
                      # "fill the meas col"
                      # "check to see\npass or fail"
                      # "pull out resistor\nvalue and tolerance\nto find limits"
                      n677 = Index Array(array=w1396, index (row) #1=w1382, index (col) #1=w1395, index (row) #2=w1382, index (col) #2=w1394) -> (element #1=w1393:string, element #2=w1392:string)
                      n678 = Fract/Exp String To Number(string=w1393) -> (number=w1377:dbl)  [unwired: 3 in, 1 out]
                      n679 = Fract/Exp String To Number(string=w1392) -> (number=w1391:dbl)  [unwired: 3 in, 1 out]
                      n680 = Fract/Exp String To Number(string=w1389) -> (number=w1386:dbl)  [unwired: 3 in, 1 out]
                      n681 = Divide(x=w1391, y=100.0) -> (x/y=w1378:dbl)
                      n682 = Multiply(x=w1378, y=w1377) -> (x*y=w1376:dbl)
                      n683 = Add(x=w1377, y=w1376) -> (x+y=w1388:dbl)
                      n684 = Subtract(x=w1377, y=w1376) -> (x-y=w1387:dbl)
                      n685 = In Range and Coerce(upper limit=w1388, x=w1386, lower limit=w1387) -> (In Range?=w1385:bool)  [unwired: 1 out]
                      n686 = Select(t="P", s=w1385, f="F") -> (s? t:f=w1380:string)
                      n687 = Replace Array Subset(array=w1396, new element #1=w1389, index (row) #1=w1382, index (col) #1=w1397, new element #2=w1380, index (row) #2=w1382, index (col) #2=5 ("disabled index (col)")) -> (w1379:string[][])
                    }
                    frame 20 {
                      w1416 = 3  # tol
                      w1417 = 2  # res
                      w1419 = 4  # meas
                      # "fill the P/F\ncol"
                      # "fill the meas col"
                      # "check to see\npass or fail"
                      # "pull out resistor\nvalue and tolerance\nto find limits"
                      n688 = Index Array(array=w1418, index (row) #1=w1404, index (col) #1=w1417, index (row) #2=w1404, index (col) #2=w1416) -> (element #1=w1415:string, element #2=w1414:string)
                      n689 = Fract/Exp String To Number(string=w1415) -> (number=w1399:dbl)  [unwired: 3 in, 1 out]
                      n690 = Fract/Exp String To Number(string=w1414) -> (number=w1413:dbl)  [unwired: 3 in, 1 out]
                      n691 = Fract/Exp String To Number(string=w1411) -> (number=w1408:dbl)  [unwired: 3 in, 1 out]
                      n692 = Divide(x=w1413, y=100.0) -> (x/y=w1400:dbl)
                      n693 = Multiply(x=w1400, y=w1399) -> (x*y=w1398:dbl)
                      n694 = Add(x=w1399, y=w1398) -> (x+y=w1410:dbl)
                      n695 = Subtract(x=w1399, y=w1398) -> (x-y=w1409:dbl)
                      n696 = In Range and Coerce(upper limit=w1410, x=w1408, lower limit=w1409) -> (In Range?=w1407:bool)  [unwired: 1 out]
                      n697 = Select(t="P", s=w1407, f="F") -> (s? t:f=w1402:string)
                      n698 = Replace Array Subset(array=w1418, new element #1=w1411, index (row) #1=w1404, index (col) #1=w1419, new element #2=w1402, index (row) #2=w1404, index (col) #2=5 ("disabled index (col)")) -> (w1401:string[][])
                    }
                    frame 21 {
                      w1438 = 3  # tol
                      w1439 = 2  # res
                      w1441 = 4  # meas
                      # "fill the P/F\ncol"
                      # "fill the meas col"
                      # "check to see\npass or fail"
                      # "pull out resistor\nvalue and tolerance\nto find limits"
                      n699 = Index Array(array=w1440, index (row) #1=w1426, index (col) #1=w1439, index (row) #2=w1426, index (col) #2=w1438) -> (element #1=w1437:string, element #2=w1436:string)
                      n700 = Fract/Exp String To Number(string=w1437) -> (number=w1421:dbl)  [unwired: 3 in, 1 out]
                      n701 = Fract/Exp String To Number(string=w1436) -> (number=w1435:dbl)  [unwired: 3 in, 1 out]
                      n702 = Fract/Exp String To Number(string=w1433) -> (number=w1430:dbl)  [unwired: 3 in, 1 out]
                      n703 = Divide(x=w1435, y=100.0) -> (x/y=w1422:dbl)
                      n704 = Multiply(x=w1422, y=w1421) -> (x*y=w1420:dbl)
                      n705 = Add(x=w1421, y=w1420) -> (x+y=w1432:dbl)
                      n706 = Subtract(x=w1421, y=w1420) -> (x-y=w1431:dbl)
                      n707 = In Range and Coerce(upper limit=w1432, x=w1430, lower limit=w1431) -> (In Range?=w1429:bool)  [unwired: 1 out]
                      n708 = Select(t="P", s=w1429, f="F") -> (s? t:f=w1424:string)
                      n709 = Replace Array Subset(array=w1440, new element #1=w1433, index (row) #1=w1426, index (col) #1=w1441, new element #2=w1424, index (row) #2=w1426, index (col) #2=5 ("disabled index (col)")) -> (w1423:string[][])
                    }
                    frame 22 {
                      w1460 = 3  # tol
                      w1461 = 2  # res
                      w1463 = 4  # meas
                      # "fill the P/F\ncol"
                      # "fill the meas col"
                      # "check to see\npass or fail"
                      # "pull out resistor\nvalue and tolerance\nto find limits"
                      n710 = Index Array(array=w1462, index (row) #1=w1448, index (col) #1=w1461, index (row) #2=w1448, index (col) #2=w1460) -> (element #1=w1459:string, element #2=w1458:string)
                      n711 = Fract/Exp String To Number(string=w1459) -> (number=w1443:dbl)  [unwired: 3 in, 1 out]
                      n712 = Fract/Exp String To Number(string=w1458) -> (number=w1457:dbl)  [unwired: 3 in, 1 out]
                      n713 = Fract/Exp String To Number(string=w1455) -> (number=w1452:dbl)  [unwired: 3 in, 1 out]
                      n714 = Divide(x=w1457, y=100.0) -> (x/y=w1444:dbl)
                      n715 = Multiply(x=w1444, y=w1443) -> (x*y=w1442:dbl)
                      n716 = Add(x=w1443, y=w1442) -> (x+y=w1454:dbl)
                      n717 = Subtract(x=w1443, y=w1442) -> (x-y=w1453:dbl)
                      n718 = In Range and Coerce(upper limit=w1454, x=w1452, lower limit=w1453) -> (In Range?=w1451:bool)  [unwired: 1 out]
                      n719 = Select(t="P", s=w1451, f="F") -> (s? t:f=w1446:string)
                      n720 = Replace Array Subset(array=w1462, new element #1=w1455, index (row) #1=w1448, index (col) #1=w1463, new element #2=w1446, index (row) #2=w1448, index (col) #2=5 ("disabled index (col)")) -> (w1445:string[][])
                    }
                    frame 23 {
                      w1482 = 3  # tol
                      w1483 = 2  # res
                      w1485 = 4  # meas
                      # "fill the P/F\ncol"
                      # "fill the meas col"
                      # "check to see\npass or fail"
                      # "pull out resistor\nvalue and tolerance\nto find limits"
                      n721 = Index Array(array=w1484, index (row) #1=w1470, index (col) #1=w1483, index (row) #2=w1470, index (col) #2=w1482) -> (element #1=w1481:string, element #2=w1480:string)
                      n722 = Fract/Exp String To Number(string=w1481) -> (number=w1465:dbl)  [unwired: 3 in, 1 out]
                      n723 = Fract/Exp String To Number(string=w1480) -> (number=w1479:dbl)  [unwired: 3 in, 1 out]
                      n724 = Fract/Exp String To Number(string=w1477) -> (number=w1474:dbl)  [unwired: 3 in, 1 out]
                      n725 = Divide(x=w1479, y=100.0) -> (x/y=w1466:dbl)
                      n726 = Multiply(x=w1466, y=w1465) -> (x*y=w1464:dbl)
                      n727 = Add(x=w1465, y=w1464) -> (x+y=w1476:dbl)
                      n728 = Subtract(x=w1465, y=w1464) -> (x-y=w1475:dbl)
                      n729 = In Range and Coerce(upper limit=w1476, x=w1474, lower limit=w1475) -> (In Range?=w1473:bool)  [unwired: 1 out]
                      n730 = Select(t="P", s=w1473, f="F") -> (s? t:f=w1468:string)
                      n731 = Replace Array Subset(array=w1484, new element #1=w1477, index (row) #1=w1470, index (col) #1=w1485, new element #2=w1468, index (row) #2=w1470, index (col) #2=5 ("disabled index (col)")) -> (w1467:string[][])
                    }
                    frame 24 {
                      w1504 = 3  # tol
                      w1505 = 2  # res
                      w1507 = 4  # meas
                      # "fill the P/F\ncol"
                      # "fill the meas col"
                      # "check to see\npass or fail"
                      # "pull out resistor\nvalue and tolerance\nto find limits"
                      n732 = Index Array(array=w1506, index (row) #1=w1492, index (col) #1=w1505, index (row) #2=w1492, index (col) #2=w1504) -> (element #1=w1503:string, element #2=w1502:string)
                      n733 = Fract/Exp String To Number(string=w1503) -> (number=w1487:dbl)  [unwired: 3 in, 1 out]
                      n734 = Fract/Exp String To Number(string=w1502) -> (number=w1501:dbl)  [unwired: 3 in, 1 out]
                      n735 = Fract/Exp String To Number(string=w1499) -> (number=w1496:dbl)  [unwired: 3 in, 1 out]
                      n736 = Divide(x=w1501, y=100.0) -> (x/y=w1488:dbl)
                      n737 = Multiply(x=w1488, y=w1487) -> (x*y=w1486:dbl)
                      n738 = Add(x=w1487, y=w1486) -> (x+y=w1498:dbl)
                      n739 = Subtract(x=w1487, y=w1486) -> (x-y=w1497:dbl)
                      n740 = In Range and Coerce(upper limit=w1498, x=w1496, lower limit=w1497) -> (In Range?=w1495:bool)  [unwired: 1 out]
                      n741 = Select(t="P", s=w1495, f="F") -> (s? t:f=w1490:string)
                      n742 = Replace Array Subset(array=w1506, new element #1=w1499, index (row) #1=w1492, index (col) #1=w1507, new element #2=w1490, index (row) #2=w1492, index (col) #2=5 ("disabled index (col)")) -> (w1489:string[][])
                    }
                    frame 25 {
                      w1526 = 3  # tol
                      w1527 = 2  # res
                      w1529 = 4  # meas
                      # "fill the P/F\ncol"
                      # "fill the meas col"
                      # "check to see\npass or fail"
                      # "pull out resistor\nvalue and tolerance\nto find limits"
                      n743 = Index Array(array=w1528, index (row) #1=w1514, index (col) #1=w1527, index (row) #2=w1514, index (col) #2=w1526) -> (element #1=w1525:string, element #2=w1524:string)
                      n744 = Fract/Exp String To Number(string=w1525) -> (number=w1509:dbl)  [unwired: 3 in, 1 out]
                      n745 = Fract/Exp String To Number(string=w1524) -> (number=w1523:dbl)  [unwired: 3 in, 1 out]
                      n746 = Fract/Exp String To Number(string=w1521) -> (number=w1518:dbl)  [unwired: 3 in, 1 out]
                      n747 = Divide(x=w1523, y=100.0) -> (x/y=w1510:dbl)
                      n748 = Multiply(x=w1510, y=w1509) -> (x*y=w1508:dbl)
                      n749 = Add(x=w1509, y=w1508) -> (x+y=w1520:dbl)
                      n750 = Subtract(x=w1509, y=w1508) -> (x-y=w1519:dbl)
                      n751 = In Range and Coerce(upper limit=w1520, x=w1518, lower limit=w1519) -> (In Range?=w1517:bool)  [unwired: 1 out]
                      n752 = Select(t="P", s=w1517, f="F") -> (s? t:f=w1512:string)
                      n753 = Replace Array Subset(array=w1528, new element #1=w1521, index (row) #1=w1514, index (col) #1=w1529, new element #2=w1512, index (row) #2=w1514, index (col) #2=5 ("disabled index (col)")) -> (w1511:string[][])
                    }
                    frame 26 {
                      w1548 = 3  # tol
                      w1549 = 2  # res
                      w1551 = 4  # meas
                      # "fill the P/F\ncol"
                      # "fill the meas col"
                      # "check to see\npass or fail"
                      # "pull out resistor\nvalue and tolerance\nto find limits"
                      n754 = Index Array(array=w1550, index (row) #1=w1536, index (col) #1=w1549, index (row) #2=w1536, index (col) #2=w1548) -> (element #1=w1547:string, element #2=w1546:string)
                      n755 = Fract/Exp String To Number(string=w1547) -> (number=w1531:dbl)  [unwired: 3 in, 1 out]
                      n756 = Fract/Exp String To Number(string=w1546) -> (number=w1545:dbl)  [unwired: 3 in, 1 out]
                      n757 = Fract/Exp String To Number(string=w1543) -> (number=w1540:dbl)  [unwired: 3 in, 1 out]
                      n758 = Divide(x=w1545, y=100.0) -> (x/y=w1532:dbl)
                      n759 = Multiply(x=w1532, y=w1531) -> (x*y=w1530:dbl)
                      n760 = Add(x=w1531, y=w1530) -> (x+y=w1542:dbl)
                      n761 = Subtract(x=w1531, y=w1530) -> (x-y=w1541:dbl)
                      n762 = In Range and Coerce(upper limit=w1542, x=w1540, lower limit=w1541) -> (In Range?=w1539:bool)  [unwired: 1 out]
                      n763 = Select(t="P", s=w1539, f="F") -> (s? t:f=w1534:string)
                      n764 = Replace Array Subset(array=w1550, new element #1=w1543, index (row) #1=w1536, index (col) #1=w1551, new element #2=w1534, index (row) #2=w1536, index (col) #2=5 ("disabled index (col)")) -> (w1533:string[][])
                    }
                    frame 27 {
                      w1570 = 3  # tol
                      w1571 = 2  # res
                      w1573 = 4  # meas
                      # "fill the P/F\ncol"
                      # "fill the meas col"
                      # "check to see\npass or fail"
                      # "pull out resistor\nvalue and tolerance\nto find limits"
                      n765 = Index Array(array=w1572, index (row) #1=w1558, index (col) #1=w1571, index (row) #2=w1558, index (col) #2=w1570) -> (element #1=w1569:string, element #2=w1568:string)
                      n766 = Fract/Exp String To Number(string=w1569) -> (number=w1553:dbl)  [unwired: 3 in, 1 out]
                      n767 = Fract/Exp String To Number(string=w1568) -> (number=w1567:dbl)  [unwired: 3 in, 1 out]
                      n768 = Fract/Exp String To Number(string=w1565) -> (number=w1562:dbl)  [unwired: 3 in, 1 out]
                      n769 = Divide(x=w1567, y=100.0) -> (x/y=w1554:dbl)
                      n770 = Multiply(x=w1554, y=w1553) -> (x*y=w1552:dbl)
                      n771 = Add(x=w1553, y=w1552) -> (x+y=w1564:dbl)
                      n772 = Subtract(x=w1553, y=w1552) -> (x-y=w1563:dbl)
                      n773 = In Range and Coerce(upper limit=w1564, x=w1562, lower limit=w1563) -> (In Range?=w1561:bool)  [unwired: 1 out]
                      n774 = Select(t="P", s=w1561, f="F") -> (s? t:f=w1556:string)
                      n775 = Replace Array Subset(array=w1572, new element #1=w1565, index (row) #1=w1558, index (col) #1=w1573, new element #2=w1556, index (row) #2=w1558, index (col) #2=5 ("disabled index (col)")) -> (w1555:string[][])
                    }
                    frame 28 {
                      w1592 = 3  # tol
                      w1593 = 2  # res
                      w1595 = 4  # meas
                      # "fill the P/F\ncol"
                      # "fill the meas col"
                      # "check to see\npass or fail"
                      # "pull out resistor\nvalue and tolerance\nto find limits"
                      n776 = Index Array(array=w1594, index (row) #1=w1580, index (col) #1=w1593, index (row) #2=w1580, index (col) #2=w1592) -> (element #1=w1591:string, element #2=w1590:string)
                      n777 = Fract/Exp String To Number(string=w1591) -> (number=w1575:dbl)  [unwired: 3 in, 1 out]
                      n778 = Fract/Exp String To Number(string=w1590) -> (number=w1589:dbl)  [unwired: 3 in, 1 out]
                      n779 = Fract/Exp String To Number(string=w1587) -> (number=w1584:dbl)  [unwired: 3 in, 1 out]
                      n780 = Divide(x=w1589, y=100.0) -> (x/y=w1576:dbl)
                      n781 = Multiply(x=w1576, y=w1575) -> (x*y=w1574:dbl)
                      n782 = Add(x=w1575, y=w1574) -> (x+y=w1586:dbl)
                      n783 = Subtract(x=w1575, y=w1574) -> (x-y=w1585:dbl)
                      n784 = In Range and Coerce(upper limit=w1586, x=w1584, lower limit=w1585) -> (In Range?=w1583:bool)  [unwired: 1 out]
                      n785 = Select(t="P", s=w1583, f="F") -> (s? t:f=w1578:string)
                      n786 = Replace Array Subset(array=w1594, new element #1=w1587, index (row) #1=w1580, index (col) #1=w1595, new element #2=w1578, index (row) #2=w1580, index (col) #2=5 ("disabled index (col)")) -> (w1577:string[][])
                    }
                    frame 29 {
                      w1614 = 3  # tol
                      w1615 = 2  # res
                      w1617 = 4  # meas
                      # "fill the P/F\ncol"
                      # "fill the meas col"
                      # "check to see\npass or fail"
                      # "pull out resistor\nvalue and tolerance\nto find limits"
                      n787 = Index Array(array=w1616, index (row) #1=w1602, index (col) #1=w1615, index (row) #2=w1602, index (col) #2=w1614) -> (element #1=w1613:string, element #2=w1612:string)
                      n788 = Fract/Exp String To Number(string=w1613) -> (number=w1597:dbl)  [unwired: 3 in, 1 out]
                      n789 = Fract/Exp String To Number(string=w1612) -> (number=w1611:dbl)  [unwired: 3 in, 1 out]
                      n790 = Fract/Exp String To Number(string=w1609) -> (number=w1606:dbl)  [unwired: 3 in, 1 out]
                      n791 = Divide(x=w1611, y=100.0) -> (x/y=w1598:dbl)
                      n792 = Multiply(x=w1598, y=w1597) -> (x*y=w1596:dbl)
                      n793 = Add(x=w1597, y=w1596) -> (x+y=w1608:dbl)
                      n794 = Subtract(x=w1597, y=w1596) -> (x-y=w1607:dbl)
                      n795 = In Range and Coerce(upper limit=w1608, x=w1606, lower limit=w1607) -> (In Range?=w1605:bool)  [unwired: 1 out]
                      n796 = Select(t="P", s=w1605, f="F") -> (s? t:f=w1600:string)
                      n797 = Replace Array Subset(array=w1616, new element #1=w1609, index (row) #1=w1602, index (col) #1=w1617, new element #2=w1600, index (row) #2=w1602, index (col) #2=5 ("disabled index (col)")) -> (w1599:string[][])
                    }
                    frame 30 {
                      w1636 = 3  # tol
                      w1637 = 2  # res
                      w1639 = 4  # meas
                      # "fill the P/F\ncol"
                      # "fill the meas col"
                      # "check to see\npass or fail"
                      # "pull out resistor\nvalue and tolerance\nto find limits"
                      n798 = Index Array(array=w1638, index (row) #1=w1624, index (col) #1=w1637, index (row) #2=w1624, index (col) #2=w1636) -> (element #1=w1635:string, element #2=w1634:string)
                      n799 = Fract/Exp String To Number(string=w1635) -> (number=w1619:dbl)  [unwired: 3 in, 1 out]
                      n800 = Fract/Exp String To Number(string=w1634) -> (number=w1633:dbl)  [unwired: 3 in, 1 out]
                      n801 = Fract/Exp String To Number(string=w1631) -> (number=w1628:dbl)  [unwired: 3 in, 1 out]
                      n802 = Divide(x=w1633, y=100.0) -> (x/y=w1620:dbl)
                      n803 = Multiply(x=w1620, y=w1619) -> (x*y=w1618:dbl)
                      n804 = Add(x=w1619, y=w1618) -> (x+y=w1630:dbl)
                      n805 = Subtract(x=w1619, y=w1618) -> (x-y=w1629:dbl)
                      n806 = In Range and Coerce(upper limit=w1630, x=w1628, lower limit=w1629) -> (In Range?=w1627:bool)  [unwired: 1 out]
                      n807 = Select(t="P", s=w1627, f="F") -> (s? t:f=w1622:string)
                      n808 = Replace Array Subset(array=w1638, new element #1=w1631, index (row) #1=w1624, index (col) #1=w1639, new element #2=w1622, index (row) #2=w1624, index (col) #2=5 ("disabled index (col)")) -> (w1621:string[][])
                    }
                    frame 31 {
                      w1658 = 3  # tol
                      w1659 = 2  # res
                      w1661 = 4  # meas
                      # "fill the P/F\ncol"
                      # "fill the meas col"
                      # "check to see\npass or fail"
                      # "pull out resistor\nvalue and tolerance\nto find limits"
                      n809 = Index Array(array=w1660, index (row) #1=w1646, index (col) #1=w1659, index (row) #2=w1646, index (col) #2=w1658) -> (element #1=w1657:string, element #2=w1656:string)
                      n810 = Fract/Exp String To Number(string=w1657) -> (number=w1641:dbl)  [unwired: 3 in, 1 out]
                      n811 = Fract/Exp String To Number(string=w1656) -> (number=w1655:dbl)  [unwired: 3 in, 1 out]
                      n812 = Fract/Exp String To Number(string=w1653) -> (number=w1650:dbl)  [unwired: 3 in, 1 out]
                      n813 = Divide(x=w1655, y=100.0) -> (x/y=w1642:dbl)
                      n814 = Multiply(x=w1642, y=w1641) -> (x*y=w1640:dbl)
                      n815 = Add(x=w1641, y=w1640) -> (x+y=w1652:dbl)
                      n816 = Subtract(x=w1641, y=w1640) -> (x-y=w1651:dbl)
                      n817 = In Range and Coerce(upper limit=w1652, x=w1650, lower limit=w1651) -> (In Range?=w1649:bool)  [unwired: 1 out]
                      n818 = Select(t="P", s=w1649, f="F") -> (s? t:f=w1644:string)
                      n819 = Replace Array Subset(array=w1660, new element #1=w1653, index (row) #1=w1646, index (col) #1=w1661, new element #2=w1644, index (row) #2=w1646, index (col) #2=5 ("disabled index (col)")) -> (w1643:string[][])
                    }
                    frame 32 {
                      w1680 = 3  # tol
                      w1681 = 2  # res
                      w1683 = 4  # meas
                      # "fill the P/F\ncol"
                      # "fill the meas col"
                      # "check to see\npass or fail"
                      # "pull out resistor\nvalue and tolerance\nto find limits"
                      n820 = Index Array(array=w1682, index (row) #1=w1668, index (col) #1=w1681, index (row) #2=w1668, index (col) #2=w1680) -> (element #1=w1679:string, element #2=w1678:string)
                      n821 = Fract/Exp String To Number(string=w1679) -> (number=w1663:dbl)  [unwired: 3 in, 1 out]
                      n822 = Fract/Exp String To Number(string=w1678) -> (number=w1677:dbl)  [unwired: 3 in, 1 out]
                      n823 = Fract/Exp String To Number(string=w1675) -> (number=w1672:dbl)  [unwired: 3 in, 1 out]
                      n824 = Divide(x=w1677, y=100.0) -> (x/y=w1664:dbl)
                      n825 = Multiply(x=w1664, y=w1663) -> (x*y=w1662:dbl)
                      n826 = Add(x=w1663, y=w1662) -> (x+y=w1674:dbl)
                      n827 = Subtract(x=w1663, y=w1662) -> (x-y=w1673:dbl)
                      n828 = In Range and Coerce(upper limit=w1674, x=w1672, lower limit=w1673) -> (In Range?=w1671:bool)  [unwired: 1 out]
                      n829 = Select(t="P", s=w1671, f="F") -> (s? t:f=w1666:string)
                      n830 = Replace Array Subset(array=w1682, new element #1=w1675, index (row) #1=w1668, index (col) #1=w1683, new element #2=w1666, index (row) #2=w1668, index (col) #2=5 ("disabled index (col)")) -> (w1665:string[][])
                    }
                    frame 33 {
                      w1702 = 3  # tol
                      w1703 = 2  # res
                      w1705 = 4  # meas
                      # "fill the P/F\ncol"
                      # "fill the meas col"
                      # "check to see\npass or fail"
                      # "pull out resistor\nvalue and tolerance\nto find limits"
                      n831 = Index Array(array=w1704, index (row) #1=w1690, index (col) #1=w1703, index (row) #2=w1690, index (col) #2=w1702) -> (element #1=w1701:string, element #2=w1700:string)
                      n832 = Fract/Exp String To Number(string=w1701) -> (number=w1685:dbl)  [unwired: 3 in, 1 out]
                      n833 = Fract/Exp String To Number(string=w1700) -> (number=w1699:dbl)  [unwired: 3 in, 1 out]
                      n834 = Fract/Exp String To Number(string=w1697) -> (number=w1694:dbl)  [unwired: 3 in, 1 out]
                      n835 = Divide(x=w1699, y=100.0) -> (x/y=w1686:dbl)
                      n836 = Multiply(x=w1686, y=w1685) -> (x*y=w1684:dbl)
                      n837 = Add(x=w1685, y=w1684) -> (x+y=w1696:dbl)
                      n838 = Subtract(x=w1685, y=w1684) -> (x-y=w1695:dbl)
                      n839 = In Range and Coerce(upper limit=w1696, x=w1694, lower limit=w1695) -> (In Range?=w1693:bool)  [unwired: 1 out]
                      n840 = Select(t="P", s=w1693, f="F") -> (s? t:f=w1688:string)
                      n841 = Replace Array Subset(array=w1704, new element #1=w1697, index (row) #1=w1690, index (col) #1=w1705, new element #2=w1688, index (row) #2=w1690, index (col) #2=5 ("disabled index (col)")) -> (w1687:string[][])
                    }
                    frame 34 {
                      w1724 = 3  # tol
                      w1725 = 2  # res
                      w1727 = 4  # meas
                      # "fill the P/F\ncol"
                      # "fill the meas col"
                      # "check to see\npass or fail"
                      # "pull out resistor\nvalue and tolerance\nto find limits"
                      n842 = Index Array(array=w1726, index (row) #1=w1712, index (col) #1=w1725, index (row) #2=w1712, index (col) #2=w1724) -> (element #1=w1723:string, element #2=w1722:string)
                      n843 = Fract/Exp String To Number(string=w1723) -> (number=w1707:dbl)  [unwired: 3 in, 1 out]
                      n844 = Fract/Exp String To Number(string=w1722) -> (number=w1721:dbl)  [unwired: 3 in, 1 out]
                      n845 = Fract/Exp String To Number(string=w1719) -> (number=w1716:dbl)  [unwired: 3 in, 1 out]
                      n846 = Divide(x=w1721, y=100.0) -> (x/y=w1708:dbl)
                      n847 = Multiply(x=w1708, y=w1707) -> (x*y=w1706:dbl)
                      n848 = Add(x=w1707, y=w1706) -> (x+y=w1718:dbl)
                      n849 = Subtract(x=w1707, y=w1706) -> (x-y=w1717:dbl)
                      n850 = In Range and Coerce(upper limit=w1718, x=w1716, lower limit=w1717) -> (In Range?=w1715:bool)  [unwired: 1 out]
                      n851 = Select(t="P", s=w1715, f="F") -> (s? t:f=w1710:string)
                      n852 = Replace Array Subset(array=w1726, new element #1=w1719, index (row) #1=w1712, index (col) #1=w1727, new element #2=w1710, index (row) #2=w1712, index (col) #2=5 ("disabled index (col)")) -> (w1709:string[][])
                    }
                  }
                }
              }
              frame "1 kOhm" {
                n853 = for {
                  tunnel: w1728 -> [w1737] mode=indexing
                  tunnel: w1730 -> [w1735]
                  shift-right: [w1733] -> w1729
                  shift-left: w1731 -> [w1736]
                  i -> [w1732]
                  # "34924A has a \nmax of 35 \nchannels."
                  n854 = Index Array(array=w1735, index=w1732) -> (element=w1734:string)
                  n855 = case shown="0, Default" w1737 {
                    selector: w1737 -> [w1744 w1766 w1788 w1810 w1832 w1854 w1876 w1898 w1920 w1942 w1964 w1986 w2008 w2030 w2052 w2074 w2096 w2118 w2140 w2162 w2184 w2206 w2228 w2250 w2272 w2294 w2316 w2338 w2360 w2382 w2404 w2426 w2448 w2470 w2492]
                    tunnel: w1736 -> [w1758 w1780 w1802 w1824 w1846 w1868 w1890 w1912 w1934 w1956 w1978 w2000 w2022 w2044 w2066 w2088 w2110 w2132 w2154 w2176 w2198 w2220 w2242 w2264 w2286 w2308 w2330 w2352 w2374 w2396 w2418 w2440 w2462 w2484 w2506]
                    tunnel: w1734 -> [w1751 w1773 w1795 w1817 w1839 w1861 w1883 w1905 w1927 w1949 w1971 w1993 w2015 w2037 w2059 w2081 w2103 w2125 w2147 w2169 w2191 w2213 w2235 w2257 w2279 w2301 w2323 w2345 w2367 w2389 w2411 w2433 w2455 w2477 w2499]
                    tunnel: [w1741 w1763 w1785 w1807 w1829 w1851 w1873 w1895 w1917 w1939 w1961 w1983 w2005 w2027 w2049 w2071 w2093 w2115 w2137 w2159 w2181 w2203 w2225 w2247 w2269 w2291 w2313 w2335 w2357 w2379 w2401 w2423 w2445 w2467 w2489] -> w1733
                    frame 0, Default {
                      w1756 = 3  # tol
                      w1757 = 2  # res
                      w1759 = 4  # meas
                      # "fill the P/F\ncol"
                      # "fill the meas col"
                      # "check to see\npass or fail"
                      # "pull out resistor\nvalue and tolerance\nto find limits"
                      n856 = Index Array(array=w1758, index (row) #1=w1744, index (col) #1=w1757, index (row) #2=w1744, index (col) #2=w1756) -> (element #1=w1755:string, element #2=w1754:string)
                      n857 = Fract/Exp String To Number(string=w1755) -> (number=w1739:dbl)  [unwired: 3 in, 1 out]
                      n858 = Fract/Exp String To Number(string=w1754) -> (number=w1753:dbl)  [unwired: 3 in, 1 out]
                      n859 = Fract/Exp String To Number(string=w1751) -> (number=w1748:dbl)  [unwired: 3 in, 1 out]
                      n860 = Divide(x=w1753, y=100.0) -> (x/y=w1740:dbl)
                      n861 = Multiply(x=w1740, y=w1739) -> (x*y=w1738:dbl)
                      n862 = Add(x=w1739, y=w1738) -> (x+y=w1750:dbl)
                      n863 = Subtract(x=w1739, y=w1738) -> (x-y=w1749:dbl)
                      n864 = In Range and Coerce(upper limit=w1750, x=w1748, lower limit=w1749) -> (In Range?=w1747:bool)  [unwired: 1 out]
                      n865 = Select(t="P", s=w1747, f="F") -> (s? t:f=w1742:string)
                      n866 = Replace Array Subset(array=w1758, new element #1=w1751, index (row) #1=w1744, index (col) #1=w1759, new element #2=w1742, index (row) #2=w1744, index (col) #2=5 ("disabled index (col)")) -> (w1741:string[][])
                    }
                    frame 1 {
                      w1778 = 3  # tol
                      w1779 = 2  # res
                      w1781 = 4  # meas
                      # "fill the P/F\ncol"
                      # "fill the meas col"
                      # "check to see\npass or fail"
                      # "pull out resistor\nvalue and tolerance\nto find limits"
                      n867 = Index Array(array=w1780, index (row) #1=w1766, index (col) #1=w1779, index (row) #2=w1766, index (col) #2=w1778) -> (element #1=w1777:string, element #2=w1776:string)
                      n868 = Fract/Exp String To Number(string=w1777) -> (number=w1761:dbl)  [unwired: 3 in, 1 out]
                      n869 = Fract/Exp String To Number(string=w1776) -> (number=w1775:dbl)  [unwired: 3 in, 1 out]
                      n870 = Fract/Exp String To Number(string=w1773) -> (number=w1770:dbl)  [unwired: 3 in, 1 out]
                      n871 = Divide(x=w1775, y=100.0) -> (x/y=w1762:dbl)
                      n872 = Multiply(x=w1762, y=w1761) -> (x*y=w1760:dbl)
                      n873 = Add(x=w1761, y=w1760) -> (x+y=w1772:dbl)
                      n874 = Subtract(x=w1761, y=w1760) -> (x-y=w1771:dbl)
                      n875 = In Range and Coerce(upper limit=w1772, x=w1770, lower limit=w1771) -> (In Range?=w1769:bool)  [unwired: 1 out]
                      n876 = Select(t="P", s=w1769, f="F") -> (s? t:f=w1764:string)
                      n877 = Replace Array Subset(array=w1780, new element #1=w1773, index (row) #1=w1766, index (col) #1=w1781, new element #2=w1764, index (row) #2=w1766, index (col) #2=5 ("disabled index (col)")) -> (w1763:string[][])
                    }
                    frame 2 {
                      w1800 = 3  # tol
                      w1801 = 2  # res
                      w1803 = 4  # meas
                      # "fill the P/F\ncol"
                      # "fill the meas col"
                      # "check to see\npass or fail"
                      # "pull out resistor\nvalue and tolerance\nto find limits"
                      n878 = Index Array(array=w1802, index (row) #1=w1788, index (col) #1=w1801, index (row) #2=w1788, index (col) #2=w1800) -> (element #1=w1799:string, element #2=w1798:string)
                      n879 = Fract/Exp String To Number(string=w1799) -> (number=w1783:dbl)  [unwired: 3 in, 1 out]
                      n880 = Fract/Exp String To Number(string=w1798) -> (number=w1797:dbl)  [unwired: 3 in, 1 out]
                      n881 = Fract/Exp String To Number(string=w1795) -> (number=w1792:dbl)  [unwired: 3 in, 1 out]
                      n882 = Divide(x=w1797, y=100.0) -> (x/y=w1784:dbl)
                      n883 = Multiply(x=w1784, y=w1783) -> (x*y=w1782:dbl)
                      n884 = Add(x=w1783, y=w1782) -> (x+y=w1794:dbl)
                      n885 = Subtract(x=w1783, y=w1782) -> (x-y=w1793:dbl)
                      n886 = In Range and Coerce(upper limit=w1794, x=w1792, lower limit=w1793) -> (In Range?=w1791:bool)  [unwired: 1 out]
                      n887 = Select(t="P", s=w1791, f="F") -> (s? t:f=w1786:string)
                      n888 = Replace Array Subset(array=w1802, new element #1=w1795, index (row) #1=w1788, index (col) #1=w1803, new element #2=w1786, index (row) #2=w1788, index (col) #2=5 ("disabled index (col)")) -> (w1785:string[][])
                    }
                    frame 3 {
                      w1822 = 3  # tol
                      w1823 = 2  # res
                      w1825 = 4  # meas
                      # "fill the P/F\ncol"
                      # "fill the meas col"
                      # "check to see\npass or fail"
                      # "pull out resistor\nvalue and tolerance\nto find limits"
                      n889 = Index Array(array=w1824, index (row) #1=w1810, index (col) #1=w1823, index (row) #2=w1810, index (col) #2=w1822) -> (element #1=w1821:string, element #2=w1820:string)
                      n890 = Fract/Exp String To Number(string=w1821) -> (number=w1805:dbl)  [unwired: 3 in, 1 out]
                      n891 = Fract/Exp String To Number(string=w1820) -> (number=w1819:dbl)  [unwired: 3 in, 1 out]
                      n892 = Fract/Exp String To Number(string=w1817) -> (number=w1814:dbl)  [unwired: 3 in, 1 out]
                      n893 = Divide(x=w1819, y=100.0) -> (x/y=w1806:dbl)
                      n894 = Multiply(x=w1806, y=w1805) -> (x*y=w1804:dbl)
                      n895 = Add(x=w1805, y=w1804) -> (x+y=w1816:dbl)
                      n896 = Subtract(x=w1805, y=w1804) -> (x-y=w1815:dbl)
                      n897 = In Range and Coerce(upper limit=w1816, x=w1814, lower limit=w1815) -> (In Range?=w1813:bool)  [unwired: 1 out]
                      n898 = Select(t="P", s=w1813, f="F") -> (s? t:f=w1808:string)
                      n899 = Replace Array Subset(array=w1824, new element #1=w1817, index (row) #1=w1810, index (col) #1=w1825, new element #2=w1808, index (row) #2=w1810, index (col) #2=5 ("disabled index (col)")) -> (w1807:string[][])
                    }
                    frame 4 {
                      w1844 = 3  # tol
                      w1845 = 2  # res
                      w1847 = 4  # meas
                      # "fill the P/F\ncol"
                      # "fill the meas col"
                      # "check to see\npass or fail"
                      # "pull out resistor\nvalue and tolerance\nto find limits"
                      n900 = Index Array(array=w1846, index (row) #1=w1832, index (col) #1=w1845, index (row) #2=w1832, index (col) #2=w1844) -> (element #1=w1843:string, element #2=w1842:string)
                      n901 = Fract/Exp String To Number(string=w1843) -> (number=w1827:dbl)  [unwired: 3 in, 1 out]
                      n902 = Fract/Exp String To Number(string=w1842) -> (number=w1841:dbl)  [unwired: 3 in, 1 out]
                      n903 = Fract/Exp String To Number(string=w1839) -> (number=w1836:dbl)  [unwired: 3 in, 1 out]
                      n904 = Divide(x=w1841, y=100.0) -> (x/y=w1828:dbl)
                      n905 = Multiply(x=w1828, y=w1827) -> (x*y=w1826:dbl)
                      n906 = Add(x=w1827, y=w1826) -> (x+y=w1838:dbl)
                      n907 = Subtract(x=w1827, y=w1826) -> (x-y=w1837:dbl)
                      n908 = In Range and Coerce(upper limit=w1838, x=w1836, lower limit=w1837) -> (In Range?=w1835:bool)  [unwired: 1 out]
                      n909 = Select(t="P", s=w1835, f="F") -> (s? t:f=w1830:string)
                      n910 = Replace Array Subset(array=w1846, new element #1=w1839, index (row) #1=w1832, index (col) #1=w1847, new element #2=w1830, index (row) #2=w1832, index (col) #2=5 ("disabled index (col)")) -> (w1829:string[][])
                    }
                    frame 5 {
                      w1866 = 3  # tol
                      w1867 = 2  # res
                      w1869 = 4  # meas
                      # "fill the P/F\ncol"
                      # "fill the meas col"
                      # "check to see\npass or fail"
                      # "pull out resistor\nvalue and tolerance\nto find limits"
                      n911 = Index Array(array=w1868, index (row) #1=w1854, index (col) #1=w1867, index (row) #2=w1854, index (col) #2=w1866) -> (element #1=w1865:string, element #2=w1864:string)
                      n912 = Fract/Exp String To Number(string=w1865) -> (number=w1849:dbl)  [unwired: 3 in, 1 out]
                      n913 = Fract/Exp String To Number(string=w1864) -> (number=w1863:dbl)  [unwired: 3 in, 1 out]
                      n914 = Fract/Exp String To Number(string=w1861) -> (number=w1858:dbl)  [unwired: 3 in, 1 out]
                      n915 = Divide(x=w1863, y=100.0) -> (x/y=w1850:dbl)
                      n916 = Multiply(x=w1850, y=w1849) -> (x*y=w1848:dbl)
                      n917 = Add(x=w1849, y=w1848) -> (x+y=w1860:dbl)
                      n918 = Subtract(x=w1849, y=w1848) -> (x-y=w1859:dbl)
                      n919 = In Range and Coerce(upper limit=w1860, x=w1858, lower limit=w1859) -> (In Range?=w1857:bool)  [unwired: 1 out]
                      n920 = Select(t="P", s=w1857, f="F") -> (s? t:f=w1852:string)
                      n921 = Replace Array Subset(array=w1868, new element #1=w1861, index (row) #1=w1854, index (col) #1=w1869, new element #2=w1852, index (row) #2=w1854, index (col) #2=5 ("disabled index (col)")) -> (w1851:string[][])
                    }
                    frame 6 {
                      w1888 = 3  # tol
                      w1889 = 2  # res
                      w1891 = 4  # meas
                      # "fill the P/F\ncol"
                      # "fill the meas col"
                      # "check to see\npass or fail"
                      # "pull out resistor\nvalue and tolerance\nto find limits"
                      n922 = Index Array(array=w1890, index (row) #1=w1876, index (col) #1=w1889, index (row) #2=w1876, index (col) #2=w1888) -> (element #1=w1887:string, element #2=w1886:string)
                      n923 = Fract/Exp String To Number(string=w1887) -> (number=w1871:dbl)  [unwired: 3 in, 1 out]
                      n924 = Fract/Exp String To Number(string=w1886) -> (number=w1885:dbl)  [unwired: 3 in, 1 out]
                      n925 = Fract/Exp String To Number(string=w1883) -> (number=w1880:dbl)  [unwired: 3 in, 1 out]
                      n926 = Divide(x=w1885, y=100.0) -> (x/y=w1872:dbl)
                      n927 = Multiply(x=w1872, y=w1871) -> (x*y=w1870:dbl)
                      n928 = Add(x=w1871, y=w1870) -> (x+y=w1882:dbl)
                      n929 = Subtract(x=w1871, y=w1870) -> (x-y=w1881:dbl)
                      n930 = In Range and Coerce(upper limit=w1882, x=w1880, lower limit=w1881) -> (In Range?=w1879:bool)  [unwired: 1 out]
                      n931 = Select(t="P", s=w1879, f="F") -> (s? t:f=w1874:string)
                      n932 = Replace Array Subset(array=w1890, new element #1=w1883, index (row) #1=w1876, index (col) #1=w1891, new element #2=w1874, index (row) #2=w1876, index (col) #2=5 ("disabled index (col)")) -> (w1873:string[][])
                    }
                    frame 7 {
                      w1910 = 3  # tol
                      w1911 = 2  # res
                      w1913 = 4  # meas
                      # "fill the P/F\ncol"
                      # "fill the meas col"
                      # "check to see\npass or fail"
                      # "pull out resistor\nvalue and tolerance\nto find limits"
                      n933 = Index Array(array=w1912, index (row) #1=w1898, index (col) #1=w1911, index (row) #2=w1898, index (col) #2=w1910) -> (element #1=w1909:string, element #2=w1908:string)
                      n934 = Fract/Exp String To Number(string=w1909) -> (number=w1893:dbl)  [unwired: 3 in, 1 out]
                      n935 = Fract/Exp String To Number(string=w1908) -> (number=w1907:dbl)  [unwired: 3 in, 1 out]
                      n936 = Fract/Exp String To Number(string=w1905) -> (number=w1902:dbl)  [unwired: 3 in, 1 out]
                      n937 = Divide(x=w1907, y=100.0) -> (x/y=w1894:dbl)
                      n938 = Multiply(x=w1894, y=w1893) -> (x*y=w1892:dbl)
                      n939 = Add(x=w1893, y=w1892) -> (x+y=w1904:dbl)
                      n940 = Subtract(x=w1893, y=w1892) -> (x-y=w1903:dbl)
                      n941 = In Range and Coerce(upper limit=w1904, x=w1902, lower limit=w1903) -> (In Range?=w1901:bool)  [unwired: 1 out]
                      n942 = Select(t="P", s=w1901, f="F") -> (s? t:f=w1896:string)
                      n943 = Replace Array Subset(array=w1912, new element #1=w1905, index (row) #1=w1898, index (col) #1=w1913, new element #2=w1896, index (row) #2=w1898, index (col) #2=5 ("disabled index (col)")) -> (w1895:string[][])
                    }
                    frame 8 {
                      w1932 = 3  # tol
                      w1933 = 2  # res
                      w1935 = 4  # meas
                      # "fill the P/F\ncol"
                      # "fill the meas col"
                      # "check to see\npass or fail"
                      # "pull out resistor\nvalue and tolerance\nto find limits"
                      n944 = Index Array(array=w1934, index (row) #1=w1920, index (col) #1=w1933, index (row) #2=w1920, index (col) #2=w1932) -> (element #1=w1931:string, element #2=w1930:string)
                      n945 = Fract/Exp String To Number(string=w1931) -> (number=w1915:dbl)  [unwired: 3 in, 1 out]
                      n946 = Fract/Exp String To Number(string=w1930) -> (number=w1929:dbl)  [unwired: 3 in, 1 out]
                      n947 = Fract/Exp String To Number(string=w1927) -> (number=w1924:dbl)  [unwired: 3 in, 1 out]
                      n948 = Divide(x=w1929, y=100.0) -> (x/y=w1916:dbl)
                      n949 = Multiply(x=w1916, y=w1915) -> (x*y=w1914:dbl)
                      n950 = Add(x=w1915, y=w1914) -> (x+y=w1926:dbl)
                      n951 = Subtract(x=w1915, y=w1914) -> (x-y=w1925:dbl)
                      n952 = In Range and Coerce(upper limit=w1926, x=w1924, lower limit=w1925) -> (In Range?=w1923:bool)  [unwired: 1 out]
                      n953 = Select(t="P", s=w1923, f="F") -> (s? t:f=w1918:string)
                      n954 = Replace Array Subset(array=w1934, new element #1=w1927, index (row) #1=w1920, index (col) #1=w1935, new element #2=w1918, index (row) #2=w1920, index (col) #2=5 ("disabled index (col)")) -> (w1917:string[][])
                    }
                    frame 9 {
                      w1954 = 3  # tol
                      w1955 = 2  # res
                      w1957 = 4  # meas
                      # "fill the P/F\ncol"
                      # "fill the meas col"
                      # "check to see\npass or fail"
                      # "pull out resistor\nvalue and tolerance\nto find limits"
                      n955 = Index Array(array=w1956, index (row) #1=w1942, index (col) #1=w1955, index (row) #2=w1942, index (col) #2=w1954) -> (element #1=w1953:string, element #2=w1952:string)
                      n956 = Fract/Exp String To Number(string=w1953) -> (number=w1937:dbl)  [unwired: 3 in, 1 out]
                      n957 = Fract/Exp String To Number(string=w1952) -> (number=w1951:dbl)  [unwired: 3 in, 1 out]
                      n958 = Fract/Exp String To Number(string=w1949) -> (number=w1946:dbl)  [unwired: 3 in, 1 out]
                      n959 = Divide(x=w1951, y=100.0) -> (x/y=w1938:dbl)
                      n960 = Multiply(x=w1938, y=w1937) -> (x*y=w1936:dbl)
                      n961 = Add(x=w1937, y=w1936) -> (x+y=w1948:dbl)
                      n962 = Subtract(x=w1937, y=w1936) -> (x-y=w1947:dbl)
                      n963 = In Range and Coerce(upper limit=w1948, x=w1946, lower limit=w1947) -> (In Range?=w1945:bool)  [unwired: 1 out]
                      n964 = Select(t="P", s=w1945, f="F") -> (s? t:f=w1940:string)
                      n965 = Replace Array Subset(array=w1956, new element #1=w1949, index (row) #1=w1942, index (col) #1=w1957, new element #2=w1940, index (row) #2=w1942, index (col) #2=5 ("disabled index (col)")) -> (w1939:string[][])
                    }
                    frame 10 {
                      w1976 = 3  # tol
                      w1977 = 2  # res
                      w1979 = 4  # meas
                      # "fill the P/F\ncol"
                      # "fill the meas col"
                      # "check to see\npass or fail"
                      # "pull out resistor\nvalue and tolerance\nto find limits"
                      n966 = Index Array(array=w1978, index (row) #1=w1964, index (col) #1=w1977, index (row) #2=w1964, index (col) #2=w1976) -> (element #1=w1975:string, element #2=w1974:string)
                      n967 = Fract/Exp String To Number(string=w1975) -> (number=w1959:dbl)  [unwired: 3 in, 1 out]
                      n968 = Fract/Exp String To Number(string=w1974) -> (number=w1973:dbl)  [unwired: 3 in, 1 out]
                      n969 = Fract/Exp String To Number(string=w1971) -> (number=w1968:dbl)  [unwired: 3 in, 1 out]
                      n970 = Divide(x=w1973, y=100.0) -> (x/y=w1960:dbl)
                      n971 = Multiply(x=w1960, y=w1959) -> (x*y=w1958:dbl)
                      n972 = Add(x=w1959, y=w1958) -> (x+y=w1970:dbl)
                      n973 = Subtract(x=w1959, y=w1958) -> (x-y=w1969:dbl)
                      n974 = In Range and Coerce(upper limit=w1970, x=w1968, lower limit=w1969) -> (In Range?=w1967:bool)  [unwired: 1 out]
                      n975 = Select(t="P", s=w1967, f="F") -> (s? t:f=w1962:string)
                      n976 = Replace Array Subset(array=w1978, new element #1=w1971, index (row) #1=w1964, index (col) #1=w1979, new element #2=w1962, index (row) #2=w1964, index (col) #2=5 ("disabled index (col)")) -> (w1961:string[][])
                    }
                    frame 11 {
                      w1998 = 3  # tol
                      w1999 = 2  # res
                      w2001 = 4  # meas
                      # "fill the P/F\ncol"
                      # "fill the meas col"
                      # "check to see\npass or fail"
                      # "pull out resistor\nvalue and tolerance\nto find limits"
                      n977 = Index Array(array=w2000, index (row) #1=w1986, index (col) #1=w1999, index (row) #2=w1986, index (col) #2=w1998) -> (element #1=w1997:string, element #2=w1996:string)
                      n978 = Fract/Exp String To Number(string=w1997) -> (number=w1981:dbl)  [unwired: 3 in, 1 out]
                      n979 = Fract/Exp String To Number(string=w1996) -> (number=w1995:dbl)  [unwired: 3 in, 1 out]
                      n980 = Fract/Exp String To Number(string=w1993) -> (number=w1990:dbl)  [unwired: 3 in, 1 out]
                      n981 = Divide(x=w1995, y=100.0) -> (x/y=w1982:dbl)
                      n982 = Multiply(x=w1982, y=w1981) -> (x*y=w1980:dbl)
                      n983 = Add(x=w1981, y=w1980) -> (x+y=w1992:dbl)
                      n984 = Subtract(x=w1981, y=w1980) -> (x-y=w1991:dbl)
                      n985 = In Range and Coerce(upper limit=w1992, x=w1990, lower limit=w1991) -> (In Range?=w1989:bool)  [unwired: 1 out]
                      n986 = Select(t="P", s=w1989, f="F") -> (s? t:f=w1984:string)
                      n987 = Replace Array Subset(array=w2000, new element #1=w1993, index (row) #1=w1986, index (col) #1=w2001, new element #2=w1984, index (row) #2=w1986, index (col) #2=5 ("disabled index (col)")) -> (w1983:string[][])
                    }
                    frame 12 {
                      w2020 = 3  # tol
                      w2021 = 2  # res
                      w2023 = 4  # meas
                      # "fill the P/F\ncol"
                      # "fill the meas col"
                      # "check to see\npass or fail"
                      # "pull out resistor\nvalue and tolerance\nto find limits"
                      n988 = Index Array(array=w2022, index (row) #1=w2008, index (col) #1=w2021, index (row) #2=w2008, index (col) #2=w2020) -> (element #1=w2019:string, element #2=w2018:string)
                      n989 = Fract/Exp String To Number(string=w2019) -> (number=w2003:dbl)  [unwired: 3 in, 1 out]
                      n990 = Fract/Exp String To Number(string=w2018) -> (number=w2017:dbl)  [unwired: 3 in, 1 out]
                      n991 = Fract/Exp String To Number(string=w2015) -> (number=w2012:dbl)  [unwired: 3 in, 1 out]
                      n992 = Divide(x=w2017, y=100.0) -> (x/y=w2004:dbl)
                      n993 = Multiply(x=w2004, y=w2003) -> (x*y=w2002:dbl)
                      n994 = Add(x=w2003, y=w2002) -> (x+y=w2014:dbl)
                      n995 = Subtract(x=w2003, y=w2002) -> (x-y=w2013:dbl)
                      n996 = In Range and Coerce(upper limit=w2014, x=w2012, lower limit=w2013) -> (In Range?=w2011:bool)  [unwired: 1 out]
                      n997 = Select(t="P", s=w2011, f="F") -> (s? t:f=w2006:string)
                      n998 = Replace Array Subset(array=w2022, new element #1=w2015, index (row) #1=w2008, index (col) #1=w2023, new element #2=w2006, index (row) #2=w2008, index (col) #2=5 ("disabled index (col)")) -> (w2005:string[][])
                    }
                    frame 13 {
                      w2042 = 3  # tol
                      w2043 = 2  # res
                      w2045 = 4  # meas
                      # "fill the P/F\ncol"
                      # "fill the meas col"
                      # "check to see\npass or fail"
                      # "pull out resistor\nvalue and tolerance\nto find limits"
                      n999 = Index Array(array=w2044, index (row) #1=w2030, index (col) #1=w2043, index (row) #2=w2030, index (col) #2=w2042) -> (element #1=w2041:string, element #2=w2040:string)
                      n1000 = Fract/Exp String To Number(string=w2041) -> (number=w2025:dbl)  [unwired: 3 in, 1 out]
                      n1001 = Fract/Exp String To Number(string=w2040) -> (number=w2039:dbl)  [unwired: 3 in, 1 out]
                      n1002 = Fract/Exp String To Number(string=w2037) -> (number=w2034:dbl)  [unwired: 3 in, 1 out]
                      n1003 = Divide(x=w2039, y=100.0) -> (x/y=w2026:dbl)
                      n1004 = Multiply(x=w2026, y=w2025) -> (x*y=w2024:dbl)
                      n1005 = Add(x=w2025, y=w2024) -> (x+y=w2036:dbl)
                      n1006 = Subtract(x=w2025, y=w2024) -> (x-y=w2035:dbl)
                      n1007 = In Range and Coerce(upper limit=w2036, x=w2034, lower limit=w2035) -> (In Range?=w2033:bool)  [unwired: 1 out]
                      n1008 = Select(t="P", s=w2033, f="F") -> (s? t:f=w2028:string)
                      n1009 = Replace Array Subset(array=w2044, new element #1=w2037, index (row) #1=w2030, index (col) #1=w2045, new element #2=w2028, index (row) #2=w2030, index (col) #2=5 ("disabled index (col)")) -> (w2027:string[][])
                    }
                    frame 14 {
                      w2064 = 3  # tol
                      w2065 = 2  # res
                      w2067 = 4  # meas
                      # "fill the P/F\ncol"
                      # "fill the meas col"
                      # "check to see\npass or fail"
                      # "pull out resistor\nvalue and tolerance\nto find limits"
                      n1010 = Index Array(array=w2066, index (row) #1=w2052, index (col) #1=w2065, index (row) #2=w2052, index (col) #2=w2064) -> (element #1=w2063:string, element #2=w2062:string)
                      n1011 = Fract/Exp String To Number(string=w2063) -> (number=w2047:dbl)  [unwired: 3 in, 1 out]
                      n1012 = Fract/Exp String To Number(string=w2062) -> (number=w2061:dbl)  [unwired: 3 in, 1 out]
                      n1013 = Fract/Exp String To Number(string=w2059) -> (number=w2056:dbl)  [unwired: 3 in, 1 out]
                      n1014 = Divide(x=w2061, y=100.0) -> (x/y=w2048:dbl)
                      n1015 = Multiply(x=w2048, y=w2047) -> (x*y=w2046:dbl)
                      n1016 = Add(x=w2047, y=w2046) -> (x+y=w2058:dbl)
                      n1017 = Subtract(x=w2047, y=w2046) -> (x-y=w2057:dbl)
                      n1018 = In Range and Coerce(upper limit=w2058, x=w2056, lower limit=w2057) -> (In Range?=w2055:bool)  [unwired: 1 out]
                      n1019 = Select(t="P", s=w2055, f="F") -> (s? t:f=w2050:string)
                      n1020 = Replace Array Subset(array=w2066, new element #1=w2059, index (row) #1=w2052, index (col) #1=w2067, new element #2=w2050, index (row) #2=w2052, index (col) #2=5 ("disabled index (col)")) -> (w2049:string[][])
                    }
                    frame 15 {
                      w2086 = 3  # tol
                      w2087 = 2  # res
                      w2089 = 4  # meas
                      # "fill the P/F\ncol"
                      # "fill the meas col"
                      # "check to see\npass or fail"
                      # "pull out resistor\nvalue and tolerance\nto find limits"
                      n1021 = Index Array(array=w2088, index (row) #1=w2074, index (col) #1=w2087, index (row) #2=w2074, index (col) #2=w2086) -> (element #1=w2085:string, element #2=w2084:string)
                      n1022 = Fract/Exp String To Number(string=w2085) -> (number=w2069:dbl)  [unwired: 3 in, 1 out]
                      n1023 = Fract/Exp String To Number(string=w2084) -> (number=w2083:dbl)  [unwired: 3 in, 1 out]
                      n1024 = Fract/Exp String To Number(string=w2081) -> (number=w2078:dbl)  [unwired: 3 in, 1 out]
                      n1025 = Divide(x=w2083, y=100.0) -> (x/y=w2070:dbl)
                      n1026 = Multiply(x=w2070, y=w2069) -> (x*y=w2068:dbl)
                      n1027 = Add(x=w2069, y=w2068) -> (x+y=w2080:dbl)
                      n1028 = Subtract(x=w2069, y=w2068) -> (x-y=w2079:dbl)
                      n1029 = In Range and Coerce(upper limit=w2080, x=w2078, lower limit=w2079) -> (In Range?=w2077:bool)  [unwired: 1 out]
                      n1030 = Select(t="P", s=w2077, f="F") -> (s? t:f=w2072:string)
                      n1031 = Replace Array Subset(array=w2088, new element #1=w2081, index (row) #1=w2074, index (col) #1=w2089, new element #2=w2072, index (row) #2=w2074, index (col) #2=5 ("disabled index (col)")) -> (w2071:string[][])
                    }
                    frame 16 {
                      w2108 = 3  # tol
                      w2109 = 2  # res
                      w2111 = 4  # meas
                      # "fill the P/F\ncol"
                      # "fill the meas col"
                      # "check to see\npass or fail"
                      # "pull out resistor\nvalue and tolerance\nto find limits"
                      n1032 = Index Array(array=w2110, index (row) #1=w2096, index (col) #1=w2109, index (row) #2=w2096, index (col) #2=w2108) -> (element #1=w2107:string, element #2=w2106:string)
                      n1033 = Fract/Exp String To Number(string=w2107) -> (number=w2091:dbl)  [unwired: 3 in, 1 out]
                      n1034 = Fract/Exp String To Number(string=w2106) -> (number=w2105:dbl)  [unwired: 3 in, 1 out]
                      n1035 = Fract/Exp String To Number(string=w2103) -> (number=w2100:dbl)  [unwired: 3 in, 1 out]
                      n1036 = Divide(x=w2105, y=100.0) -> (x/y=w2092:dbl)
                      n1037 = Multiply(x=w2092, y=w2091) -> (x*y=w2090:dbl)
                      n1038 = Add(x=w2091, y=w2090) -> (x+y=w2102:dbl)
                      n1039 = Subtract(x=w2091, y=w2090) -> (x-y=w2101:dbl)
                      n1040 = In Range and Coerce(upper limit=w2102, x=w2100, lower limit=w2101) -> (In Range?=w2099:bool)  [unwired: 1 out]
                      n1041 = Select(t="P", s=w2099, f="F") -> (s? t:f=w2094:string)
                      n1042 = Replace Array Subset(array=w2110, new element #1=w2103, index (row) #1=w2096, index (col) #1=w2111, new element #2=w2094, index (row) #2=w2096, index (col) #2=5 ("disabled index (col)")) -> (w2093:string[][])
                    }
                    frame 17 {
                      w2130 = 3  # tol
                      w2131 = 2  # res
                      w2133 = 4  # meas
                      # "fill the P/F\ncol"
                      # "fill the meas col"
                      # "check to see\npass or fail"
                      # "pull out resistor\nvalue and tolerance\nto find limits"
                      n1043 = Index Array(array=w2132, index (row) #1=w2118, index (col) #1=w2131, index (row) #2=w2118, index (col) #2=w2130) -> (element #1=w2129:string, element #2=w2128:string)
                      n1044 = Fract/Exp String To Number(string=w2129) -> (number=w2113:dbl)  [unwired: 3 in, 1 out]
                      n1045 = Fract/Exp String To Number(string=w2128) -> (number=w2127:dbl)  [unwired: 3 in, 1 out]
                      n1046 = Fract/Exp String To Number(string=w2125) -> (number=w2122:dbl)  [unwired: 3 in, 1 out]
                      n1047 = Divide(x=w2127, y=100.0) -> (x/y=w2114:dbl)
                      n1048 = Multiply(x=w2114, y=w2113) -> (x*y=w2112:dbl)
                      n1049 = Add(x=w2113, y=w2112) -> (x+y=w2124:dbl)
                      n1050 = Subtract(x=w2113, y=w2112) -> (x-y=w2123:dbl)
                      n1051 = In Range and Coerce(upper limit=w2124, x=w2122, lower limit=w2123) -> (In Range?=w2121:bool)  [unwired: 1 out]
                      n1052 = Select(t="P", s=w2121, f="F") -> (s? t:f=w2116:string)
                      n1053 = Replace Array Subset(array=w2132, new element #1=w2125, index (row) #1=w2118, index (col) #1=w2133, new element #2=w2116, index (row) #2=w2118, index (col) #2=5 ("disabled index (col)")) -> (w2115:string[][])
                    }
                    frame 18 {
                      w2152 = 3  # tol
                      w2153 = 2  # res
                      w2155 = 4  # meas
                      # "fill the P/F\ncol"
                      # "fill the meas col"
                      # "check to see\npass or fail"
                      # "pull out resistor\nvalue and tolerance\nto find limits"
                      n1054 = Index Array(array=w2154, index (row) #1=w2140, index (col) #1=w2153, index (row) #2=w2140, index (col) #2=w2152) -> (element #1=w2151:string, element #2=w2150:string)
                      n1055 = Fract/Exp String To Number(string=w2151) -> (number=w2135:dbl)  [unwired: 3 in, 1 out]
                      n1056 = Fract/Exp String To Number(string=w2150) -> (number=w2149:dbl)  [unwired: 3 in, 1 out]
                      n1057 = Fract/Exp String To Number(string=w2147) -> (number=w2144:dbl)  [unwired: 3 in, 1 out]
                      n1058 = Divide(x=w2149, y=100.0) -> (x/y=w2136:dbl)
                      n1059 = Multiply(x=w2136, y=w2135) -> (x*y=w2134:dbl)
                      n1060 = Add(x=w2135, y=w2134) -> (x+y=w2146:dbl)
                      n1061 = Subtract(x=w2135, y=w2134) -> (x-y=w2145:dbl)
                      n1062 = In Range and Coerce(upper limit=w2146, x=w2144, lower limit=w2145) -> (In Range?=w2143:bool)  [unwired: 1 out]
                      n1063 = Select(t="P", s=w2143, f="F") -> (s? t:f=w2138:string)
                      n1064 = Replace Array Subset(array=w2154, new element #1=w2147, index (row) #1=w2140, index (col) #1=w2155, new element #2=w2138, index (row) #2=w2140, index (col) #2=5 ("disabled index (col)")) -> (w2137:string[][])
                    }
                    frame 19 {
                      w2174 = 3  # tol
                      w2175 = 2  # res
                      w2177 = 4  # meas
                      # "fill the P/F\ncol"
                      # "fill the meas col"
                      # "check to see\npass or fail"
                      # "pull out resistor\nvalue and tolerance\nto find limits"
                      n1065 = Index Array(array=w2176, index (row) #1=w2162, index (col) #1=w2175, index (row) #2=w2162, index (col) #2=w2174) -> (element #1=w2173:string, element #2=w2172:string)
                      n1066 = Fract/Exp String To Number(string=w2173) -> (number=w2157:dbl)  [unwired: 3 in, 1 out]
                      n1067 = Fract/Exp String To Number(string=w2172) -> (number=w2171:dbl)  [unwired: 3 in, 1 out]
                      n1068 = Fract/Exp String To Number(string=w2169) -> (number=w2166:dbl)  [unwired: 3 in, 1 out]
                      n1069 = Divide(x=w2171, y=100.0) -> (x/y=w2158:dbl)
                      n1070 = Multiply(x=w2158, y=w2157) -> (x*y=w2156:dbl)
                      n1071 = Add(x=w2157, y=w2156) -> (x+y=w2168:dbl)
                      n1072 = Subtract(x=w2157, y=w2156) -> (x-y=w2167:dbl)
                      n1073 = In Range and Coerce(upper limit=w2168, x=w2166, lower limit=w2167) -> (In Range?=w2165:bool)  [unwired: 1 out]
                      n1074 = Select(t="P", s=w2165, f="F") -> (s? t:f=w2160:string)
                      n1075 = Replace Array Subset(array=w2176, new element #1=w2169, index (row) #1=w2162, index (col) #1=w2177, new element #2=w2160, index (row) #2=w2162, index (col) #2=5 ("disabled index (col)")) -> (w2159:string[][])
                    }
                    frame 20 {
                      w2196 = 3  # tol
                      w2197 = 2  # res
                      w2199 = 4  # meas
                      # "fill the P/F\ncol"
                      # "fill the meas col"
                      # "check to see\npass or fail"
                      # "pull out resistor\nvalue and tolerance\nto find limits"
                      n1076 = Index Array(array=w2198, index (row) #1=w2184, index (col) #1=w2197, index (row) #2=w2184, index (col) #2=w2196) -> (element #1=w2195:string, element #2=w2194:string)
                      n1077 = Fract/Exp String To Number(string=w2195) -> (number=w2179:dbl)  [unwired: 3 in, 1 out]
                      n1078 = Fract/Exp String To Number(string=w2194) -> (number=w2193:dbl)  [unwired: 3 in, 1 out]
                      n1079 = Fract/Exp String To Number(string=w2191) -> (number=w2188:dbl)  [unwired: 3 in, 1 out]
                      n1080 = Divide(x=w2193, y=100.0) -> (x/y=w2180:dbl)
                      n1081 = Multiply(x=w2180, y=w2179) -> (x*y=w2178:dbl)
                      n1082 = Add(x=w2179, y=w2178) -> (x+y=w2190:dbl)
                      n1083 = Subtract(x=w2179, y=w2178) -> (x-y=w2189:dbl)
                      n1084 = In Range and Coerce(upper limit=w2190, x=w2188, lower limit=w2189) -> (In Range?=w2187:bool)  [unwired: 1 out]
                      n1085 = Select(t="P", s=w2187, f="F") -> (s? t:f=w2182:string)
                      n1086 = Replace Array Subset(array=w2198, new element #1=w2191, index (row) #1=w2184, index (col) #1=w2199, new element #2=w2182, index (row) #2=w2184, index (col) #2=5 ("disabled index (col)")) -> (w2181:string[][])
                    }
                    frame 21 {
                      w2218 = 3  # tol
                      w2219 = 2  # res
                      w2221 = 4  # meas
                      # "fill the P/F\ncol"
                      # "fill the meas col"
                      # "check to see\npass or fail"
                      # "pull out resistor\nvalue and tolerance\nto find limits"
                      n1087 = Index Array(array=w2220, index (row) #1=w2206, index (col) #1=w2219, index (row) #2=w2206, index (col) #2=w2218) -> (element #1=w2217:string, element #2=w2216:string)
                      n1088 = Fract/Exp String To Number(string=w2217) -> (number=w2201:dbl)  [unwired: 3 in, 1 out]
                      n1089 = Fract/Exp String To Number(string=w2216) -> (number=w2215:dbl)  [unwired: 3 in, 1 out]
                      n1090 = Fract/Exp String To Number(string=w2213) -> (number=w2210:dbl)  [unwired: 3 in, 1 out]
                      n1091 = Divide(x=w2215, y=100.0) -> (x/y=w2202:dbl)
                      n1092 = Multiply(x=w2202, y=w2201) -> (x*y=w2200:dbl)
                      n1093 = Add(x=w2201, y=w2200) -> (x+y=w2212:dbl)
                      n1094 = Subtract(x=w2201, y=w2200) -> (x-y=w2211:dbl)
                      n1095 = In Range and Coerce(upper limit=w2212, x=w2210, lower limit=w2211) -> (In Range?=w2209:bool)  [unwired: 1 out]
                      n1096 = Select(t="P", s=w2209, f="F") -> (s? t:f=w2204:string)
                      n1097 = Replace Array Subset(array=w2220, new element #1=w2213, index (row) #1=w2206, index (col) #1=w2221, new element #2=w2204, index (row) #2=w2206, index (col) #2=5 ("disabled index (col)")) -> (w2203:string[][])
                    }
                    frame 22 {
                      w2240 = 3  # tol
                      w2241 = 2  # res
                      w2243 = 4  # meas
                      # "fill the P/F\ncol"
                      # "fill the meas col"
                      # "check to see\npass or fail"
                      # "pull out resistor\nvalue and tolerance\nto find limits"
                      n1098 = Index Array(array=w2242, index (row) #1=w2228, index (col) #1=w2241, index (row) #2=w2228, index (col) #2=w2240) -> (element #1=w2239:string, element #2=w2238:string)
                      n1099 = Fract/Exp String To Number(string=w2239) -> (number=w2223:dbl)  [unwired: 3 in, 1 out]
                      n1100 = Fract/Exp String To Number(string=w2238) -> (number=w2237:dbl)  [unwired: 3 in, 1 out]
                      n1101 = Fract/Exp String To Number(string=w2235) -> (number=w2232:dbl)  [unwired: 3 in, 1 out]
                      n1102 = Divide(x=w2237, y=100.0) -> (x/y=w2224:dbl)
                      n1103 = Multiply(x=w2224, y=w2223) -> (x*y=w2222:dbl)
                      n1104 = Add(x=w2223, y=w2222) -> (x+y=w2234:dbl)
                      n1105 = Subtract(x=w2223, y=w2222) -> (x-y=w2233:dbl)
                      n1106 = In Range and Coerce(upper limit=w2234, x=w2232, lower limit=w2233) -> (In Range?=w2231:bool)  [unwired: 1 out]
                      n1107 = Select(t="P", s=w2231, f="F") -> (s? t:f=w2226:string)
                      n1108 = Replace Array Subset(array=w2242, new element #1=w2235, index (row) #1=w2228, index (col) #1=w2243, new element #2=w2226, index (row) #2=w2228, index (col) #2=5 ("disabled index (col)")) -> (w2225:string[][])
                    }
                    frame 23 {
                      w2262 = 3  # tol
                      w2263 = 2  # res
                      w2265 = 4  # meas
                      # "fill the P/F\ncol"
                      # "fill the meas col"
                      # "check to see\npass or fail"
                      # "pull out resistor\nvalue and tolerance\nto find limits"
                      n1109 = Index Array(array=w2264, index (row) #1=w2250, index (col) #1=w2263, index (row) #2=w2250, index (col) #2=w2262) -> (element #1=w2261:string, element #2=w2260:string)
                      n1110 = Fract/Exp String To Number(string=w2261) -> (number=w2245:dbl)  [unwired: 3 in, 1 out]
                      n1111 = Fract/Exp String To Number(string=w2260) -> (number=w2259:dbl)  [unwired: 3 in, 1 out]
                      n1112 = Fract/Exp String To Number(string=w2257) -> (number=w2254:dbl)  [unwired: 3 in, 1 out]
                      n1113 = Divide(x=w2259, y=100.0) -> (x/y=w2246:dbl)
                      n1114 = Multiply(x=w2246, y=w2245) -> (x*y=w2244:dbl)
                      n1115 = Add(x=w2245, y=w2244) -> (x+y=w2256:dbl)
                      n1116 = Subtract(x=w2245, y=w2244) -> (x-y=w2255:dbl)
                      n1117 = In Range and Coerce(upper limit=w2256, x=w2254, lower limit=w2255) -> (In Range?=w2253:bool)  [unwired: 1 out]
                      n1118 = Select(t="P", s=w2253, f="F") -> (s? t:f=w2248:string)
                      n1119 = Replace Array Subset(array=w2264, new element #1=w2257, index (row) #1=w2250, index (col) #1=w2265, new element #2=w2248, index (row) #2=w2250, index (col) #2=5 ("disabled index (col)")) -> (w2247:string[][])
                    }
                    frame 24 {
                      w2284 = 3  # tol
                      w2285 = 2  # res
                      w2287 = 4  # meas
                      # "fill the P/F\ncol"
                      # "fill the meas col"
                      # "check to see\npass or fail"
                      # "pull out resistor\nvalue and tolerance\nto find limits"
                      n1120 = Index Array(array=w2286, index (row) #1=w2272, index (col) #1=w2285, index (row) #2=w2272, index (col) #2=w2284) -> (element #1=w2283:string, element #2=w2282:string)
                      n1121 = Fract/Exp String To Number(string=w2283) -> (number=w2267:dbl)  [unwired: 3 in, 1 out]
                      n1122 = Fract/Exp String To Number(string=w2282) -> (number=w2281:dbl)  [unwired: 3 in, 1 out]
                      n1123 = Fract/Exp String To Number(string=w2279) -> (number=w2276:dbl)  [unwired: 3 in, 1 out]
                      n1124 = Divide(x=w2281, y=100.0) -> (x/y=w2268:dbl)
                      n1125 = Multiply(x=w2268, y=w2267) -> (x*y=w2266:dbl)
                      n1126 = Add(x=w2267, y=w2266) -> (x+y=w2278:dbl)
                      n1127 = Subtract(x=w2267, y=w2266) -> (x-y=w2277:dbl)
                      n1128 = In Range and Coerce(upper limit=w2278, x=w2276, lower limit=w2277) -> (In Range?=w2275:bool)  [unwired: 1 out]
                      n1129 = Select(t="P", s=w2275, f="F") -> (s? t:f=w2270:string)
                      n1130 = Replace Array Subset(array=w2286, new element #1=w2279, index (row) #1=w2272, index (col) #1=w2287, new element #2=w2270, index (row) #2=w2272, index (col) #2=5 ("disabled index (col)")) -> (w2269:string[][])
                    }
                    frame 25 {
                      w2306 = 3  # tol
                      w2307 = 2  # res
                      w2309 = 4  # meas
                      # "fill the P/F\ncol"
                      # "fill the meas col"
                      # "check to see\npass or fail"
                      # "pull out resistor\nvalue and tolerance\nto find limits"
                      n1131 = Index Array(array=w2308, index (row) #1=w2294, index (col) #1=w2307, index (row) #2=w2294, index (col) #2=w2306) -> (element #1=w2305:string, element #2=w2304:string)
                      n1132 = Fract/Exp String To Number(string=w2305) -> (number=w2289:dbl)  [unwired: 3 in, 1 out]
                      n1133 = Fract/Exp String To Number(string=w2304) -> (number=w2303:dbl)  [unwired: 3 in, 1 out]
                      n1134 = Fract/Exp String To Number(string=w2301) -> (number=w2298:dbl)  [unwired: 3 in, 1 out]
                      n1135 = Divide(x=w2303, y=100.0) -> (x/y=w2290:dbl)
                      n1136 = Multiply(x=w2290, y=w2289) -> (x*y=w2288:dbl)
                      n1137 = Add(x=w2289, y=w2288) -> (x+y=w2300:dbl)
                      n1138 = Subtract(x=w2289, y=w2288) -> (x-y=w2299:dbl)
                      n1139 = In Range and Coerce(upper limit=w2300, x=w2298, lower limit=w2299) -> (In Range?=w2297:bool)  [unwired: 1 out]
                      n1140 = Select(t="P", s=w2297, f="F") -> (s? t:f=w2292:string)
                      n1141 = Replace Array Subset(array=w2308, new element #1=w2301, index (row) #1=w2294, index (col) #1=w2309, new element #2=w2292, index (row) #2=w2294, index (col) #2=5 ("disabled index (col)")) -> (w2291:string[][])
                    }
                    frame 26 {
                      w2328 = 3  # tol
                      w2329 = 2  # res
                      w2331 = 4  # meas
                      # "fill the P/F\ncol"
                      # "fill the meas col"
                      # "check to see\npass or fail"
                      # "pull out resistor\nvalue and tolerance\nto find limits"
                      n1142 = Index Array(array=w2330, index (row) #1=w2316, index (col) #1=w2329, index (row) #2=w2316, index (col) #2=w2328) -> (element #1=w2327:string, element #2=w2326:string)
                      n1143 = Fract/Exp String To Number(string=w2327) -> (number=w2311:dbl)  [unwired: 3 in, 1 out]
                      n1144 = Fract/Exp String To Number(string=w2326) -> (number=w2325:dbl)  [unwired: 3 in, 1 out]
                      n1145 = Fract/Exp String To Number(string=w2323) -> (number=w2320:dbl)  [unwired: 3 in, 1 out]
                      n1146 = Divide(x=w2325, y=100.0) -> (x/y=w2312:dbl)
                      n1147 = Multiply(x=w2312, y=w2311) -> (x*y=w2310:dbl)
                      n1148 = Add(x=w2311, y=w2310) -> (x+y=w2322:dbl)
                      n1149 = Subtract(x=w2311, y=w2310) -> (x-y=w2321:dbl)
                      n1150 = In Range and Coerce(upper limit=w2322, x=w2320, lower limit=w2321) -> (In Range?=w2319:bool)  [unwired: 1 out]
                      n1151 = Select(t="P", s=w2319, f="F") -> (s? t:f=w2314:string)
                      n1152 = Replace Array Subset(array=w2330, new element #1=w2323, index (row) #1=w2316, index (col) #1=w2331, new element #2=w2314, index (row) #2=w2316, index (col) #2=5 ("disabled index (col)")) -> (w2313:string[][])
                    }
                    frame 27 {
                      w2350 = 3  # tol
                      w2351 = 2  # res
                      w2353 = 4  # meas
                      # "fill the P/F\ncol"
                      # "fill the meas col"
                      # "check to see\npass or fail"
                      # "pull out resistor\nvalue and tolerance\nto find limits"
                      n1153 = Index Array(array=w2352, index (row) #1=w2338, index (col) #1=w2351, index (row) #2=w2338, index (col) #2=w2350) -> (element #1=w2349:string, element #2=w2348:string)
                      n1154 = Fract/Exp String To Number(string=w2349) -> (number=w2333:dbl)  [unwired: 3 in, 1 out]
                      n1155 = Fract/Exp String To Number(string=w2348) -> (number=w2347:dbl)  [unwired: 3 in, 1 out]
                      n1156 = Fract/Exp String To Number(string=w2345) -> (number=w2342:dbl)  [unwired: 3 in, 1 out]
                      n1157 = Divide(x=w2347, y=100.0) -> (x/y=w2334:dbl)
                      n1158 = Multiply(x=w2334, y=w2333) -> (x*y=w2332:dbl)
                      n1159 = Add(x=w2333, y=w2332) -> (x+y=w2344:dbl)
                      n1160 = Subtract(x=w2333, y=w2332) -> (x-y=w2343:dbl)
                      n1161 = In Range and Coerce(upper limit=w2344, x=w2342, lower limit=w2343) -> (In Range?=w2341:bool)  [unwired: 1 out]
                      n1162 = Select(t="P", s=w2341, f="F") -> (s? t:f=w2336:string)
                      n1163 = Replace Array Subset(array=w2352, new element #1=w2345, index (row) #1=w2338, index (col) #1=w2353, new element #2=w2336, index (row) #2=w2338, index (col) #2=5 ("disabled index (col)")) -> (w2335:string[][])
                    }
                    frame 28 {
                      w2372 = 3  # tol
                      w2373 = 2  # res
                      w2375 = 4  # meas
                      # "fill the P/F\ncol"
                      # "fill the meas col"
                      # "check to see\npass or fail"
                      # "pull out resistor\nvalue and tolerance\nto find limits"
                      n1164 = Index Array(array=w2374, index (row) #1=w2360, index (col) #1=w2373, index (row) #2=w2360, index (col) #2=w2372) -> (element #1=w2371:string, element #2=w2370:string)
                      n1165 = Fract/Exp String To Number(string=w2371) -> (number=w2355:dbl)  [unwired: 3 in, 1 out]
                      n1166 = Fract/Exp String To Number(string=w2370) -> (number=w2369:dbl)  [unwired: 3 in, 1 out]
                      n1167 = Fract/Exp String To Number(string=w2367) -> (number=w2364:dbl)  [unwired: 3 in, 1 out]
                      n1168 = Divide(x=w2369, y=100.0) -> (x/y=w2356:dbl)
                      n1169 = Multiply(x=w2356, y=w2355) -> (x*y=w2354:dbl)
                      n1170 = Add(x=w2355, y=w2354) -> (x+y=w2366:dbl)
                      n1171 = Subtract(x=w2355, y=w2354) -> (x-y=w2365:dbl)
                      n1172 = In Range and Coerce(upper limit=w2366, x=w2364, lower limit=w2365) -> (In Range?=w2363:bool)  [unwired: 1 out]
                      n1173 = Select(t="P", s=w2363, f="F") -> (s? t:f=w2358:string)
                      n1174 = Replace Array Subset(array=w2374, new element #1=w2367, index (row) #1=w2360, index (col) #1=w2375, new element #2=w2358, index (row) #2=w2360, index (col) #2=5 ("disabled index (col)")) -> (w2357:string[][])
                    }
                    frame 29 {
                      w2394 = 3  # tol
                      w2395 = 2  # res
                      w2397 = 4  # meas
                      # "fill the P/F\ncol"
                      # "fill the meas col"
                      # "check to see\npass or fail"
                      # "pull out resistor\nvalue and tolerance\nto find limits"
                      n1175 = Index Array(array=w2396, index (row) #1=w2382, index (col) #1=w2395, index (row) #2=w2382, index (col) #2=w2394) -> (element #1=w2393:string, element #2=w2392:string)
                      n1176 = Fract/Exp String To Number(string=w2393) -> (number=w2377:dbl)  [unwired: 3 in, 1 out]
                      n1177 = Fract/Exp String To Number(string=w2392) -> (number=w2391:dbl)  [unwired: 3 in, 1 out]
                      n1178 = Fract/Exp String To Number(string=w2389) -> (number=w2386:dbl)  [unwired: 3 in, 1 out]
                      n1179 = Divide(x=w2391, y=100.0) -> (x/y=w2378:dbl)
                      n1180 = Multiply(x=w2378, y=w2377) -> (x*y=w2376:dbl)
                      n1181 = Add(x=w2377, y=w2376) -> (x+y=w2388:dbl)
                      n1182 = Subtract(x=w2377, y=w2376) -> (x-y=w2387:dbl)
                      n1183 = In Range and Coerce(upper limit=w2388, x=w2386, lower limit=w2387) -> (In Range?=w2385:bool)  [unwired: 1 out]
                      n1184 = Select(t="P", s=w2385, f="F") -> (s? t:f=w2380:string)
                      n1185 = Replace Array Subset(array=w2396, new element #1=w2389, index (row) #1=w2382, index (col) #1=w2397, new element #2=w2380, index (row) #2=w2382, index (col) #2=5 ("disabled index (col)")) -> (w2379:string[][])
                    }
                    frame 30 {
                      w2416 = 3  # tol
                      w2417 = 2  # res
                      w2419 = 4  # meas
                      # "fill the P/F\ncol"
                      # "fill the meas col"
                      # "check to see\npass or fail"
                      # "pull out resistor\nvalue and tolerance\nto find limits"
                      n1186 = Index Array(array=w2418, index (row) #1=w2404, index (col) #1=w2417, index (row) #2=w2404, index (col) #2=w2416) -> (element #1=w2415:string, element #2=w2414:string)
                      n1187 = Fract/Exp String To Number(string=w2415) -> (number=w2399:dbl)  [unwired: 3 in, 1 out]
                      n1188 = Fract/Exp String To Number(string=w2414) -> (number=w2413:dbl)  [unwired: 3 in, 1 out]
                      n1189 = Fract/Exp String To Number(string=w2411) -> (number=w2408:dbl)  [unwired: 3 in, 1 out]
                      n1190 = Divide(x=w2413, y=100.0) -> (x/y=w2400:dbl)
                      n1191 = Multiply(x=w2400, y=w2399) -> (x*y=w2398:dbl)
                      n1192 = Add(x=w2399, y=w2398) -> (x+y=w2410:dbl)
                      n1193 = Subtract(x=w2399, y=w2398) -> (x-y=w2409:dbl)
                      n1194 = In Range and Coerce(upper limit=w2410, x=w2408, lower limit=w2409) -> (In Range?=w2407:bool)  [unwired: 1 out]
                      n1195 = Select(t="P", s=w2407, f="F") -> (s? t:f=w2402:string)
                      n1196 = Replace Array Subset(array=w2418, new element #1=w2411, index (row) #1=w2404, index (col) #1=w2419, new element #2=w2402, index (row) #2=w2404, index (col) #2=5 ("disabled index (col)")) -> (w2401:string[][])
                    }
                    frame 31 {
                      w2438 = 3  # tol
                      w2439 = 2  # res
                      w2441 = 4  # meas
                      # "fill the P/F\ncol"
                      # "fill the meas col"
                      # "check to see\npass or fail"
                      # "pull out resistor\nvalue and tolerance\nto find limits"
                      n1197 = Index Array(array=w2440, index (row) #1=w2426, index (col) #1=w2439, index (row) #2=w2426, index (col) #2=w2438) -> (element #1=w2437:string, element #2=w2436:string)
                      n1198 = Fract/Exp String To Number(string=w2437) -> (number=w2421:dbl)  [unwired: 3 in, 1 out]
                      n1199 = Fract/Exp String To Number(string=w2436) -> (number=w2435:dbl)  [unwired: 3 in, 1 out]
                      n1200 = Fract/Exp String To Number(string=w2433) -> (number=w2430:dbl)  [unwired: 3 in, 1 out]
                      n1201 = Divide(x=w2435, y=100.0) -> (x/y=w2422:dbl)
                      n1202 = Multiply(x=w2422, y=w2421) -> (x*y=w2420:dbl)
                      n1203 = Add(x=w2421, y=w2420) -> (x+y=w2432:dbl)
                      n1204 = Subtract(x=w2421, y=w2420) -> (x-y=w2431:dbl)
                      n1205 = In Range and Coerce(upper limit=w2432, x=w2430, lower limit=w2431) -> (In Range?=w2429:bool)  [unwired: 1 out]
                      n1206 = Select(t="P", s=w2429, f="F") -> (s? t:f=w2424:string)
                      n1207 = Replace Array Subset(array=w2440, new element #1=w2433, index (row) #1=w2426, index (col) #1=w2441, new element #2=w2424, index (row) #2=w2426, index (col) #2=5 ("disabled index (col)")) -> (w2423:string[][])
                    }
                    frame 32 {
                      w2460 = 3  # tol
                      w2461 = 2  # res
                      w2463 = 4  # meas
                      # "fill the P/F\ncol"
                      # "fill the meas col"
                      # "check to see\npass or fail"
                      # "pull out resistor\nvalue and tolerance\nto find limits"
                      n1208 = Index Array(array=w2462, index (row) #1=w2448, index (col) #1=w2461, index (row) #2=w2448, index (col) #2=w2460) -> (element #1=w2459:string, element #2=w2458:string)
                      n1209 = Fract/Exp String To Number(string=w2459) -> (number=w2443:dbl)  [unwired: 3 in, 1 out]
                      n1210 = Fract/Exp String To Number(string=w2458) -> (number=w2457:dbl)  [unwired: 3 in, 1 out]
                      n1211 = Fract/Exp String To Number(string=w2455) -> (number=w2452:dbl)  [unwired: 3 in, 1 out]
                      n1212 = Divide(x=w2457, y=100.0) -> (x/y=w2444:dbl)
                      n1213 = Multiply(x=w2444, y=w2443) -> (x*y=w2442:dbl)
                      n1214 = Add(x=w2443, y=w2442) -> (x+y=w2454:dbl)
                      n1215 = Subtract(x=w2443, y=w2442) -> (x-y=w2453:dbl)
                      n1216 = In Range and Coerce(upper limit=w2454, x=w2452, lower limit=w2453) -> (In Range?=w2451:bool)  [unwired: 1 out]
                      n1217 = Select(t="P", s=w2451, f="F") -> (s? t:f=w2446:string)
                      n1218 = Replace Array Subset(array=w2462, new element #1=w2455, index (row) #1=w2448, index (col) #1=w2463, new element #2=w2446, index (row) #2=w2448, index (col) #2=5 ("disabled index (col)")) -> (w2445:string[][])
                    }
                    frame 33 {
                      w2482 = 3  # tol
                      w2483 = 2  # res
                      w2485 = 4  # meas
                      # "fill the P/F\ncol"
                      # "fill the meas col"
                      # "check to see\npass or fail"
                      # "pull out resistor\nvalue and tolerance\nto find limits"
                      n1219 = Index Array(array=w2484, index (row) #1=w2470, index (col) #1=w2483, index (row) #2=w2470, index (col) #2=w2482) -> (element #1=w2481:string, element #2=w2480:string)
                      n1220 = Fract/Exp String To Number(string=w2481) -> (number=w2465:dbl)  [unwired: 3 in, 1 out]
                      n1221 = Fract/Exp String To Number(string=w2480) -> (number=w2479:dbl)  [unwired: 3 in, 1 out]
                      n1222 = Fract/Exp String To Number(string=w2477) -> (number=w2474:dbl)  [unwired: 3 in, 1 out]
                      n1223 = Divide(x=w2479, y=100.0) -> (x/y=w2466:dbl)
                      n1224 = Multiply(x=w2466, y=w2465) -> (x*y=w2464:dbl)
                      n1225 = Add(x=w2465, y=w2464) -> (x+y=w2476:dbl)
                      n1226 = Subtract(x=w2465, y=w2464) -> (x-y=w2475:dbl)
                      n1227 = In Range and Coerce(upper limit=w2476, x=w2474, lower limit=w2475) -> (In Range?=w2473:bool)  [unwired: 1 out]
                      n1228 = Select(t="P", s=w2473, f="F") -> (s? t:f=w2468:string)
                      n1229 = Replace Array Subset(array=w2484, new element #1=w2477, index (row) #1=w2470, index (col) #1=w2485, new element #2=w2468, index (row) #2=w2470, index (col) #2=5 ("disabled index (col)")) -> (w2467:string[][])
                    }
                    frame 34 {
                      w2504 = 3  # tol
                      w2505 = 2  # res
                      w2507 = 4  # meas
                      # "fill the P/F\ncol"
                      # "fill the meas col"
                      # "check to see\npass or fail"
                      # "pull out resistor\nvalue and tolerance\nto find limits"
                      n1230 = Index Array(array=w2506, index (row) #1=w2492, index (col) #1=w2505, index (row) #2=w2492, index (col) #2=w2504) -> (element #1=w2503:string, element #2=w2502:string)
                      n1231 = Fract/Exp String To Number(string=w2503) -> (number=w2487:dbl)  [unwired: 3 in, 1 out]
                      n1232 = Fract/Exp String To Number(string=w2502) -> (number=w2501:dbl)  [unwired: 3 in, 1 out]
                      n1233 = Fract/Exp String To Number(string=w2499) -> (number=w2496:dbl)  [unwired: 3 in, 1 out]
                      n1234 = Divide(x=w2501, y=100.0) -> (x/y=w2488:dbl)
                      n1235 = Multiply(x=w2488, y=w2487) -> (x*y=w2486:dbl)
                      n1236 = Add(x=w2487, y=w2486) -> (x+y=w2498:dbl)
                      n1237 = Subtract(x=w2487, y=w2486) -> (x-y=w2497:dbl)
                      n1238 = In Range and Coerce(upper limit=w2498, x=w2496, lower limit=w2497) -> (In Range?=w2495:bool)  [unwired: 1 out]
                      n1239 = Select(t="P", s=w2495, f="F") -> (s? t:f=w2490:string)
                      n1240 = Replace Array Subset(array=w2506, new element #1=w2499, index (row) #1=w2492, index (col) #1=w2507, new element #2=w2490, index (row) #2=w2492, index (col) #2=5 ("disabled index (col)")) -> (w2489:string[][])
                    }
                  }
                }
              }
              frame "10 kOhm" {
                n1241 = for {
                  tunnel: w2508 -> [w2517] mode=indexing
                  tunnel: w2510 -> [w2515]
                  shift-right: [w2513] -> w2509
                  shift-left: w2511 -> [w2516]
                  i -> [w2512]
                  # "34924A has a \nmax of 35 \nchannels."
                  n1242 = Index Array(array=w2515, index=w2512) -> (element=w2514:string)
                  n1243 = case shown="0, Default" w2517 {
                    selector: w2517 -> [w2524 w2546 w2568 w2590 w2612 w2634 w2656 w2678 w2700 w2722 w2744 w2766 w2788 w2810 w2832 w2854 w2876 w2898 w2920 w2942 w2964 w2986 w3008 w3030 w3052 w3074 w3096 w3118 w3140 w3162 w3184 w3206 w3228 w3250 w3272]
                    tunnel: w2516 -> [w2538 w2560 w2582 w2604 w2626 w2648 w2670 w2692 w2714 w2736 w2758 w2780 w2802 w2824 w2846 w2868 w2890 w2912 w2934 w2956 w2978 w3000 w3022 w3044 w3066 w3088 w3110 w3132 w3154 w3176 w3198 w3220 w3242 w3264 w3286]
                    tunnel: w2514 -> [w2531 w2553 w2575 w2597 w2619 w2641 w2663 w2685 w2707 w2729 w2751 w2773 w2795 w2817 w2839 w2861 w2883 w2905 w2927 w2949 w2971 w2993 w3015 w3037 w3059 w3081 w3103 w3125 w3147 w3169 w3191 w3213 w3235 w3257 w3279]
                    tunnel: [w2521 w2543 w2565 w2587 w2609 w2631 w2653 w2675 w2697 w2719 w2741 w2763 w2785 w2807 w2829 w2851 w2873 w2895 w2917 w2939 w2961 w2983 w3005 w3027 w3049 w3071 w3093 w3115 w3137 w3159 w3181 w3203 w3225 w3247 w3269] -> w2513
                    frame 0, Default {
                      w2536 = 3  # tol
                      w2537 = 2  # res
                      w2539 = 4  # meas
                      # "fill the P/F\ncol"
                      # "fill the meas col"
                      # "check to see\npass or fail"
                      # "pull out resistor\nvalue and tolerance\nto find limits"
                      n1244 = Index Array(array=w2538, index (row) #1=w2524, index (col) #1=w2537, index (row) #2=w2524, index (col) #2=w2536) -> (element #1=w2535:string, element #2=w2534:string)
                      n1245 = Fract/Exp String To Number(string=w2535) -> (number=w2519:dbl)  [unwired: 3 in, 1 out]
                      n1246 = Fract/Exp String To Number(string=w2534) -> (number=w2533:dbl)  [unwired: 3 in, 1 out]
                      n1247 = Fract/Exp String To Number(string=w2531) -> (number=w2528:dbl)  [unwired: 3 in, 1 out]
                      n1248 = Divide(x=w2533, y=100.0) -> (x/y=w2520:dbl)
                      n1249 = Multiply(x=w2520, y=w2519) -> (x*y=w2518:dbl)
                      n1250 = Add(x=w2519, y=w2518) -> (x+y=w2530:dbl)
                      n1251 = Subtract(x=w2519, y=w2518) -> (x-y=w2529:dbl)
                      n1252 = In Range and Coerce(upper limit=w2530, x=w2528, lower limit=w2529) -> (In Range?=w2527:bool)  [unwired: 1 out]
                      n1253 = Select(t="P", s=w2527, f="F") -> (s? t:f=w2522:string)
                      n1254 = Replace Array Subset(array=w2538, new element #1=w2531, index (row) #1=w2524, index (col) #1=w2539, new element #2=w2522, index (row) #2=w2524, index (col) #2=5 ("disabled index (col)")) -> (w2521:string[][])
                    }
                    frame 1 {
                      w2558 = 3  # tol
                      w2559 = 2  # res
                      w2561 = 4  # meas
                      # "fill the P/F\ncol"
                      # "fill the meas col"
                      # "check to see\npass or fail"
                      # "pull out resistor\nvalue and tolerance\nto find limits"
                      n1255 = Index Array(array=w2560, index (row) #1=w2546, index (col) #1=w2559, index (row) #2=w2546, index (col) #2=w2558) -> (element #1=w2557:string, element #2=w2556:string)
                      n1256 = Fract/Exp String To Number(string=w2557) -> (number=w2541:dbl)  [unwired: 3 in, 1 out]
                      n1257 = Fract/Exp String To Number(string=w2556) -> (number=w2555:dbl)  [unwired: 3 in, 1 out]
                      n1258 = Fract/Exp String To Number(string=w2553) -> (number=w2550:dbl)  [unwired: 3 in, 1 out]
                      n1259 = Divide(x=w2555, y=100.0) -> (x/y=w2542:dbl)
                      n1260 = Multiply(x=w2542, y=w2541) -> (x*y=w2540:dbl)
                      n1261 = Add(x=w2541, y=w2540) -> (x+y=w2552:dbl)
                      n1262 = Subtract(x=w2541, y=w2540) -> (x-y=w2551:dbl)
                      n1263 = In Range and Coerce(upper limit=w2552, x=w2550, lower limit=w2551) -> (In Range?=w2549:bool)  [unwired: 1 out]
                      n1264 = Select(t="P", s=w2549, f="F") -> (s? t:f=w2544:string)
                      n1265 = Replace Array Subset(array=w2560, new element #1=w2553, index (row) #1=w2546, index (col) #1=w2561, new element #2=w2544, index (row) #2=w2546, index (col) #2=5 ("disabled index (col)")) -> (w2543:string[][])
                    }
                    frame 2 {
                      w2580 = 3  # tol
                      w2581 = 2  # res
                      w2583 = 4  # meas
                      # "fill the P/F\ncol"
                      # "fill the meas col"
                      # "check to see\npass or fail"
                      # "pull out resistor\nvalue and tolerance\nto find limits"
                      n1266 = Index Array(array=w2582, index (row) #1=w2568, index (col) #1=w2581, index (row) #2=w2568, index (col) #2=w2580) -> (element #1=w2579:string, element #2=w2578:string)
                      n1267 = Fract/Exp String To Number(string=w2579) -> (number=w2563:dbl)  [unwired: 3 in, 1 out]
                      n1268 = Fract/Exp String To Number(string=w2578) -> (number=w2577:dbl)  [unwired: 3 in, 1 out]
                      n1269 = Fract/Exp String To Number(string=w2575) -> (number=w2572:dbl)  [unwired: 3 in, 1 out]
                      n1270 = Divide(x=w2577, y=100.0) -> (x/y=w2564:dbl)
                      n1271 = Multiply(x=w2564, y=w2563) -> (x*y=w2562:dbl)
                      n1272 = Add(x=w2563, y=w2562) -> (x+y=w2574:dbl)
                      n1273 = Subtract(x=w2563, y=w2562) -> (x-y=w2573:dbl)
                      n1274 = In Range and Coerce(upper limit=w2574, x=w2572, lower limit=w2573) -> (In Range?=w2571:bool)  [unwired: 1 out]
                      n1275 = Select(t="P", s=w2571, f="F") -> (s? t:f=w2566:string)
                      n1276 = Replace Array Subset(array=w2582, new element #1=w2575, index (row) #1=w2568, index (col) #1=w2583, new element #2=w2566, index (row) #2=w2568, index (col) #2=5 ("disabled index (col)")) -> (w2565:string[][])
                    }
                    frame 3 {
                      w2602 = 3  # tol
                      w2603 = 2  # res
                      w2605 = 4  # meas
                      # "fill the P/F\ncol"
                      # "fill the meas col"
                      # "check to see\npass or fail"
                      # "pull out resistor\nvalue and tolerance\nto find limits"
                      n1277 = Index Array(array=w2604, index (row) #1=w2590, index (col) #1=w2603, index (row) #2=w2590, index (col) #2=w2602) -> (element #1=w2601:string, element #2=w2600:string)
                      n1278 = Fract/Exp String To Number(string=w2601) -> (number=w2585:dbl)  [unwired: 3 in, 1 out]
                      n1279 = Fract/Exp String To Number(string=w2600) -> (number=w2599:dbl)  [unwired: 3 in, 1 out]
                      n1280 = Fract/Exp String To Number(string=w2597) -> (number=w2594:dbl)  [unwired: 3 in, 1 out]
                      n1281 = Divide(x=w2599, y=100.0) -> (x/y=w2586:dbl)
                      n1282 = Multiply(x=w2586, y=w2585) -> (x*y=w2584:dbl)
                      n1283 = Add(x=w2585, y=w2584) -> (x+y=w2596:dbl)
                      n1284 = Subtract(x=w2585, y=w2584) -> (x-y=w2595:dbl)
                      n1285 = In Range and Coerce(upper limit=w2596, x=w2594, lower limit=w2595) -> (In Range?=w2593:bool)  [unwired: 1 out]
                      n1286 = Select(t="P", s=w2593, f="F") -> (s? t:f=w2588:string)
                      n1287 = Replace Array Subset(array=w2604, new element #1=w2597, index (row) #1=w2590, index (col) #1=w2605, new element #2=w2588, index (row) #2=w2590, index (col) #2=5 ("disabled index (col)")) -> (w2587:string[][])
                    }
                    frame 4 {
                      w2624 = 3  # tol
                      w2625 = 2  # res
                      w2627 = 4  # meas
                      # "fill the P/F\ncol"
                      # "fill the meas col"
                      # "check to see\npass or fail"
                      # "pull out resistor\nvalue and tolerance\nto find limits"
                      n1288 = Index Array(array=w2626, index (row) #1=w2612, index (col) #1=w2625, index (row) #2=w2612, index (col) #2=w2624) -> (element #1=w2623:string, element #2=w2622:string)
                      n1289 = Fract/Exp String To Number(string=w2623) -> (number=w2607:dbl)  [unwired: 3 in, 1 out]
                      n1290 = Fract/Exp String To Number(string=w2622) -> (number=w2621:dbl)  [unwired: 3 in, 1 out]
                      n1291 = Fract/Exp String To Number(string=w2619) -> (number=w2616:dbl)  [unwired: 3 in, 1 out]
                      n1292 = Divide(x=w2621, y=100.0) -> (x/y=w2608:dbl)
                      n1293 = Multiply(x=w2608, y=w2607) -> (x*y=w2606:dbl)
                      n1294 = Add(x=w2607, y=w2606) -> (x+y=w2618:dbl)
                      n1295 = Subtract(x=w2607, y=w2606) -> (x-y=w2617:dbl)
                      n1296 = In Range and Coerce(upper limit=w2618, x=w2616, lower limit=w2617) -> (In Range?=w2615:bool)  [unwired: 1 out]
                      n1297 = Select(t="P", s=w2615, f="F") -> (s? t:f=w2610:string)
                      n1298 = Replace Array Subset(array=w2626, new element #1=w2619, index (row) #1=w2612, index (col) #1=w2627, new element #2=w2610, index (row) #2=w2612, index (col) #2=5 ("disabled index (col)")) -> (w2609:string[][])
                    }
                    frame 5 {
                      w2646 = 3  # tol
                      w2647 = 2  # res
                      w2649 = 4  # meas
                      # "fill the P/F\ncol"
                      # "fill the meas col"
                      # "check to see\npass or fail"
                      # "pull out resistor\nvalue and tolerance\nto find limits"
                      n1299 = Index Array(array=w2648, index (row) #1=w2634, index (col) #1=w2647, index (row) #2=w2634, index (col) #2=w2646) -> (element #1=w2645:string, element #2=w2644:string)
                      n1300 = Fract/Exp String To Number(string=w2645) -> (number=w2629:dbl)  [unwired: 3 in, 1 out]
                      n1301 = Fract/Exp String To Number(string=w2644) -> (number=w2643:dbl)  [unwired: 3 in, 1 out]
                      n1302 = Fract/Exp String To Number(string=w2641) -> (number=w2638:dbl)  [unwired: 3 in, 1 out]
                      n1303 = Divide(x=w2643, y=100.0) -> (x/y=w2630:dbl)
                      n1304 = Multiply(x=w2630, y=w2629) -> (x*y=w2628:dbl)
                      n1305 = Add(x=w2629, y=w2628) -> (x+y=w2640:dbl)
                      n1306 = Subtract(x=w2629, y=w2628) -> (x-y=w2639:dbl)
                      n1307 = In Range and Coerce(upper limit=w2640, x=w2638, lower limit=w2639) -> (In Range?=w2637:bool)  [unwired: 1 out]
                      n1308 = Select(t="P", s=w2637, f="F") -> (s? t:f=w2632:string)
                      n1309 = Replace Array Subset(array=w2648, new element #1=w2641, index (row) #1=w2634, index (col) #1=w2649, new element #2=w2632, index (row) #2=w2634, index (col) #2=5 ("disabled index (col)")) -> (w2631:string[][])
                    }
                    frame 6 {
                      w2668 = 3  # tol
                      w2669 = 2  # res
                      w2671 = 4  # meas
                      # "fill the P/F\ncol"
                      # "fill the meas col"
                      # "check to see\npass or fail"
                      # "pull out resistor\nvalue and tolerance\nto find limits"
                      n1310 = Index Array(array=w2670, index (row) #1=w2656, index (col) #1=w2669, index (row) #2=w2656, index (col) #2=w2668) -> (element #1=w2667:string, element #2=w2666:string)
                      n1311 = Fract/Exp String To Number(string=w2667) -> (number=w2651:dbl)  [unwired: 3 in, 1 out]
                      n1312 = Fract/Exp String To Number(string=w2666) -> (number=w2665:dbl)  [unwired: 3 in, 1 out]
                      n1313 = Fract/Exp String To Number(string=w2663) -> (number=w2660:dbl)  [unwired: 3 in, 1 out]
                      n1314 = Divide(x=w2665, y=100.0) -> (x/y=w2652:dbl)
                      n1315 = Multiply(x=w2652, y=w2651) -> (x*y=w2650:dbl)
                      n1316 = Add(x=w2651, y=w2650) -> (x+y=w2662:dbl)
                      n1317 = Subtract(x=w2651, y=w2650) -> (x-y=w2661:dbl)
                      n1318 = In Range and Coerce(upper limit=w2662, x=w2660, lower limit=w2661) -> (In Range?=w2659:bool)  [unwired: 1 out]
                      n1319 = Select(t="P", s=w2659, f="F") -> (s? t:f=w2654:string)
                      n1320 = Replace Array Subset(array=w2670, new element #1=w2663, index (row) #1=w2656, index (col) #1=w2671, new element #2=w2654, index (row) #2=w2656, index (col) #2=5 ("disabled index (col)")) -> (w2653:string[][])
                    }
                    frame 7 {
                      w2690 = 3  # tol
                      w2691 = 2  # res
                      w2693 = 4  # meas
                      # "fill the P/F\ncol"
                      # "fill the meas col"
                      # "check to see\npass or fail"
                      # "pull out resistor\nvalue and tolerance\nto find limits"
                      n1321 = Index Array(array=w2692, index (row) #1=w2678, index (col) #1=w2691, index (row) #2=w2678, index (col) #2=w2690) -> (element #1=w2689:string, element #2=w2688:string)
                      n1322 = Fract/Exp String To Number(string=w2689) -> (number=w2673:dbl)  [unwired: 3 in, 1 out]
                      n1323 = Fract/Exp String To Number(string=w2688) -> (number=w2687:dbl)  [unwired: 3 in, 1 out]
                      n1324 = Fract/Exp String To Number(string=w2685) -> (number=w2682:dbl)  [unwired: 3 in, 1 out]
                      n1325 = Divide(x=w2687, y=100.0) -> (x/y=w2674:dbl)
                      n1326 = Multiply(x=w2674, y=w2673) -> (x*y=w2672:dbl)
                      n1327 = Add(x=w2673, y=w2672) -> (x+y=w2684:dbl)
                      n1328 = Subtract(x=w2673, y=w2672) -> (x-y=w2683:dbl)
                      n1329 = In Range and Coerce(upper limit=w2684, x=w2682, lower limit=w2683) -> (In Range?=w2681:bool)  [unwired: 1 out]
                      n1330 = Select(t="P", s=w2681, f="F") -> (s? t:f=w2676:string)
                      n1331 = Replace Array Subset(array=w2692, new element #1=w2685, index (row) #1=w2678, index (col) #1=w2693, new element #2=w2676, index (row) #2=w2678, index (col) #2=5 ("disabled index (col)")) -> (w2675:string[][])
                    }
                    frame 8 {
                      w2712 = 3  # tol
                      w2713 = 2  # res
                      w2715 = 4  # meas
                      # "fill the P/F\ncol"
                      # "fill the meas col"
                      # "check to see\npass or fail"
                      # "pull out resistor\nvalue and tolerance\nto find limits"
                      n1332 = Index Array(array=w2714, index (row) #1=w2700, index (col) #1=w2713, index (row) #2=w2700, index (col) #2=w2712) -> (element #1=w2711:string, element #2=w2710:string)
                      n1333 = Fract/Exp String To Number(string=w2711) -> (number=w2695:dbl)  [unwired: 3 in, 1 out]
                      n1334 = Fract/Exp String To Number(string=w2710) -> (number=w2709:dbl)  [unwired: 3 in, 1 out]
                      n1335 = Fract/Exp String To Number(string=w2707) -> (number=w2704:dbl)  [unwired: 3 in, 1 out]
                      n1336 = Divide(x=w2709, y=100.0) -> (x/y=w2696:dbl)
                      n1337 = Multiply(x=w2696, y=w2695) -> (x*y=w2694:dbl)
                      n1338 = Add(x=w2695, y=w2694) -> (x+y=w2706:dbl)
                      n1339 = Subtract(x=w2695, y=w2694) -> (x-y=w2705:dbl)
                      n1340 = In Range and Coerce(upper limit=w2706, x=w2704, lower limit=w2705) -> (In Range?=w2703:bool)  [unwired: 1 out]
                      n1341 = Select(t="P", s=w2703, f="F") -> (s? t:f=w2698:string)
                      n1342 = Replace Array Subset(array=w2714, new element #1=w2707, index (row) #1=w2700, index (col) #1=w2715, new element #2=w2698, index (row) #2=w2700, index (col) #2=5 ("disabled index (col)")) -> (w2697:string[][])
                    }
                    frame 9 {
                      w2734 = 3  # tol
                      w2735 = 2  # res
                      w2737 = 4  # meas
                      # "fill the P/F\ncol"
                      # "fill the meas col"
                      # "check to see\npass or fail"
                      # "pull out resistor\nvalue and tolerance\nto find limits"
                      n1343 = Index Array(array=w2736, index (row) #1=w2722, index (col) #1=w2735, index (row) #2=w2722, index (col) #2=w2734) -> (element #1=w2733:string, element #2=w2732:string)
                      n1344 = Fract/Exp String To Number(string=w2733) -> (number=w2717:dbl)  [unwired: 3 in, 1 out]
                      n1345 = Fract/Exp String To Number(string=w2732) -> (number=w2731:dbl)  [unwired: 3 in, 1 out]
                      n1346 = Fract/Exp String To Number(string=w2729) -> (number=w2726:dbl)  [unwired: 3 in, 1 out]
                      n1347 = Divide(x=w2731, y=100.0) -> (x/y=w2718:dbl)
                      n1348 = Multiply(x=w2718, y=w2717) -> (x*y=w2716:dbl)
                      n1349 = Add(x=w2717, y=w2716) -> (x+y=w2728:dbl)
                      n1350 = Subtract(x=w2717, y=w2716) -> (x-y=w2727:dbl)
                      n1351 = In Range and Coerce(upper limit=w2728, x=w2726, lower limit=w2727) -> (In Range?=w2725:bool)  [unwired: 1 out]
                      n1352 = Select(t="P", s=w2725, f="F") -> (s? t:f=w2720:string)
                      n1353 = Replace Array Subset(array=w2736, new element #1=w2729, index (row) #1=w2722, index (col) #1=w2737, new element #2=w2720, index (row) #2=w2722, index (col) #2=5 ("disabled index (col)")) -> (w2719:string[][])
                    }
                    frame 10 {
                      w2756 = 3  # tol
                      w2757 = 2  # res
                      w2759 = 4  # meas
                      # "fill the P/F\ncol"
                      # "fill the meas col"
                      # "check to see\npass or fail"
                      # "pull out resistor\nvalue and tolerance\nto find limits"
                      n1354 = Index Array(array=w2758, index (row) #1=w2744, index (col) #1=w2757, index (row) #2=w2744, index (col) #2=w2756) -> (element #1=w2755:string, element #2=w2754:string)
                      n1355 = Fract/Exp String To Number(string=w2755) -> (number=w2739:dbl)  [unwired: 3 in, 1 out]
                      n1356 = Fract/Exp String To Number(string=w2754) -> (number=w2753:dbl)  [unwired: 3 in, 1 out]
                      n1357 = Fract/Exp String To Number(string=w2751) -> (number=w2748:dbl)  [unwired: 3 in, 1 out]
                      n1358 = Divide(x=w2753, y=100.0) -> (x/y=w2740:dbl)
                      n1359 = Multiply(x=w2740, y=w2739) -> (x*y=w2738:dbl)
                      n1360 = Add(x=w2739, y=w2738) -> (x+y=w2750:dbl)
                      n1361 = Subtract(x=w2739, y=w2738) -> (x-y=w2749:dbl)
                      n1362 = In Range and Coerce(upper limit=w2750, x=w2748, lower limit=w2749) -> (In Range?=w2747:bool)  [unwired: 1 out]
                      n1363 = Select(t="P", s=w2747, f="F") -> (s? t:f=w2742:string)
                      n1364 = Replace Array Subset(array=w2758, new element #1=w2751, index (row) #1=w2744, index (col) #1=w2759, new element #2=w2742, index (row) #2=w2744, index (col) #2=5 ("disabled index (col)")) -> (w2741:string[][])
                    }
                    frame 11 {
                      w2778 = 3  # tol
                      w2779 = 2  # res
                      w2781 = 4  # meas
                      # "fill the P/F\ncol"
                      # "fill the meas col"
                      # "check to see\npass or fail"
                      # "pull out resistor\nvalue and tolerance\nto find limits"
                      n1365 = Index Array(array=w2780, index (row) #1=w2766, index (col) #1=w2779, index (row) #2=w2766, index (col) #2=w2778) -> (element #1=w2777:string, element #2=w2776:string)
                      n1366 = Fract/Exp String To Number(string=w2777) -> (number=w2761:dbl)  [unwired: 3 in, 1 out]
                      n1367 = Fract/Exp String To Number(string=w2776) -> (number=w2775:dbl)  [unwired: 3 in, 1 out]
                      n1368 = Fract/Exp String To Number(string=w2773) -> (number=w2770:dbl)  [unwired: 3 in, 1 out]
                      n1369 = Divide(x=w2775, y=100.0) -> (x/y=w2762:dbl)
                      n1370 = Multiply(x=w2762, y=w2761) -> (x*y=w2760:dbl)
                      n1371 = Add(x=w2761, y=w2760) -> (x+y=w2772:dbl)
                      n1372 = Subtract(x=w2761, y=w2760) -> (x-y=w2771:dbl)
                      n1373 = In Range and Coerce(upper limit=w2772, x=w2770, lower limit=w2771) -> (In Range?=w2769:bool)  [unwired: 1 out]
                      n1374 = Select(t="P", s=w2769, f="F") -> (s? t:f=w2764:string)
                      n1375 = Replace Array Subset(array=w2780, new element #1=w2773, index (row) #1=w2766, index (col) #1=w2781, new element #2=w2764, index (row) #2=w2766, index (col) #2=5 ("disabled index (col)")) -> (w2763:string[][])
                    }
                    frame 12 {
                      w2800 = 3  # tol
                      w2801 = 2  # res
                      w2803 = 4  # meas
                      # "fill the P/F\ncol"
                      # "fill the meas col"
                      # "check to see\npass or fail"
                      # "pull out resistor\nvalue and tolerance\nto find limits"
                      n1376 = Index Array(array=w2802, index (row) #1=w2788, index (col) #1=w2801, index (row) #2=w2788, index (col) #2=w2800) -> (element #1=w2799:string, element #2=w2798:string)
                      n1377 = Fract/Exp String To Number(string=w2799) -> (number=w2783:dbl)  [unwired: 3 in, 1 out]
                      n1378 = Fract/Exp String To Number(string=w2798) -> (number=w2797:dbl)  [unwired: 3 in, 1 out]
                      n1379 = Fract/Exp String To Number(string=w2795) -> (number=w2792:dbl)  [unwired: 3 in, 1 out]
                      n1380 = Divide(x=w2797, y=100.0) -> (x/y=w2784:dbl)
                      n1381 = Multiply(x=w2784, y=w2783) -> (x*y=w2782:dbl)
                      n1382 = Add(x=w2783, y=w2782) -> (x+y=w2794:dbl)
                      n1383 = Subtract(x=w2783, y=w2782) -> (x-y=w2793:dbl)
                      n1384 = In Range and Coerce(upper limit=w2794, x=w2792, lower limit=w2793) -> (In Range?=w2791:bool)  [unwired: 1 out]
                      n1385 = Select(t="P", s=w2791, f="F") -> (s? t:f=w2786:string)
                      n1386 = Replace Array Subset(array=w2802, new element #1=w2795, index (row) #1=w2788, index (col) #1=w2803, new element #2=w2786, index (row) #2=w2788, index (col) #2=5 ("disabled index (col)")) -> (w2785:string[][])
                    }
                    frame 13 {
                      w2822 = 3  # tol
                      w2823 = 2  # res
                      w2825 = 4  # meas
                      # "fill the P/F\ncol"
                      # "fill the meas col"
                      # "check to see\npass or fail"
                      # "pull out resistor\nvalue and tolerance\nto find limits"
                      n1387 = Index Array(array=w2824, index (row) #1=w2810, index (col) #1=w2823, index (row) #2=w2810, index (col) #2=w2822) -> (element #1=w2821:string, element #2=w2820:string)
                      n1388 = Fract/Exp String To Number(string=w2821) -> (number=w2805:dbl)  [unwired: 3 in, 1 out]
                      n1389 = Fract/Exp String To Number(string=w2820) -> (number=w2819:dbl)  [unwired: 3 in, 1 out]
                      n1390 = Fract/Exp String To Number(string=w2817) -> (number=w2814:dbl)  [unwired: 3 in, 1 out]
                      n1391 = Divide(x=w2819, y=100.0) -> (x/y=w2806:dbl)
                      n1392 = Multiply(x=w2806, y=w2805) -> (x*y=w2804:dbl)
                      n1393 = Add(x=w2805, y=w2804) -> (x+y=w2816:dbl)
                      n1394 = Subtract(x=w2805, y=w2804) -> (x-y=w2815:dbl)
                      n1395 = In Range and Coerce(upper limit=w2816, x=w2814, lower limit=w2815) -> (In Range?=w2813:bool)  [unwired: 1 out]
                      n1396 = Select(t="P", s=w2813, f="F") -> (s? t:f=w2808:string)
                      n1397 = Replace Array Subset(array=w2824, new element #1=w2817, index (row) #1=w2810, index (col) #1=w2825, new element #2=w2808, index (row) #2=w2810, index (col) #2=5 ("disabled index (col)")) -> (w2807:string[][])
                    }
                    frame 14 {
                      w2844 = 3  # tol
                      w2845 = 2  # res
                      w2847 = 4  # meas
                      # "fill the P/F\ncol"
                      # "fill the meas col"
                      # "check to see\npass or fail"
                      # "pull out resistor\nvalue and tolerance\nto find limits"
                      n1398 = Index Array(array=w2846, index (row) #1=w2832, index (col) #1=w2845, index (row) #2=w2832, index (col) #2=w2844) -> (element #1=w2843:string, element #2=w2842:string)
                      n1399 = Fract/Exp String To Number(string=w2843) -> (number=w2827:dbl)  [unwired: 3 in, 1 out]
                      n1400 = Fract/Exp String To Number(string=w2842) -> (number=w2841:dbl)  [unwired: 3 in, 1 out]
                      n1401 = Fract/Exp String To Number(string=w2839) -> (number=w2836:dbl)  [unwired: 3 in, 1 out]
                      n1402 = Divide(x=w2841, y=100.0) -> (x/y=w2828:dbl)
                      n1403 = Multiply(x=w2828, y=w2827) -> (x*y=w2826:dbl)
                      n1404 = Add(x=w2827, y=w2826) -> (x+y=w2838:dbl)
                      n1405 = Subtract(x=w2827, y=w2826) -> (x-y=w2837:dbl)
                      n1406 = In Range and Coerce(upper limit=w2838, x=w2836, lower limit=w2837) -> (In Range?=w2835:bool)  [unwired: 1 out]
                      n1407 = Select(t="P", s=w2835, f="F") -> (s? t:f=w2830:string)
                      n1408 = Replace Array Subset(array=w2846, new element #1=w2839, index (row) #1=w2832, index (col) #1=w2847, new element #2=w2830, index (row) #2=w2832, index (col) #2=5 ("disabled index (col)")) -> (w2829:string[][])
                    }
                    frame 15 {
                      w2866 = 3  # tol
                      w2867 = 2  # res
                      w2869 = 4  # meas
                      # "fill the P/F\ncol"
                      # "fill the meas col"
                      # "check to see\npass or fail"
                      # "pull out resistor\nvalue and tolerance\nto find limits"
                      n1409 = Index Array(array=w2868, index (row) #1=w2854, index (col) #1=w2867, index (row) #2=w2854, index (col) #2=w2866) -> (element #1=w2865:string, element #2=w2864:string)
                      n1410 = Fract/Exp String To Number(string=w2865) -> (number=w2849:dbl)  [unwired: 3 in, 1 out]
                      n1411 = Fract/Exp String To Number(string=w2864) -> (number=w2863:dbl)  [unwired: 3 in, 1 out]
                      n1412 = Fract/Exp String To Number(string=w2861) -> (number=w2858:dbl)  [unwired: 3 in, 1 out]
                      n1413 = Divide(x=w2863, y=100.0) -> (x/y=w2850:dbl)
                      n1414 = Multiply(x=w2850, y=w2849) -> (x*y=w2848:dbl)
                      n1415 = Add(x=w2849, y=w2848) -> (x+y=w2860:dbl)
                      n1416 = Subtract(x=w2849, y=w2848) -> (x-y=w2859:dbl)
                      n1417 = In Range and Coerce(upper limit=w2860, x=w2858, lower limit=w2859) -> (In Range?=w2857:bool)  [unwired: 1 out]
                      n1418 = Select(t="P", s=w2857, f="F") -> (s? t:f=w2852:string)
                      n1419 = Replace Array Subset(array=w2868, new element #1=w2861, index (row) #1=w2854, index (col) #1=w2869, new element #2=w2852, index (row) #2=w2854, index (col) #2=5 ("disabled index (col)")) -> (w2851:string[][])
                    }
                    frame 16 {
                      w2888 = 3  # tol
                      w2889 = 2  # res
                      w2891 = 4  # meas
                      # "fill the P/F\ncol"
                      # "fill the meas col"
                      # "check to see\npass or fail"
                      # "pull out resistor\nvalue and tolerance\nto find limits"
                      n1420 = Index Array(array=w2890, index (row) #1=w2876, index (col) #1=w2889, index (row) #2=w2876, index (col) #2=w2888) -> (element #1=w2887:string, element #2=w2886:string)
                      n1421 = Fract/Exp String To Number(string=w2887) -> (number=w2871:dbl)  [unwired: 3 in, 1 out]
                      n1422 = Fract/Exp String To Number(string=w2886) -> (number=w2885:dbl)  [unwired: 3 in, 1 out]
                      n1423 = Fract/Exp String To Number(string=w2883) -> (number=w2880:dbl)  [unwired: 3 in, 1 out]
                      n1424 = Divide(x=w2885, y=100.0) -> (x/y=w2872:dbl)
                      n1425 = Multiply(x=w2872, y=w2871) -> (x*y=w2870:dbl)
                      n1426 = Add(x=w2871, y=w2870) -> (x+y=w2882:dbl)
                      n1427 = Subtract(x=w2871, y=w2870) -> (x-y=w2881:dbl)
                      n1428 = In Range and Coerce(upper limit=w2882, x=w2880, lower limit=w2881) -> (In Range?=w2879:bool)  [unwired: 1 out]
                      n1429 = Select(t="P", s=w2879, f="F") -> (s? t:f=w2874:string)
                      n1430 = Replace Array Subset(array=w2890, new element #1=w2883, index (row) #1=w2876, index (col) #1=w2891, new element #2=w2874, index (row) #2=w2876, index (col) #2=5 ("disabled index (col)")) -> (w2873:string[][])
                    }
                    frame 17 {
                      w2910 = 3  # tol
                      w2911 = 2  # res
                      w2913 = 4  # meas
                      # "fill the P/F\ncol"
                      # "fill the meas col"
                      # "check to see\npass or fail"
                      # "pull out resistor\nvalue and tolerance\nto find limits"
                      n1431 = Index Array(array=w2912, index (row) #1=w2898, index (col) #1=w2911, index (row) #2=w2898, index (col) #2=w2910) -> (element #1=w2909:string, element #2=w2908:string)
                      n1432 = Fract/Exp String To Number(string=w2909) -> (number=w2893:dbl)  [unwired: 3 in, 1 out]
                      n1433 = Fract/Exp String To Number(string=w2908) -> (number=w2907:dbl)  [unwired: 3 in, 1 out]
                      n1434 = Fract/Exp String To Number(string=w2905) -> (number=w2902:dbl)  [unwired: 3 in, 1 out]
                      n1435 = Divide(x=w2907, y=100.0) -> (x/y=w2894:dbl)
                      n1436 = Multiply(x=w2894, y=w2893) -> (x*y=w2892:dbl)
                      n1437 = Add(x=w2893, y=w2892) -> (x+y=w2904:dbl)
                      n1438 = Subtract(x=w2893, y=w2892) -> (x-y=w2903:dbl)
                      n1439 = In Range and Coerce(upper limit=w2904, x=w2902, lower limit=w2903) -> (In Range?=w2901:bool)  [unwired: 1 out]
                      n1440 = Select(t="P", s=w2901, f="F") -> (s? t:f=w2896:string)
                      n1441 = Replace Array Subset(array=w2912, new element #1=w2905, index (row) #1=w2898, index (col) #1=w2913, new element #2=w2896, index (row) #2=w2898, index (col) #2=5 ("disabled index (col)")) -> (w2895:string[][])
                    }
                    frame 18 {
                      w2932 = 3  # tol
                      w2933 = 2  # res
                      w2935 = 4  # meas
                      # "fill the P/F\ncol"
                      # "fill the meas col"
                      # "check to see\npass or fail"
                      # "pull out resistor\nvalue and tolerance\nto find limits"
                      n1442 = Index Array(array=w2934, index (row) #1=w2920, index (col) #1=w2933, index (row) #2=w2920, index (col) #2=w2932) -> (element #1=w2931:string, element #2=w2930:string)
                      n1443 = Fract/Exp String To Number(string=w2931) -> (number=w2915:dbl)  [unwired: 3 in, 1 out]
                      n1444 = Fract/Exp String To Number(string=w2930) -> (number=w2929:dbl)  [unwired: 3 in, 1 out]
                      n1445 = Fract/Exp String To Number(string=w2927) -> (number=w2924:dbl)  [unwired: 3 in, 1 out]
                      n1446 = Divide(x=w2929, y=100.0) -> (x/y=w2916:dbl)
                      n1447 = Multiply(x=w2916, y=w2915) -> (x*y=w2914:dbl)
                      n1448 = Add(x=w2915, y=w2914) -> (x+y=w2926:dbl)
                      n1449 = Subtract(x=w2915, y=w2914) -> (x-y=w2925:dbl)
                      n1450 = In Range and Coerce(upper limit=w2926, x=w2924, lower limit=w2925) -> (In Range?=w2923:bool)  [unwired: 1 out]
                      n1451 = Select(t="P", s=w2923, f="F") -> (s? t:f=w2918:string)
                      n1452 = Replace Array Subset(array=w2934, new element #1=w2927, index (row) #1=w2920, index (col) #1=w2935, new element #2=w2918, index (row) #2=w2920, index (col) #2=5 ("disabled index (col)")) -> (w2917:string[][])
                    }
                    frame 19 {
                      w2954 = 3  # tol
                      w2955 = 2  # res
                      w2957 = 4  # meas
                      # "fill the P/F\ncol"
                      # "fill the meas col"
                      # "check to see\npass or fail"
                      # "pull out resistor\nvalue and tolerance\nto find limits"
                      n1453 = Index Array(array=w2956, index (row) #1=w2942, index (col) #1=w2955, index (row) #2=w2942, index (col) #2=w2954) -> (element #1=w2953:string, element #2=w2952:string)
                      n1454 = Fract/Exp String To Number(string=w2953) -> (number=w2937:dbl)  [unwired: 3 in, 1 out]
                      n1455 = Fract/Exp String To Number(string=w2952) -> (number=w2951:dbl)  [unwired: 3 in, 1 out]
                      n1456 = Fract/Exp String To Number(string=w2949) -> (number=w2946:dbl)  [unwired: 3 in, 1 out]
                      n1457 = Divide(x=w2951, y=100.0) -> (x/y=w2938:dbl)
                      n1458 = Multiply(x=w2938, y=w2937) -> (x*y=w2936:dbl)
                      n1459 = Add(x=w2937, y=w2936) -> (x+y=w2948:dbl)
                      n1460 = Subtract(x=w2937, y=w2936) -> (x-y=w2947:dbl)
                      n1461 = In Range and Coerce(upper limit=w2948, x=w2946, lower limit=w2947) -> (In Range?=w2945:bool)  [unwired: 1 out]
                      n1462 = Select(t="P", s=w2945, f="F") -> (s? t:f=w2940:string)
                      n1463 = Replace Array Subset(array=w2956, new element #1=w2949, index (row) #1=w2942, index (col) #1=w2957, new element #2=w2940, index (row) #2=w2942, index (col) #2=5 ("disabled index (col)")) -> (w2939:string[][])
                    }
                    frame 20 {
                      w2976 = 3  # tol
                      w2977 = 2  # res
                      w2979 = 4  # meas
                      # "fill the P/F\ncol"
                      # "fill the meas col"
                      # "check to see\npass or fail"
                      # "pull out resistor\nvalue and tolerance\nto find limits"
                      n1464 = Index Array(array=w2978, index (row) #1=w2964, index (col) #1=w2977, index (row) #2=w2964, index (col) #2=w2976) -> (element #1=w2975:string, element #2=w2974:string)
                      n1465 = Fract/Exp String To Number(string=w2975) -> (number=w2959:dbl)  [unwired: 3 in, 1 out]
                      n1466 = Fract/Exp String To Number(string=w2974) -> (number=w2973:dbl)  [unwired: 3 in, 1 out]
                      n1467 = Fract/Exp String To Number(string=w2971) -> (number=w2968:dbl)  [unwired: 3 in, 1 out]
                      n1468 = Divide(x=w2973, y=100.0) -> (x/y=w2960:dbl)
                      n1469 = Multiply(x=w2960, y=w2959) -> (x*y=w2958:dbl)
                      n1470 = Add(x=w2959, y=w2958) -> (x+y=w2970:dbl)
                      n1471 = Subtract(x=w2959, y=w2958) -> (x-y=w2969:dbl)
                      n1472 = In Range and Coerce(upper limit=w2970, x=w2968, lower limit=w2969) -> (In Range?=w2967:bool)  [unwired: 1 out]
                      n1473 = Select(t="P", s=w2967, f="F") -> (s? t:f=w2962:string)
                      n1474 = Replace Array Subset(array=w2978, new element #1=w2971, index (row) #1=w2964, index (col) #1=w2979, new element #2=w2962, index (row) #2=w2964, index (col) #2=5 ("disabled index (col)")) -> (w2961:string[][])
                    }
                    frame 21 {
                      w2998 = 3  # tol
                      w2999 = 2  # res
                      w3001 = 4  # meas
                      # "fill the P/F\ncol"
                      # "fill the meas col"
                      # "check to see\npass or fail"
                      # "pull out resistor\nvalue and tolerance\nto find limits"
                      n1475 = Index Array(array=w3000, index (row) #1=w2986, index (col) #1=w2999, index (row) #2=w2986, index (col) #2=w2998) -> (element #1=w2997:string, element #2=w2996:string)
                      n1476 = Fract/Exp String To Number(string=w2997) -> (number=w2981:dbl)  [unwired: 3 in, 1 out]
                      n1477 = Fract/Exp String To Number(string=w2996) -> (number=w2995:dbl)  [unwired: 3 in, 1 out]
                      n1478 = Fract/Exp String To Number(string=w2993) -> (number=w2990:dbl)  [unwired: 3 in, 1 out]
                      n1479 = Divide(x=w2995, y=100.0) -> (x/y=w2982:dbl)
                      n1480 = Multiply(x=w2982, y=w2981) -> (x*y=w2980:dbl)
                      n1481 = Add(x=w2981, y=w2980) -> (x+y=w2992:dbl)
                      n1482 = Subtract(x=w2981, y=w2980) -> (x-y=w2991:dbl)
                      n1483 = In Range and Coerce(upper limit=w2992, x=w2990, lower limit=w2991) -> (In Range?=w2989:bool)  [unwired: 1 out]
                      n1484 = Select(t="P", s=w2989, f="F") -> (s? t:f=w2984:string)
                      n1485 = Replace Array Subset(array=w3000, new element #1=w2993, index (row) #1=w2986, index (col) #1=w3001, new element #2=w2984, index (row) #2=w2986, index (col) #2=5 ("disabled index (col)")) -> (w2983:string[][])
                    }
                    frame 22 {
                      w3020 = 3  # tol
                      w3021 = 2  # res
                      w3023 = 4  # meas
                      # "fill the P/F\ncol"
                      # "fill the meas col"
                      # "check to see\npass or fail"
                      # "pull out resistor\nvalue and tolerance\nto find limits"
                      n1486 = Index Array(array=w3022, index (row) #1=w3008, index (col) #1=w3021, index (row) #2=w3008, index (col) #2=w3020) -> (element #1=w3019:string, element #2=w3018:string)
                      n1487 = Fract/Exp String To Number(string=w3019) -> (number=w3003:dbl)  [unwired: 3 in, 1 out]
                      n1488 = Fract/Exp String To Number(string=w3018) -> (number=w3017:dbl)  [unwired: 3 in, 1 out]
                      n1489 = Fract/Exp String To Number(string=w3015) -> (number=w3012:dbl)  [unwired: 3 in, 1 out]
                      n1490 = Divide(x=w3017, y=100.0) -> (x/y=w3004:dbl)
                      n1491 = Multiply(x=w3004, y=w3003) -> (x*y=w3002:dbl)
                      n1492 = Add(x=w3003, y=w3002) -> (x+y=w3014:dbl)
                      n1493 = Subtract(x=w3003, y=w3002) -> (x-y=w3013:dbl)
                      n1494 = In Range and Coerce(upper limit=w3014, x=w3012, lower limit=w3013) -> (In Range?=w3011:bool)  [unwired: 1 out]
                      n1495 = Select(t="P", s=w3011, f="F") -> (s? t:f=w3006:string)
                      n1496 = Replace Array Subset(array=w3022, new element #1=w3015, index (row) #1=w3008, index (col) #1=w3023, new element #2=w3006, index (row) #2=w3008, index (col) #2=5 ("disabled index (col)")) -> (w3005:string[][])
                    }
                    frame 23 {
                      w3042 = 3  # tol
                      w3043 = 2  # res
                      w3045 = 4  # meas
                      # "fill the P/F\ncol"
                      # "fill the meas col"
                      # "check to see\npass or fail"
                      # "pull out resistor\nvalue and tolerance\nto find limits"
                      n1497 = Index Array(array=w3044, index (row) #1=w3030, index (col) #1=w3043, index (row) #2=w3030, index (col) #2=w3042) -> (element #1=w3041:string, element #2=w3040:string)
                      n1498 = Fract/Exp String To Number(string=w3041) -> (number=w3025:dbl)  [unwired: 3 in, 1 out]
                      n1499 = Fract/Exp String To Number(string=w3040) -> (number=w3039:dbl)  [unwired: 3 in, 1 out]
                      n1500 = Fract/Exp String To Number(string=w3037) -> (number=w3034:dbl)  [unwired: 3 in, 1 out]
                      n1501 = Divide(x=w3039, y=100.0) -> (x/y=w3026:dbl)
                      n1502 = Multiply(x=w3026, y=w3025) -> (x*y=w3024:dbl)
                      n1503 = Add(x=w3025, y=w3024) -> (x+y=w3036:dbl)
                      n1504 = Subtract(x=w3025, y=w3024) -> (x-y=w3035:dbl)
                      n1505 = In Range and Coerce(upper limit=w3036, x=w3034, lower limit=w3035) -> (In Range?=w3033:bool)  [unwired: 1 out]
                      n1506 = Select(t="P", s=w3033, f="F") -> (s? t:f=w3028:string)
                      n1507 = Replace Array Subset(array=w3044, new element #1=w3037, index (row) #1=w3030, index (col) #1=w3045, new element #2=w3028, index (row) #2=w3030, index (col) #2=5 ("disabled index (col)")) -> (w3027:string[][])
                    }
                    frame 24 {
                      w3064 = 3  # tol
                      w3065 = 2  # res
                      w3067 = 4  # meas
                      # "fill the P/F\ncol"
                      # "fill the meas col"
                      # "check to see\npass or fail"
                      # "pull out resistor\nvalue and tolerance\nto find limits"
                      n1508 = Index Array(array=w3066, index (row) #1=w3052, index (col) #1=w3065, index (row) #2=w3052, index (col) #2=w3064) -> (element #1=w3063:string, element #2=w3062:string)
                      n1509 = Fract/Exp String To Number(string=w3063) -> (number=w3047:dbl)  [unwired: 3 in, 1 out]
                      n1510 = Fract/Exp String To Number(string=w3062) -> (number=w3061:dbl)  [unwired: 3 in, 1 out]
                      n1511 = Fract/Exp String To Number(string=w3059) -> (number=w3056:dbl)  [unwired: 3 in, 1 out]
                      n1512 = Divide(x=w3061, y=100.0) -> (x/y=w3048:dbl)
                      n1513 = Multiply(x=w3048, y=w3047) -> (x*y=w3046:dbl)
                      n1514 = Add(x=w3047, y=w3046) -> (x+y=w3058:dbl)
                      n1515 = Subtract(x=w3047, y=w3046) -> (x-y=w3057:dbl)
                      n1516 = In Range and Coerce(upper limit=w3058, x=w3056, lower limit=w3057) -> (In Range?=w3055:bool)  [unwired: 1 out]
                      n1517 = Select(t="P", s=w3055, f="F") -> (s? t:f=w3050:string)
                      n1518 = Replace Array Subset(array=w3066, new element #1=w3059, index (row) #1=w3052, index (col) #1=w3067, new element #2=w3050, index (row) #2=w3052, index (col) #2=5 ("disabled index (col)")) -> (w3049:string[][])
                    }
                    frame 25 {
                      w3086 = 3  # tol
                      w3087 = 2  # res
                      w3089 = 4  # meas
                      # "fill the P/F\ncol"
                      # "fill the meas col"
                      # "check to see\npass or fail"
                      # "pull out resistor\nvalue and tolerance\nto find limits"
                      n1519 = Index Array(array=w3088, index (row) #1=w3074, index (col) #1=w3087, index (row) #2=w3074, index (col) #2=w3086) -> (element #1=w3085:string, element #2=w3084:string)
                      n1520 = Fract/Exp String To Number(string=w3085) -> (number=w3069:dbl)  [unwired: 3 in, 1 out]
                      n1521 = Fract/Exp String To Number(string=w3084) -> (number=w3083:dbl)  [unwired: 3 in, 1 out]
                      n1522 = Fract/Exp String To Number(string=w3081) -> (number=w3078:dbl)  [unwired: 3 in, 1 out]
                      n1523 = Divide(x=w3083, y=100.0) -> (x/y=w3070:dbl)
                      n1524 = Multiply(x=w3070, y=w3069) -> (x*y=w3068:dbl)
                      n1525 = Add(x=w3069, y=w3068) -> (x+y=w3080:dbl)
                      n1526 = Subtract(x=w3069, y=w3068) -> (x-y=w3079:dbl)
                      n1527 = In Range and Coerce(upper limit=w3080, x=w3078, lower limit=w3079) -> (In Range?=w3077:bool)  [unwired: 1 out]
                      n1528 = Select(t="P", s=w3077, f="F") -> (s? t:f=w3072:string)
                      n1529 = Replace Array Subset(array=w3088, new element #1=w3081, index (row) #1=w3074, index (col) #1=w3089, new element #2=w3072, index (row) #2=w3074, index (col) #2=5 ("disabled index (col)")) -> (w3071:string[][])
                    }
                    frame 26 {
                      w3108 = 3  # tol
                      w3109 = 2  # res
                      w3111 = 4  # meas
                      # "fill the P/F\ncol"
                      # "fill the meas col"
                      # "check to see\npass or fail"
                      # "pull out resistor\nvalue and tolerance\nto find limits"
                      n1530 = Index Array(array=w3110, index (row) #1=w3096, index (col) #1=w3109, index (row) #2=w3096, index (col) #2=w3108) -> (element #1=w3107:string, element #2=w3106:string)
                      n1531 = Fract/Exp String To Number(string=w3107) -> (number=w3091:dbl)  [unwired: 3 in, 1 out]
                      n1532 = Fract/Exp String To Number(string=w3106) -> (number=w3105:dbl)  [unwired: 3 in, 1 out]
                      n1533 = Fract/Exp String To Number(string=w3103) -> (number=w3100:dbl)  [unwired: 3 in, 1 out]
                      n1534 = Divide(x=w3105, y=100.0) -> (x/y=w3092:dbl)
                      n1535 = Multiply(x=w3092, y=w3091) -> (x*y=w3090:dbl)
                      n1536 = Add(x=w3091, y=w3090) -> (x+y=w3102:dbl)
                      n1537 = Subtract(x=w3091, y=w3090) -> (x-y=w3101:dbl)
                      n1538 = In Range and Coerce(upper limit=w3102, x=w3100, lower limit=w3101) -> (In Range?=w3099:bool)  [unwired: 1 out]
                      n1539 = Select(t="P", s=w3099, f="F") -> (s? t:f=w3094:string)
                      n1540 = Replace Array Subset(array=w3110, new element #1=w3103, index (row) #1=w3096, index (col) #1=w3111, new element #2=w3094, index (row) #2=w3096, index (col) #2=5 ("disabled index (col)")) -> (w3093:string[][])
                    }
                    frame 27 {
                      w3130 = 3  # tol
                      w3131 = 2  # res
                      w3133 = 4  # meas
                      # "fill the P/F\ncol"
                      # "fill the meas col"
                      # "check to see\npass or fail"
                      # "pull out resistor\nvalue and tolerance\nto find limits"
                      n1541 = Index Array(array=w3132, index (row) #1=w3118, index (col) #1=w3131, index (row) #2=w3118, index (col) #2=w3130) -> (element #1=w3129:string, element #2=w3128:string)
                      n1542 = Fract/Exp String To Number(string=w3129) -> (number=w3113:dbl)  [unwired: 3 in, 1 out]
                      n1543 = Fract/Exp String To Number(string=w3128) -> (number=w3127:dbl)  [unwired: 3 in, 1 out]
                      n1544 = Fract/Exp String To Number(string=w3125) -> (number=w3122:dbl)  [unwired: 3 in, 1 out]
                      n1545 = Divide(x=w3127, y=100.0) -> (x/y=w3114:dbl)
                      n1546 = Multiply(x=w3114, y=w3113) -> (x*y=w3112:dbl)
                      n1547 = Add(x=w3113, y=w3112) -> (x+y=w3124:dbl)
                      n1548 = Subtract(x=w3113, y=w3112) -> (x-y=w3123:dbl)
                      n1549 = In Range and Coerce(upper limit=w3124, x=w3122, lower limit=w3123) -> (In Range?=w3121:bool)  [unwired: 1 out]
                      n1550 = Select(t="P", s=w3121, f="F") -> (s? t:f=w3116:string)
                      n1551 = Replace Array Subset(array=w3132, new element #1=w3125, index (row) #1=w3118, index (col) #1=w3133, new element #2=w3116, index (row) #2=w3118, index (col) #2=5 ("disabled index (col)")) -> (w3115:string[][])
                    }
                    frame 28 {
                      w3152 = 3  # tol
                      w3153 = 2  # res
                      w3155 = 4  # meas
                      # "fill the P/F\ncol"
                      # "fill the meas col"
                      # "check to see\npass or fail"
                      # "pull out resistor\nvalue and tolerance\nto find limits"
                      n1552 = Index Array(array=w3154, index (row) #1=w3140, index (col) #1=w3153, index (row) #2=w3140, index (col) #2=w3152) -> (element #1=w3151:string, element #2=w3150:string)
                      n1553 = Fract/Exp String To Number(string=w3151) -> (number=w3135:dbl)  [unwired: 3 in, 1 out]
                      n1554 = Fract/Exp String To Number(string=w3150) -> (number=w3149:dbl)  [unwired: 3 in, 1 out]
                      n1555 = Fract/Exp String To Number(string=w3147) -> (number=w3144:dbl)  [unwired: 3 in, 1 out]
                      n1556 = Divide(x=w3149, y=100.0) -> (x/y=w3136:dbl)
                      n1557 = Multiply(x=w3136, y=w3135) -> (x*y=w3134:dbl)
                      n1558 = Add(x=w3135, y=w3134) -> (x+y=w3146:dbl)
                      n1559 = Subtract(x=w3135, y=w3134) -> (x-y=w3145:dbl)
                      n1560 = In Range and Coerce(upper limit=w3146, x=w3144, lower limit=w3145) -> (In Range?=w3143:bool)  [unwired: 1 out]
                      n1561 = Select(t="P", s=w3143, f="F") -> (s? t:f=w3138:string)
                      n1562 = Replace Array Subset(array=w3154, new element #1=w3147, index (row) #1=w3140, index (col) #1=w3155, new element #2=w3138, index (row) #2=w3140, index (col) #2=5 ("disabled index (col)")) -> (w3137:string[][])
                    }
                    frame 29 {
                      w3174 = 3  # tol
                      w3175 = 2  # res
                      w3177 = 4  # meas
                      # "fill the P/F\ncol"
                      # "fill the meas col"
                      # "check to see\npass or fail"
                      # "pull out resistor\nvalue and tolerance\nto find limits"
                      n1563 = Index Array(array=w3176, index (row) #1=w3162, index (col) #1=w3175, index (row) #2=w3162, index (col) #2=w3174) -> (element #1=w3173:string, element #2=w3172:string)
                      n1564 = Fract/Exp String To Number(string=w3173) -> (number=w3157:dbl)  [unwired: 3 in, 1 out]
                      n1565 = Fract/Exp String To Number(string=w3172) -> (number=w3171:dbl)  [unwired: 3 in, 1 out]
                      n1566 = Fract/Exp String To Number(string=w3169) -> (number=w3166:dbl)  [unwired: 3 in, 1 out]
                      n1567 = Divide(x=w3171, y=100.0) -> (x/y=w3158:dbl)
                      n1568 = Multiply(x=w3158, y=w3157) -> (x*y=w3156:dbl)
                      n1569 = Add(x=w3157, y=w3156) -> (x+y=w3168:dbl)
                      n1570 = Subtract(x=w3157, y=w3156) -> (x-y=w3167:dbl)
                      n1571 = In Range and Coerce(upper limit=w3168, x=w3166, lower limit=w3167) -> (In Range?=w3165:bool)  [unwired: 1 out]
                      n1572 = Select(t="P", s=w3165, f="F") -> (s? t:f=w3160:string)
                      n1573 = Replace Array Subset(array=w3176, new element #1=w3169, index (row) #1=w3162, index (col) #1=w3177, new element #2=w3160, index (row) #2=w3162, index (col) #2=5 ("disabled index (col)")) -> (w3159:string[][])
                    }
                    frame 30 {
                      w3196 = 3  # tol
                      w3197 = 2  # res
                      w3199 = 4  # meas
                      # "fill the P/F\ncol"
                      # "fill the meas col"
                      # "check to see\npass or fail"
                      # "pull out resistor\nvalue and tolerance\nto find limits"
                      n1574 = Index Array(array=w3198, index (row) #1=w3184, index (col) #1=w3197, index (row) #2=w3184, index (col) #2=w3196) -> (element #1=w3195:string, element #2=w3194:string)
                      n1575 = Fract/Exp String To Number(string=w3195) -> (number=w3179:dbl)  [unwired: 3 in, 1 out]
                      n1576 = Fract/Exp String To Number(string=w3194) -> (number=w3193:dbl)  [unwired: 3 in, 1 out]
                      n1577 = Fract/Exp String To Number(string=w3191) -> (number=w3188:dbl)  [unwired: 3 in, 1 out]
                      n1578 = Divide(x=w3193, y=100.0) -> (x/y=w3180:dbl)
                      n1579 = Multiply(x=w3180, y=w3179) -> (x*y=w3178:dbl)
                      n1580 = Add(x=w3179, y=w3178) -> (x+y=w3190:dbl)
                      n1581 = Subtract(x=w3179, y=w3178) -> (x-y=w3189:dbl)
                      n1582 = In Range and Coerce(upper limit=w3190, x=w3188, lower limit=w3189) -> (In Range?=w3187:bool)  [unwired: 1 out]
                      n1583 = Select(t="P", s=w3187, f="F") -> (s? t:f=w3182:string)
                      n1584 = Replace Array Subset(array=w3198, new element #1=w3191, index (row) #1=w3184, index (col) #1=w3199, new element #2=w3182, index (row) #2=w3184, index (col) #2=5 ("disabled index (col)")) -> (w3181:string[][])
                    }
                    frame 31 {
                      w3218 = 3  # tol
                      w3219 = 2  # res
                      w3221 = 4  # meas
                      # "fill the P/F\ncol"
                      # "fill the meas col"
                      # "check to see\npass or fail"
                      # "pull out resistor\nvalue and tolerance\nto find limits"
                      n1585 = Index Array(array=w3220, index (row) #1=w3206, index (col) #1=w3219, index (row) #2=w3206, index (col) #2=w3218) -> (element #1=w3217:string, element #2=w3216:string)
                      n1586 = Fract/Exp String To Number(string=w3217) -> (number=w3201:dbl)  [unwired: 3 in, 1 out]
                      n1587 = Fract/Exp String To Number(string=w3216) -> (number=w3215:dbl)  [unwired: 3 in, 1 out]
                      n1588 = Fract/Exp String To Number(string=w3213) -> (number=w3210:dbl)  [unwired: 3 in, 1 out]
                      n1589 = Divide(x=w3215, y=100.0) -> (x/y=w3202:dbl)
                      n1590 = Multiply(x=w3202, y=w3201) -> (x*y=w3200:dbl)
                      n1591 = Add(x=w3201, y=w3200) -> (x+y=w3212:dbl)
                      n1592 = Subtract(x=w3201, y=w3200) -> (x-y=w3211:dbl)
                      n1593 = In Range and Coerce(upper limit=w3212, x=w3210, lower limit=w3211) -> (In Range?=w3209:bool)  [unwired: 1 out]
                      n1594 = Select(t="P", s=w3209, f="F") -> (s? t:f=w3204:string)
                      n1595 = Replace Array Subset(array=w3220, new element #1=w3213, index (row) #1=w3206, index (col) #1=w3221, new element #2=w3204, index (row) #2=w3206, index (col) #2=5 ("disabled index (col)")) -> (w3203:string[][])
                    }
                    frame 32 {
                      w3240 = 3  # tol
                      w3241 = 2  # res
                      w3243 = 4  # meas
                      # "fill the P/F\ncol"
                      # "fill the meas col"
                      # "check to see\npass or fail"
                      # "pull out resistor\nvalue and tolerance\nto find limits"
                      n1596 = Index Array(array=w3242, index (row) #1=w3228, index (col) #1=w3241, index (row) #2=w3228, index (col) #2=w3240) -> (element #1=w3239:string, element #2=w3238:string)
                      n1597 = Fract/Exp String To Number(string=w3239) -> (number=w3223:dbl)  [unwired: 3 in, 1 out]
                      n1598 = Fract/Exp String To Number(string=w3238) -> (number=w3237:dbl)  [unwired: 3 in, 1 out]
                      n1599 = Fract/Exp String To Number(string=w3235) -> (number=w3232:dbl)  [unwired: 3 in, 1 out]
                      n1600 = Divide(x=w3237, y=100.0) -> (x/y=w3224:dbl)
                      n1601 = Multiply(x=w3224, y=w3223) -> (x*y=w3222:dbl)
                      n1602 = Add(x=w3223, y=w3222) -> (x+y=w3234:dbl)
                      n1603 = Subtract(x=w3223, y=w3222) -> (x-y=w3233:dbl)
                      n1604 = In Range and Coerce(upper limit=w3234, x=w3232, lower limit=w3233) -> (In Range?=w3231:bool)  [unwired: 1 out]
                      n1605 = Select(t="P", s=w3231, f="F") -> (s? t:f=w3226:string)
                      n1606 = Replace Array Subset(array=w3242, new element #1=w3235, index (row) #1=w3228, index (col) #1=w3243, new element #2=w3226, index (row) #2=w3228, index (col) #2=5 ("disabled index (col)")) -> (w3225:string[][])
                    }
                    frame 33 {
                      w3262 = 3  # tol
                      w3263 = 2  # res
                      w3265 = 4  # meas
                      # "fill the P/F\ncol"
                      # "fill the meas col"
                      # "check to see\npass or fail"
                      # "pull out resistor\nvalue and tolerance\nto find limits"
                      n1607 = Index Array(array=w3264, index (row) #1=w3250, index (col) #1=w3263, index (row) #2=w3250, index (col) #2=w3262) -> (element #1=w3261:string, element #2=w3260:string)
                      n1608 = Fract/Exp String To Number(string=w3261) -> (number=w3245:dbl)  [unwired: 3 in, 1 out]
                      n1609 = Fract/Exp String To Number(string=w3260) -> (number=w3259:dbl)  [unwired: 3 in, 1 out]
                      n1610 = Fract/Exp String To Number(string=w3257) -> (number=w3254:dbl)  [unwired: 3 in, 1 out]
                      n1611 = Divide(x=w3259, y=100.0) -> (x/y=w3246:dbl)
                      n1612 = Multiply(x=w3246, y=w3245) -> (x*y=w3244:dbl)
                      n1613 = Add(x=w3245, y=w3244) -> (x+y=w3256:dbl)
                      n1614 = Subtract(x=w3245, y=w3244) -> (x-y=w3255:dbl)
                      n1615 = In Range and Coerce(upper limit=w3256, x=w3254, lower limit=w3255) -> (In Range?=w3253:bool)  [unwired: 1 out]
                      n1616 = Select(t="P", s=w3253, f="F") -> (s? t:f=w3248:string)
                      n1617 = Replace Array Subset(array=w3264, new element #1=w3257, index (row) #1=w3250, index (col) #1=w3265, new element #2=w3248, index (row) #2=w3250, index (col) #2=5 ("disabled index (col)")) -> (w3247:string[][])
                    }
                    frame 34 {
                      w3284 = 3  # tol
                      w3285 = 2  # res
                      w3287 = 4  # meas
                      # "fill the P/F\ncol"
                      # "fill the meas col"
                      # "check to see\npass or fail"
                      # "pull out resistor\nvalue and tolerance\nto find limits"
                      n1618 = Index Array(array=w3286, index (row) #1=w3272, index (col) #1=w3285, index (row) #2=w3272, index (col) #2=w3284) -> (element #1=w3283:string, element #2=w3282:string)
                      n1619 = Fract/Exp String To Number(string=w3283) -> (number=w3267:dbl)  [unwired: 3 in, 1 out]
                      n1620 = Fract/Exp String To Number(string=w3282) -> (number=w3281:dbl)  [unwired: 3 in, 1 out]
                      n1621 = Fract/Exp String To Number(string=w3279) -> (number=w3276:dbl)  [unwired: 3 in, 1 out]
                      n1622 = Divide(x=w3281, y=100.0) -> (x/y=w3268:dbl)
                      n1623 = Multiply(x=w3268, y=w3267) -> (x*y=w3266:dbl)
                      n1624 = Add(x=w3267, y=w3266) -> (x+y=w3278:dbl)
                      n1625 = Subtract(x=w3267, y=w3266) -> (x-y=w3277:dbl)
                      n1626 = In Range and Coerce(upper limit=w3278, x=w3276, lower limit=w3277) -> (In Range?=w3275:bool)  [unwired: 1 out]
                      n1627 = Select(t="P", s=w3275, f="F") -> (s? t:f=w3270:string)
                      n1628 = Replace Array Subset(array=w3286, new element #1=w3279, index (row) #1=w3272, index (col) #1=w3287, new element #2=w3270, index (row) #2=w3272, index (col) #2=5 ("disabled index (col)")) -> (w3269:string[][])
                    }
                  }
                }
              }
            }
            n1629 = Bundle By Name(cluster=w945, "state"=state_cntrl."fin_test_qry") -> (w946:T6)
            n1630 = local write "res_table"(w931) -> ()
            n1631 = Bundle By Name(cluster=w933, "res_table_text"=w931) -> (w932:T7)
            n1632 = Enqueue Element(queue=w947, element=w946) -> ()  [unwired: 2 in, 3 out]
          }
          frame "fin_test_qry" {
            # "Check to see if we are done with all\nthe ranges."
            n1633 = Unbundle By Name(w3292) -> ("ch_list_set_cnt"=w3293:i32)
            n1634 = Equal To 0?(x=w3293) -> (x = 0?=w3291:bool)
            n1635 = Select(t=state_cntrl."initialize" ("state"), s=w3291, f=state_cntrl."chk_100_list_flg" ("state")) -> (s? t:f=w3288:T1)
            n1636 = Bundle By Name(cluster=w3294, "state"=w3288) -> (w3295:T6)
            n1637 = Enqueue Element(queue=w3296, element=w3295) -> ()  [unwired: 2 in, 3 out]
          }
          frame "place_res_in_range" {
            n1638 = Unbundle By Name(w3299) -> ("res_col"=w3301:dbl[], "res_row_cnt"=w3300:i32)  [unwired: 1 out]
            n1639 = Bundle By Name(cluster=w3303, "state"=state_cntrl."place_res_in_range") -> (w3306:T6)
            n1640 = Increment(x=w3300) -> (x+1=w3298:i32)
            n1641 = Enqueue Element(queue=w3307, element=w3306) -> ()  [unwired: 2 in, 3 out]
            n1642 = Index Array(array=w3301, index=w3300) -> (element=w3302:dbl)
            n1643 = Less?(x=w3302, y=100.0) -> ()  [unwired: 1 out]
            n1644 = Bundle By Name(cluster=w3299, "res_row_cnt"=w3298) -> (w3297:T7)
          }
        }
      }
      frame Error {
        # "Return true in any case that should stop the loop."
      }
    }
  }
  n1645 = Release Queue(queue=w4, error in (no error)=w11) -> (error out=w7:errorcluster)  [unwired: 1 in, 2 out]
  n1646 = call <instrlib>:"AG34980A Close.vi"("VISA resource name"=w8, "error in (no error)"=w7) -> ()  [unwired: 13 in, 1 out]
